vi "Cascade front panel.vi"() -> ()   [LabVIEW 2016]
uses:
  sdi_12/SDI-12/Sonde Vertical Graph.ctl
  controls/Vertical Chart.ctl
  sdi_12/Groundwater header.ctl
  controls/MCC DAQ Setup.ctl
  controls/Aux Sensor.ctl
  KPRO_2016 subvis/Control 2.ctl
  KPRO_2016 subvis/Graph Controls 2.ctl
  KPRO_2016 subvis/Ik control.ctl
  controls/MCC DAQ Readings.ctl
  controls/Kpro pressure measurement cluster.ctl
  controls/Kpro hydraulic measurement cluster.ctl
  activeXtest/activeXtest 2015 Folder/sonde cluster from excel.ctl
  sdi_12/Sonde Value Percent Tol.ctl
  activeXtest/activeXtest 2015 Folder/sample data row cluster.ctl
  activeXtest/activeXtest 2015 Folder/sonde cluster.ctl
  KPRO_2016 subvis/Sensor Physical Measurements.ctl
  KPRO_2016 subvis/SS Control 7.ctl
  <vilib>/Utility/NIReport.llb/NI_report.lvclass
  controls/Action Control 1.ctl
  <extravilib>/ChannelInstances/One Element Stream-t'Action Control 1.ctl'/Instantiate.vi
  <extravilib>/ChannelInstances/One Element Stream-t'Action Control 1.ctl'/Endpoint.vi
  KPRO_2016 subvis/Kpro Globals.vi
  <vilib>/Utility/file.llb/Write Delimited Spreadsheet (string).vi
  <userlib>/_OpenG.lib/file/file.llb/Strip Path - Traditional__ogtk.vi
  <userlib>/_OpenG.lib/file/file.llb/Build Path - Traditional__ogtk.vi
  <vilib>/Utility/file.llb/Write Delimited Spreadsheet (DBL).vi
  <userlib>/_OpenG.lib/file/file.llb/Strip Path Extension - Path__ogtk.vi
  <userlib>/_OpenG.lib/file/file.llb/Convert File Extension (String)__ogtk.vi
  <vilib>/ULx/Create Channel.llb/ULx Create Channel (AI-Voltage-Basic).vi
  KPRO_2016 subvis/Global_SIM_switch.vi
  C:/Program Files (x86)/National Instruments/LabVIEW 2016/vi.lib/ULx/ULx_LV.dll
  Program Files (x86)/National Instruments/LabVIEW 2016/vi.lib/ULx/ULx_LV.dll
  <vilib>/Utility/config.llb/NI_LVConfig.lvlib
  <extravilib>/ChannelInstances/One Element Stream-t'Action Control 1.ctl'.lvlib
panel:
  in  "Open Excel Files":bool
  in  "Input Variables and Slopes 2":T1={"Total Volume"=0.0, "String Pot Slope"=1.6619999408721924, "Flow Slope"=39.040000915527344, "Up Hole Pressure Slope"=48.27000045776367, "Depth to Water Table"=-0.0, "Atmospheric Pressure"=32.22022530555725, "Reservoir Pressure"=-0.004827000045779073, "Height of Sample Box"=0.0, "DH Pressure Trans Slope"=42.0, "DH Pressure Offset"=0.0, "Up Hole  Pressure Offset"=0.0, "Aux 1 Slope"=1.0, "Aux 2 Slope"=1.0, "Aux 3 Slope"=1.0} {"Aux 3 Slope" format="%.2f"; "Aux 2 Slope" format="%.2f"; "Aux 1 Slope" format="%.2f"; "Up Hole  Pressure Offset" format="%.2f"; "DH Pressure Offset" format="%.2f"; "DH Pressure Trans Slope" format="%.2f"; "Height of Sample Box" format="%.2f"; "Reservoir Pressure" format="%.2f"; "Atmospheric Pressure" format="%.2f"; "Depth to Water Table" format="%.2f"; "Up Hole Pressure Slope" format="%.2f"; "Flow Slope" format="%.2f"; "String Pot Slope" format="%.2f"; "Total Volume" format="%.2f"}
  out "Select Worksheet Index":i32
  out "Number of Sample Sheets":i32
  out "NI_report out":refnum<class "NI_report.lvclass">
  out "Sonde OK":bool
  out "DAQ On":bool
  in  "Finish Tests 2":bool
  out "output cluster":T2 caption="Cluster" {"Salinity" format="%_3g"; "Temp\ndeg C" format="%_2g"; "ORP" format="%_4g"; "pH" format="%_4g"; "Dissolved\nOxygen mg/L" format="%_3g"; "Specific\nCond (mS)" format="%_4g"; "Cumulative\nVolume (ml)" format="%#_4g"}
  out "Serial Number/MISC":string
  in  "Depth mode":bool caption="Use \nIncrement"
  in  "Sample Sheet Data Row Cluster 2":T3={"Head\nPressure"=0.0, "Depth"=0.0, "comment string"="", "Sonde Data Cluster"={"Cumulative\nVolume (ml)"=100.0, "Specific\nCond (mS)"=2.0, "Dissolved\nOxygen mg/L"=3.0, "pH"=4.0, "ORP"=5.0, "Temp\ndeg C"=26.0, "Salinity"=7.0}, "Aux1"=0.0, "Aux2"=0.0, "Aux3"=0.0} {"Sonde Data Cluster"."Salinity" format="%_3g"; "Sonde Data Cluster"."Temp\ndeg C" format="%_2g"; "Sonde Data Cluster"."ORP" format="%_4g"; "Sonde Data Cluster"."pH" format="%_4g"; "Sonde Data Cluster"."Dissolved\nOxygen mg/L" format="%_4g"; "Sonde Data Cluster"."Specific\nCond (mS)" format="%_4g"; "Sonde Data Cluster"."Cumulative\nVolume (ml)" format="%#_4g"; "Depth" format="%#.3g"; "Head\nPressure" format="%#.4g"}
  out "subarray":string[][](array[string])
  out "Initialization":i32
  in  "Increment Depth":bool
  in  "Finish Tests":bool
  in  "Start KPRO":bool
  in  "Record Continuous Samples":bool
  out "Current Time (s)":dbl
  in  "stop":bool
  in  "Write Data to Spreadsheet":bool
  in  "Sample Not Collected":bool
  in  "Record Single Sample":bool
  in  "Tab Control":T4(tab)
  out "12V Voltage Monitor":dbl format="%_3f"
  out "Found Quanta Sonde Com Port":refnum<visa-resource-name>
  in  "Temporary Data Files Directory":path=path "C:/Cascade/Data/Output Files"
  in  "Data File Directory":path=path "C:/Cascade/Data/Excel Reports"
  out "Quanta Sonde found?":bool
  in  "template file path":path=path "C:/Cascade/templates/Groundwater Profiling Log_empty_labview_template.xlsx"
  in  "Config File Path":path=path "C:/Cascade/Data/config files/DAQ Setup Config.ini"
  in  "Read Configuration File?":bool
  out "H-4191 Adapter found":bool
  in  "Save Configuration File?":bool
  out "Sonde Communication Error Out":errorcluster
  in  "Search for Comm Ports?":bool=TRUE
  in  "USB Serial Port Manual Entry":refnum<visa-resource-name>="COM13"
  in  "Sonde Parameters \nTolerance Limits":T5 {"Salinity %" format="%_2f%%"; "Temp %" format="%_2f%%"; "ORP %" format="%_2f%%"; "pH %" format="%_2f%%"; "DO %" format="%_2f%%"; "SC %" format="%_2f%%"}
  in  "Sonde Parameters \nInitial Values":T6 {"Salinity Initial" format="%_2f"; "Temp Initial" format="%_2f"; "ORP  Initial" format="%_2f"; "pH Initial" format="%_2f"; "DO Initial" format="%_2f"; "SC Initial" format="%_2f"}
  in  "Header path":path=path "C:/Cascade/templates/Fields for Excel sheets.xlsx"
  out "Sensor  Real \nMeasurements":T7 {"9V Monitor" format="%#.3g"; "Aux 3" format="%#.3g"; "Aux 2" format="%#.3g"; "Aux 1" format="%#.3g"; "String Pot" format="%#.3g"; "Top String Pot" format="%#_4g"; "Downhole Pressure" format="%#_4g"; "Flow" format="%#_4g"; "Uphole Pressure" format="%#_4g"}
  in  "MCC USB-DAQ Setup":T8={"Device Name in InstaCal"="Dev0", "Omega Pressure Sensor"={"DAQ Channel"=2.0, "Output Voltage Range"=1, "Enabled"=TRUE, "Description"="Uphole Pressure"}, "McMillian 102 Flowmeter"={"DAQ Channel"=11.0, "Output Voltage Range"=0, "Enabled"=TRUE, "Description"="Flow"}, "DHT Pressure Sensor"={"DAQ Channel"=3.0, "Output Voltage Range"=1, "Enabled"=TRUE, "Description"="Downhole Pressure"}, "Top String Pot"={"DAQ Channel"=0.0, "Output Voltage Range"=0, "Enabled"=TRUE, "Description"="Top String Pot"}, "String Pot Signal"={"DAQ Channel"=1.0, "Output Voltage Range"=0, "Enabled"=TRUE, "Description"="String Pot"}, "Aux Sensor 1"={"DAQ Channel"=5.0, "Output Voltage Range"=1, "Enabled"=TRUE, "Description"="Aux 1"}, "Aux Sensor 2"={"DAQ Channel"=6.0, "Output Voltage Range"=1, "Enabled"=TRUE, "Description"="Aux 2"}, "Aux Sensor 3"={"DAQ Channel"=7.0, "Output Voltage Range"=1, "Enabled"=TRUE, "Description"="Aux 3"}, "Voltage Monitor"={"DAQ Channel"=8.0, "Output Voltage Range"=0, "Enabled"=TRUE, "Description"="9V Monitor"}} {"Voltage Monitor"."Output Voltage Range" items=["+/-10 V Range", "+/-5 V Range", "+/-2.5V Range", "+/-1.25 V Range", "+/-0.625 V Range", "+/-0.3125 V Range", "+/-0.1562V Range", "+/-0.078125 V Range"]; "Aux Sensor 3"."Output Voltage Range" items=["+/-10 V Range", "+/-5 V Range", "+/-2.5V Range", "+/-1.25 V Range", "+/-0.625 V Range", "+/-0.3125 V Range", "+/-0.1562V Range", "+/-0.078125 V Range"]; "Aux Sensor 2"."Output Voltage Range" items=["+/-10 V Range", "+/-5 V Range", "+/-2.5V Range", "+/-1.25 V Range", "+/-0.625 V Range", "+/-0.3125 V Range", "+/-0.1562V Range", "+/-0.078125 V Range"]; "Aux Sensor 1"."Output Voltage Range" items=["+/-10 V Range", "+/-5 V Range", "+/-2.5V Range", "+/-1.25 V Range", "+/-0.625 V Range", "+/-0.3125 V Range", "+/-0.1562V Range", "+/-0.078125 V Range"]; "String Pot Signal"."Output Voltage Range" items=["+/-10 V Range", "+/-5 V Range", "+/-2.5V Range", "+/-1.25 V Range", "+/-0.625 V Range", "+/-0.3125 V Range", "+/-0.1562V Range", "+/-0.078125 V Range"]; "Top String Pot"."Output Voltage Range" items=["+/-10 V Range", "+/-5 V Range", "+/-2.5V Range", "+/-1.25 V Range", "+/-0.625 V Range", "+/-0.3125 V Range", "+/-0.1562V Range", "+/-0.078125 V Range"]; "DHT Pressure Sensor"."Output Voltage Range" items=["+/-10 V Range", "+/-5 V Range", "+/-2.5V Range", "+/-1.25 V Range", "+/-0.625 V Range", "+/-0.3125 V Range", "+/-0.1562V Range", "+/-0.078125 V Range"]; "McMillian 102 Flowmeter"."Output Voltage Range" items=["+/-10 V Range", "+/-5 V Range", "+/-2.5V Range", "+/-1.25 V Range", "+/-0.625 V Range", "+/-0.3125 V Range", "+/-0.1562V Range", "+/-0.078125 V Range"]; "Omega Pressure Sensor"."Output Voltage Range" items=["+/-10 V Range", "+/-5 V Range", "+/-2.5V Range", "+/-1.25 V Range", "+/-0.625 V Range", "+/-0.3125 V Range", "+/-0.1562V Range", "+/-0.078125 V Range"]}
  out "Rate":dbl=1000.0 caption="Sample Rate (Hz)"
  out "Number \nof Channels":u16
  in  "Channel \nData Rate S/s":dbl=3720.0 format="%#_13g"
  out "Descriptions":string[](array[string])
  out "Raw Voltages":dbl[](array[numeric])
  out "9V Voltage Monitor":dbl format="%#_3g"
  in  "Record DAQ Raw Voltages":bool
  out "Sensor Voltage Cluster":T10 {"9V Monitor" format="%#.3g"; "Aux 3" format="%#_3g"; "Aux 2" format="%#.3g"; "Aux 1" format="%#.3g"; "String Pot" format="%#.3g"; "Top String Pot" format="%#_3g"; "Downhole Pressure" format="%#.3g"; "Flow" format="%#_3g"; "Uphole Pressure" format="%-#1.3g"}
  in  "Clear Groundwater Header Values":bool
  in  "Groundwater Header":T11
  in  "Excel report file path":path=path "C:/Cascade/Data/Excel Reports/Groundwater Profiling Log_ara1.xlsx"
  out "Data Setup Indicator":string
  in  "Start Initialization":bool
  in  "Input Variables and Slopes":T1={"Total Volume"=0.0, "String Pot Slope"=1.6619999408721924, "Flow Slope"=39.040000915527344, "Up Hole Pressure Slope"=48.27000045776367, "Depth to Water Table"=-0.0, "Atmospheric Pressure"=32.22022530555725, "Reservoir Pressure"=-0.004827000045779073, "Height of Sample Box"=0.0, "DH Pressure Trans Slope"=42.0, "DH Pressure Offset"=0.0, "Up Hole  Pressure Offset"=0.0, "Aux 1 Slope"=1.0, "Aux 2 Slope"=1.0, "Aux 3 Slope"=1.0} {"Aux 3 Slope" format="%.2f"; "Aux 2 Slope" format="%.2f"; "Aux 1 Slope" format="%.2f"; "Up Hole  Pressure Offset" format="%.2f"; "DH Pressure Offset" format="%.2f"; "DH Pressure Trans Slope" format="%.2f"; "Height of Sample Box" format="%.2f"; "Reservoir Pressure" format="%.2f"; "Atmospheric Pressure" format="%.2f"; "Depth to Water Table" format="%.2f"; "Up Hole Pressure Slope" format="%.2f"; "Flow Slope" format="%.2f"; "String Pot Slope" format="%.2f"; "Total Volume" format="%.2f"}
  out "Pressure Offset":dbl
  out "appended path":path
  out "Down hole Pressure Transducer CSV data  path 2":path
  in  "Static IK path":path=path "C:/Cascade/Data/Output Files/Static Ik.csv"
  in  "Slopes File Path":path=path "C:/Cascade/Data/Output Files/slopes.csv"
  out "Output File Path":path=path "C:/KPRO_2010/Output_files/Static Ik.txt"
  out "KPRO SessionOutput File Path":path=path "C:/KPRO_2010/Output_files/Static Ik.txt"
  in  "Slopes History File Path":path=path "C:/Cascade/Data/Output Files/slopes.csv"
  out "Sonde Recording Error file":path
  out "IK Recording Error file":path
  out "Sonde Output File Path":path=path "C:/KPRO_2010/Output_files/Static Ik.txt"
  out "KPRO Cumulative Output File Path":path=path "C:/Cascade/Data/Output Files/Output_files"
  in  "Update Sonde":bool
  out "Sonde Data Array":T12[](array[typedef]) {"Salinity"."%" format="%_2f%%"; "Salinity"."Value" format="%_4g"; "Temperature"."%" format="%_2f%%"; "Temperature"."Value" format="%_4g"; "ORP"."%" format="%_2f%%"; "ORP"."Value" format="%_4g"; "pH"."%" format="%_2f%%"; "pH"."Value" format="%_4g"; "Dissolved Oxygen"."%" format="%_2f%%"; "Dissolved Oxygen"."Value" format="%_4g"; "Sp. Conductance"."%" format="%_2f%%"; "Sp. Conductance"."Value" format="%_4g"; "Cumulative\nVolume" format="%#_4g"}
  out "Table Label":string="Data from Sample Sheet %d from Excel File"
  out "Sonde Data Display":T14
  out "Temperature":cluster{"Y":dbl[], "Y":dbl[]}[](graph)
  in  "Record  Sonde Reason":bool
  in  "Select Reasons to Record Data":u16(ring) items=["Per Client Request", "Timed Out", "Sample stopped flowing", "Equipment Issue"]
  out "Sonde Recording Failure Path":path
  out "Sonde IK Behavior Path":path
  out "Recording Reason Sonde array":string[][](array[string])
  out "IK Reason array":string[][](array[string])
  out "SC  Reference\nCalibrate Response":bool
  out "DO  Reference\nCalibrate Response":bool
  in  "Salinity \nReference":dbl
  out "Salinity  Reference\nCalibrate Response":bool
  out "ORP  Reference\nCalibrate Response":bool
  in  "SC \nReference":dbl
  in  "DO \nReference":dbl
  in  "ORP Reference":dbl
  in  "pH Reference":dbl
  in  "pH Zero":dbl
  in  "Record  SC Calibration":bool
  in  "Record DO Calibration":bool
  in  "Record Salinity Calibration":bool
  in  "Record ORP Calibration":bool
  in  "Record pH Calibration Reference":bool
  in  "Record pH Calibration Zero":bool
  out "pH Zero \nCalibrate Response":bool
  out "pH  Reference\nCalibrate Response":bool
  out "KPRO Finish\nIndicator":bool
  in  "Input Depths \nand Parameters Cluster":T16={"Flow"=0.21081600494384767, "Zeroed \nPressure"=74.74207969932556, "Ik"=0.003788962123473114, "Current Depth"=-100.6, "Feet of Stainless"=40, "Start Depth"=0.0, "Abs Start Depth"=0.0} {"Abs Start Depth" format="%.2f"; "Start Depth" format="%.2f"; "Current Depth" format="%.2f"; "Ik" format="%.2f"; "Zeroed \nPressure" format="%.2f"; "Flow" format="%.2f"}
  out "Zero Pressure\nIndicator":bool
  in  "Zero\nPressure":bool caption="Zero Pressure"
  in  "enable_IKMGS_file":bool
  in  "enable_slug_file":bool
  in  "enable_kpro_file":bool=TRUE
  in  "Simulate AD6B":bool
  out "KPRO Test\nIndicator":bool
  in  "Record DTW File":bool
  in  "Zero In-Line Pressure\n(F = leave as is)":bool=TRUE
  out "Current Session":sgl[][](array[numeric]) format="%.2f"
  in  "KPRO test report header":string[](array[string])=["Time(msecs)", "Uncorrected Depth", "Corrected Depth", "Drive_Rate", "Flow", "Feet_of Stainless", "Up Hole Pressure", "IK", "Corrected Pressure", "Atm Pressure", "Depth to water", "Height of box", "Res_Pressure", "Secs_since_1_JAN_1904", "Depth jumps more than 1_foot", "Down hole Pressure"]
  in  "Depth Cluster":T17
  out "Cumulative_data_from_file":sgl[][](array[numeric]) format="%.2f"
  in  "KPRO test report header 2":string[](array[string])=["Time(msecs)", "Uncorrected Depth", "Corrected Depth", "Drive_Rate", "Flow", "Feet_of Stainless", "Up Hole Pressure", "IK", "Corrected Pressure", "Atm Pressure", "Depth to water", "Height of box", "Res_Pressure", "Secs_since_1_JAN_1904", "Depth jumps more than 1_foot", "Down hole Pressure"]
  out "Cumulative_data_ready":bool
  out "Depth Rate\nft/min":dbl format="%#.2g"
  out "Ik":dbl=0.003788962123473114 caption="Real Time - Depth vs. lk" format="%.2f"
  out "Uphole Pressure":dbl format="%.2f"
  in  "New Depth":dbl
  in  "Update Depth":bool
  in  "Select Entry for IK Log File":u16(ring) items=["IK Increase", "IK stayed the Same", "IK decreased"]
  out "Large Depth IK Graph Cluster":T18={[0.003788962123473114, 0.0037174584307500765, 0.0037174584307500765, 0.0037174584307500765, 0.0037174584307500765, 0.003788962123473114], [-100.1, -100.2, -100.3, -100.4, -100.5, -100.6]}
  in  "Culmulative Graph Cluster":T19={"Cumulative - Depth vs. Ik"={[], []}, "Real Time - Depth vs. lk "={[0.003788962123473114, 0.0037174584307500765, 0.0037174584307500765, 0.0037174584307500765, 0.0037174584307500765, 0.003788962123473114], [-100.1, -100.2, -100.3, -100.4, -100.5, -100.6]}, "Cumulative - Depth vs. Drive Rate"={[], []}, "Real Time - Depth vs. Drive Rate"={[0.02036245163917736, 0.125, 0.16666666666666674, 0.16666666666666663, 0.16666666666666663, 0.16666666666666663], [-100.1, -100.2, -100.3, -100.4, -100.5, -100.6]}}
  out "Down hole Pressure":dbl format="%.2f"
  in  "Record IK Reason":bool
  in  "Corrected Pressure Cluster":T20
  out "Flow":dbl format="%#.2g"
  out "Current Depth":sgl=-100.6 format="%.2f"
  out "Current \nDepth (m)":sgl=-30.661383 format="%.2f"
  in  "Read String Pot":bool
  out "Large Depth IK Graph":dbl(graph)
  out "DAQ Error":errorcluster
  out "Initialization Finished":bool=TRUE
  out "Stop":bool
  out "error out":errorcluster
  in  "error in (no error)":errorcluster
  out "producer loop":i32
  out "consumer loop":i32
  out "Active Channel Array":string[](array[string])
  out "delimited string":string
  out "Voltage Range":dbl[](array[numeric])
  out "Stop 2":bool
  out "column max value":i32
  out "Current Sample Sheet":string="Sample 1"
  out "last occupied cell's name":string
  out "row max value":i32
  in  "Current Sheet":i32=1
  out "Worksheet Names":string[](array[string])
  # "ft. water"
  # "mL/min."
  # "ft. water"
  # "ft."
  # "ft."
  # "Instructions for Sonde Calibration:\n1.  Use the Record Single Point to Record the Data prior to start of\ncalibration procedure to record the initial points to the excel worksheet.\n2.  pH Calibration is a 2 step process:  A pH standard between 6.8 and 7.2 is treated as the “zero”\nand all other values are treated as the “slope”. First calibrate “zero”, then  add a second to calibrate “slope”. \n3.  Specific Conductance:  Wait for the specific conductance readings to stabilize in the calibration solution, which may\nrequire one or two minutes."
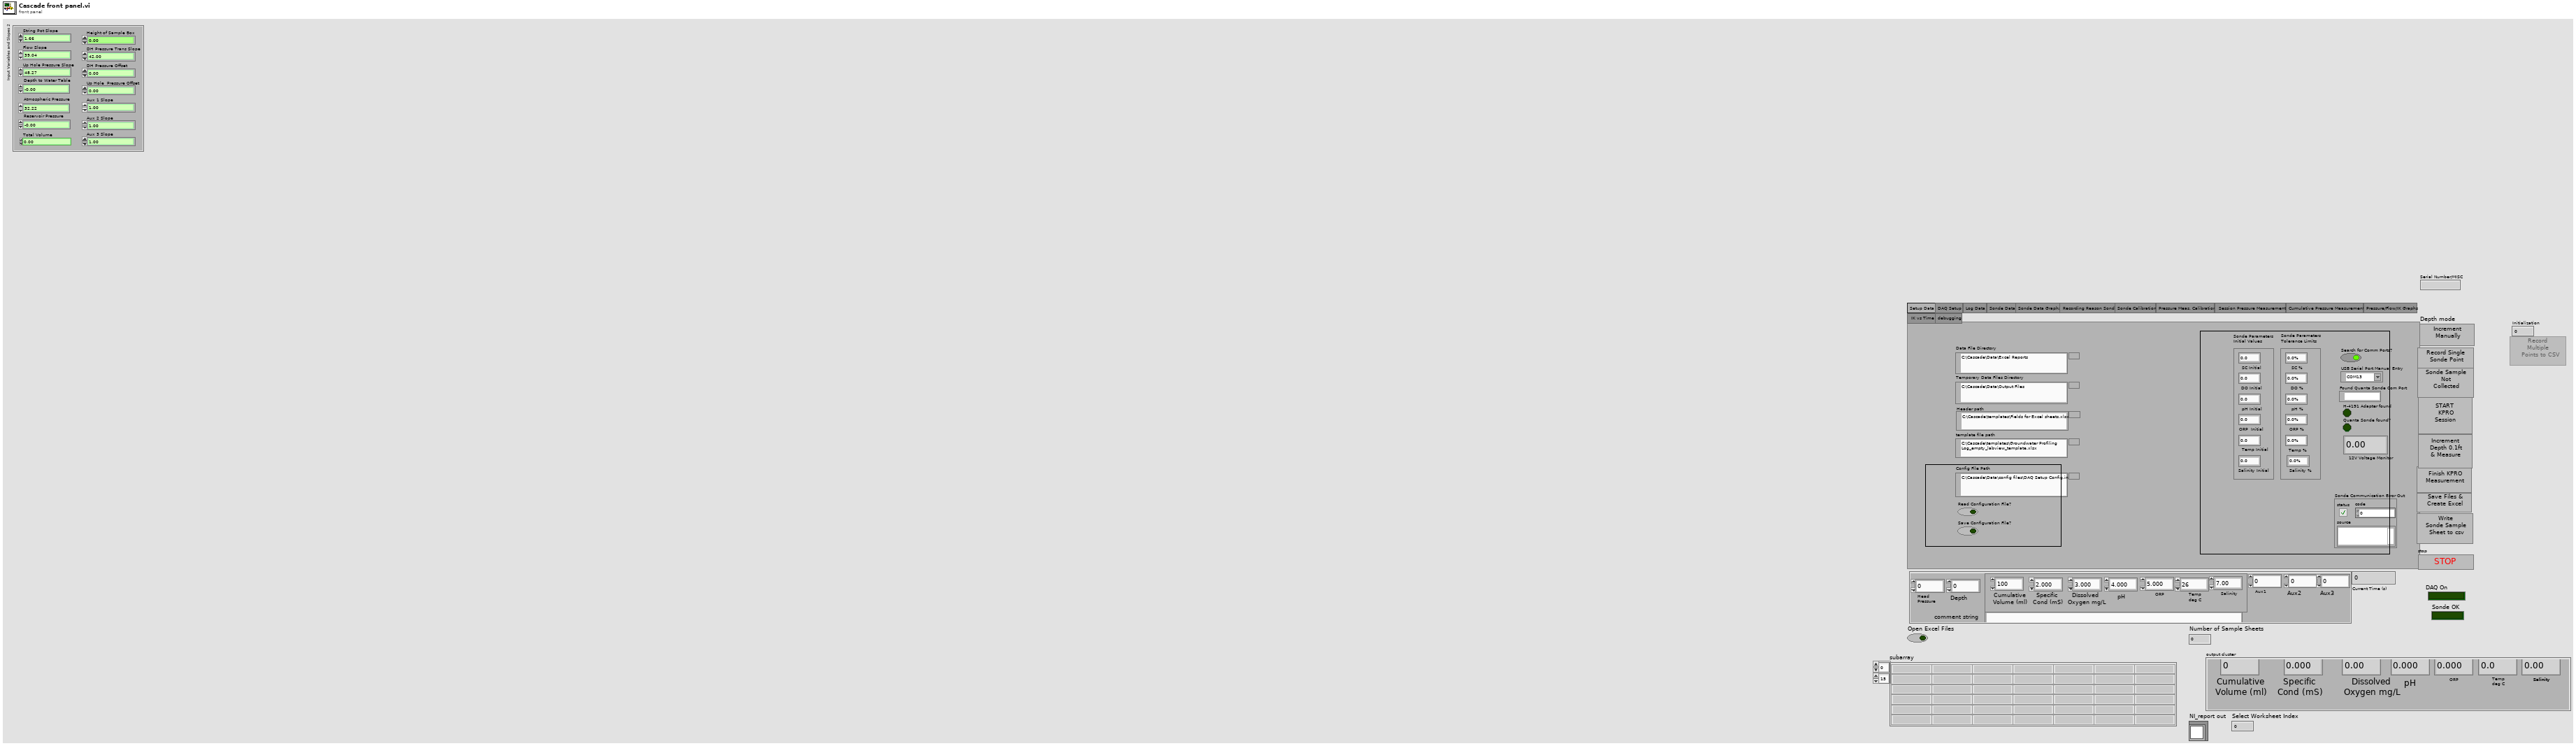
[diagram p1: front panel]
types:
  T1 = typedef "Control 2.ctl" = cluster{"Total Volume":dbl, "String Pot Slope":dbl, "Flow Slope":dbl, "Up Hole Pressure Slope":dbl, "Depth to Water Table":dbl, "Atmospheric Pressure":dbl, "Reservoir Pressure":dbl, "Height of Sample Box":dbl, "DH Pressure Trans Slope":dbl, "DH Pressure Offset":dbl, "Up Hole  Pressure Offset":dbl, "Aux 1 Slope":dbl, "Aux 2 Slope":dbl, "Aux 3 Slope":dbl}
  T2 = typedef "sonde cluster.ctl" = cluster{"Cumulative\nVolume (ml)":dbl, "Specific\nCond (mS)":dbl, "Dissolved\nOxygen mg/L":dbl, "pH":dbl, "ORP":dbl, "Temp\ndeg C":dbl, "Salinity":dbl}
  T3 = typedef "sample data row cluster.ctl" = cluster{"Head\nPressure":dbl, "Depth":dbl, "comment string":string, "Sonde Data Cluster":T2, "Aux1":dbl, "Aux2":dbl, "Aux3":dbl}
  T4 = enum32{"Setup Data", "DAQ Setup", "Log Data", "Sonde Data", "Sonde Data Graphs", "Recording Reason Sonde", "Sonde Calibration", "Pressure Meas. Calibration", " Session Pressure Measurements", "Cumulative Pressure Measurements", "Pressure/Flow/IK Graphs", "IK vs Time ", "debugging"}
  T5 = cluster{"SC %":dbl, "DO %":dbl, "pH % ":dbl, "ORP % ":dbl, "Temp % ":dbl, "Salinity %":dbl}
  T6 = cluster{"SC Initial ":dbl, "DO Initial ":dbl, "pH Initial  ":dbl, "ORP  Initial":dbl, "Temp Initial":dbl, "Salinity Initial ":dbl}
  T7 = typedef "Sensor Physical Measurements.ctl" = cluster{"Uphole Pressure":dbl, "Flow":dbl, "Downhole Pressure":dbl, "Top String Pot":dbl, "String Pot":dbl, "Aux 1":dbl, "Aux 2":dbl, "Aux 3":dbl, "9V Monitor":dbl}
  T8 = typedef "MCC DAQ Setup.ctl" = cluster{"Device Name in InstaCal":string, "Omega Pressure Sensor":T9, "McMillian 102 Flowmeter":T9, "DHT Pressure Sensor":T9, "Top String Pot":T9, "String Pot Signal":T9, "Aux Sensor 1":T9, "Aux Sensor 2":T9, "Aux Sensor 3":T9, "Voltage Monitor":T9}
  T9 = typedef "Aux Sensor.ctl" = cluster{"DAQ Channel":dbl, "Output Voltage Range":u16, "Enabled":bool, "Description":string}
  T10 = typedef "MCC DAQ Readings.ctl" = cluster{"Uphole Pressure":dbl, "Flow":dbl, "Downhole Pressure":dbl, "Top String Pot":dbl, "String Pot":dbl, "Aux 1":dbl, "Aux 2":dbl, "Aux 3":dbl, "9V Monitor":dbl}
  T11 = typedef "Groundwater header.ctl" = cluster{"Location":string, "Date Finished":string, "CTS":string, "sampler":string, "Kpro box Serial ":string, "Sonde Serial":string, "Drilling Contractor":string, "Ave Depth to Water":string, "Gas/Peri Pump":string, "Atmospheric Pressure":string, "KPRO N2 Pressure":string, "Gas Drive N2 Pressure":string, "Profile ID":string}
  T12 = typedef "sonde cluster from excel.ctl" = cluster{"Head":dbl, "Depth":dbl, "Time":string, "Cumulative\nVolume":dbl, "Sp. Conductance":T13, "Dissolved Oxygen":T13, "pH":T13, "ORP":T13, "Temperature":T13, "Salinity":T13, "Final Tol.":bool, "Final":bool, "Time 2":timestamp, "Aux 1":dbl, "Aux 2":dbl, "Aux 3":dbl}
  T13 = typedef "Sonde Value Percent Tol.ctl" = cluster{"Value":dbl, "%":dbl, "Tol.":bool}
  T14 = typedef "Sonde Vertical Graph.ctl" = cluster{"pH":T15, "Conductance":T15, "Salinity":T15, "DO % Saturation":T15, "DO mg/L":T15, "ORP":T15}
  T15 = typedef "Vertical Chart.ctl" = cluster{"Y":dbl[], "Y":dbl[]}[]
  T16 = typedef "SS Control 7.ctl" = cluster{"Flow":dbl, "Zeroed \nPressure":dbl, "Ik":dbl, "Current Depth":sgl, "Feet of Stainless":i32, "Start Depth":sgl, "Abs Start Depth":sgl}
  T17 = typedef "Kpro hydraulic measurement cluster.ctl" = cluster{"Absolute Depth In":dbl, "Current Absolute Depth":dbl, "First Absolute Depth":dbl, "Previous Relative Depth":dbl, "Current Relative Depth":dbl, "First Relative Depth":dbl, "Last Filed Depth":dbl, "Total Volume In":dbl, "Total Volume Out":dbl, "Current Measurement Time":dbl, "Previous Measurement Time":dbl}
  T18 = typedef "Ik control.ctl" = cluster{dbl[], dbl[]}
  T19 = typedef "Graph Controls 2.ctl" = cluster{"Cumulative - Depth vs. Ik":cluster{dbl[], dbl[]}, "Real Time - Depth vs. lk ":cluster{dbl[], dbl[]}, "Cumulative - Depth vs. Drive Rate":cluster{dbl[], dbl[]}, "Real Time - Depth vs. Drive Rate":cluster{dbl[], dbl[]}}
  T20 = typedef "Kpro pressure measurement cluster.ctl" = cluster{"Up hole Corrected Pressure":dbl, "Down hole Corrected Pressure":dbl}
  T21 = typedef "NI_LVConfig.lvlib/Config Data RefNum.ctl" = refnum<k1>
  T22 = enum8{"Enabled", "Disabled", "Disabled and Grayed Out"}
  T23 = typedef "Action Control 1.ctl" = enum16{"TimeOut", "Continuous  Sonde Data", "Init", "Exit", "Acq. Single Sonde Point", "Write Sonde Sample Sheet", "Acq. DAQ data", "Sample Not Collected", "Record Sonde Reason", "pH Calibration Zero", "pH Calibration Standard", "ORP Calibration Standard", "Salinity Calibration Standard", "DO Calibration Standard", "SC Calibration Standard", "Increment Depth Manually", "Start KPRO Measurements", "Finish KPRO Measurements", "Update Depth", "IK vs Time", "Record IK Reason", "Create Excel Files"}
  T24 = typedef "One Element Stream-t'Action Control 1.ctl'.lvlib/)Channel.ctl" = refnum<queue>
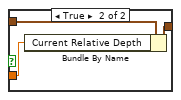
[diagram p13: hidden frame]
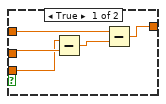
[diagram p14: hidden frame]
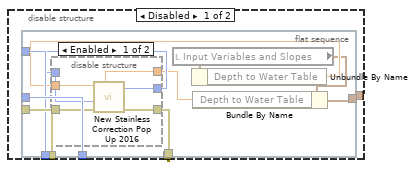
[diagram p20: hidden frame]
diagram:
  # "For calibrate command (XC) on SDI-12 address ‘a’, P is pH, C is specific conductance, S is\nsalinity or TDS, % is DO %Saturation, O is DO mg/L, R is ORP, D is depth, B is\nbarometric pressure, and t is TDS scale factor."
  n1 = flat-sequence {
    tunnel: [w20] -> w5
    tunnel: [w52] -> w7
    tunnel: w5 -> [w52]
    tunnel: [w48] -> w3
    tunnel: [w54] -> w14
    tunnel: w7 -> [w57]
    tunnel: [w57] -> w6
    tunnel: w14 -> [w101]
    tunnel: [w106] -> w12
    tunnel: [w108] -> w11
    tunnel: [w110] -> w8
    tunnel: [w103] -> w9
    tunnel: [w109] -> w10
    tunnel: [w107] -> _
    tunnel: [w98] -> w13
    tunnel: [w104] -> w2
    tunnel: [w105] -> w1
    frame #0 {
      n2 = invoke on="error out" class="Clust (strict)" method="Reinit To Default"(error in="error in (no error)") -> (error out=w18:errorcluster)  [unwired: 2 in, 2 out]
      n3 = flat-sequence {
        tunnel: [w24] -> w20
        tunnel: w18 -> [w23]
        frame #0 {
          n4 = case shown="False" "Read Configuration File?" {
            selector: "Read Configuration File?" -> [_ w31]
            tunnel: [w25 w36] -> w24
            tunnel: w23 -> [w25 w33]
            tunnel: "Config File Path" -> [_ w32]
            frame False {
            }
            frame True {
              n5 = call <vilib>:"Check if File or Folder Exists.vi"("error in (no error)"=w33, "path"=w32) -> ("error out"=w28:errorcluster, "file or folder exists?"=w29:bool, "dup path"=w27:path)  [unwired: 7 in]
              n6 = And(x=w31, y=w29) -> (x .and. y?=w30:bool)
              n7 = control-ref of="This VI"() -> (w34:refnum<vi>)
              n8 = case shown="True" w30 {
                selector: w30 -> [w37 _]
                tunnel: w27 -> [_ w42]
                tunnel: w28 -> [w38 w46]
                tunnel: [w38 w39] -> w35
                tunnel: w34 -> [_ w47]
                frame False {
                  n9 = local write "Read Configuration File?"(w37) -> ()
                }
                frame True {
                  n10 = call <vilib>:"Open Config Data.vi"("error in (no error)"=w46, "create file if necessary (T)"=FALSE, "configuration file path"=w42) -> ("error out"=w44:errorcluster, "refnum"=w45:T21)  [unwired: 6 in, 1 out]
                  n11 = call <userlib>:"Read Panel from INI__ogtk.vi"("error in (no error)"=w44, "VI ref"=w47, "refnum"=w45) -> ("error out"=w40:errorcluster, "refnum out"=w41:T21)  [unwired: 7 in]
                  n12 = call <vilib>:"Close Config Data.vi"("error in (no error)"=w40, "refnum"=w41) -> ("error out"=w39:errorcluster)  [unwired: 8 in, 1 out]
                }
              }
              n13 = call <vilib>:"Clear Errors.vi"("error in (no error)"=w35) -> ("error out"=w26:errorcluster)  [unwired: 5 in, 1 out]
              n14 = Merge Errors(w26) -> (w36:errorcluster)
            }
          }
        }
      }
    }
    frame #1 {
      n15 = invoke on="Current Session" class="Arr (strict)" method="Reinit To Default"() -> ()  [unwired: 3 in, 3 out]
      n16 = control-ref of="Sonde Data Display"() -> ()  [unwired: 1 out]
      n17 = local write "Current Sheet"(1 ("Current Sheet")) -> ()
      n18 = Get Date/Time In Seconds() -> (seconds since 1Jan1904=w48:timestamp)
      n19 = Get Date/Time In Seconds() -> (seconds since 1Jan1904=w49:timestamp)
      n20 = Subtract(x=w48, y=w49) -> (x-y=w50:dbl)
      n21 = To Double Precision Float(number=w50) -> (double precision float=→"Current Time (s)":dbl)
    }
    frame #2 {
      w65 = T22."Enabled" ("Disabled")
      w84 = T22."Disabled and Grayed Out" ("Disabled")
      n22 = invoke on="Current Sheet" class="DigNum (strict)" method="Reinit To Default"(error in=w57) -> (error out=w78:errorcluster)  [unwired: 2 in, 2 out]
      n23 = local write "Initialization Finished"(FALSE ("Initialization Finished")) -> ()
      n24 = invoke on="Sample Not Collected" class="Bool" method="Reinit To Default"(error in=w78) -> (error out=w81:errorcluster)  [unwired: 2 in, 2 out]
      n25 = invoke on="Record Continuous Samples" class="Bool" method="Reinit To Default"(error in=w81) -> (error out=w80:errorcluster)  [unwired: 2 in, 2 out]
      n26 = invoke on="Write Data to Spreadsheet" class="Bool" method="Reinit To Default"(error in=w80) -> (error out=w79:errorcluster)  [unwired: 2 in, 2 out]
      n27 = call "search for Quanta Sonde devices.vi"("VISA resource name"="USB Serial Port Manual Entry", "Search for Comm Ports?"="Search for Comm Ports?", "error in (no error)"=w57) -> ("12V monitor"=w64:dbl, "Com Port with Quanta Sonde devices"=w90:refnum<visa-resource-name>[], "Number of Quanta Sonde devices"=w89:i32, "Serial Number/MISC"=w67:string, "Number of Quanta Sonde devices > 0?"=→"Quanta Sonde found?":bool, "H-4191 Adapter found"=→"H-4191 Adapter found":bool, "Error Out"=w73:errorcluster)  [unwired: 4 in, 2 out]
      "12V Voltage Monitor" <- w64
      "Sonde Communication Error Out" <- w73
      "Serial Number/MISC" <- w67
      n28 = invoke on="Record Single Sample" class="Bool" method="Reinit To Default"(error in=w79) -> (error out=w56:errorcluster)  [unwired: 2 in, 2 out]
      n29 = property on="Record Continuous Samples" class="Bool"(error in=w56, "DisabledEnum"=w84) -> (error out=w85:errorcluster)  [unwired: 1 in, 1 out]
      n30 = local read "Groundwater Header"() -> (w66:T11)
      n31 = Greater Or Equal?(x=w64, y=11.75) -> (x >= y?=→"Sonde OK":bool)
      n32 = case shown="1" w89 {
        tunnel: w90 -> [_ w97]
        tunnel: [refnum<visa-resource-name> refnum ("RS232 Port Out") w95] -> w88
        frame 0, Default {
        }
        frame 1 {
          n33 = Index Array(array=w97, index=0) -> (element=w95:refnum<visa-resource-name>)
        }
      }
      "Found Quanta Sonde Com Port" <- w88
      n34 = property on="Record Single Sample" class="Bool"(error in=w85, "DisabledEnum"=w84) -> (error out=w86:errorcluster)  [unwired: 1 in, 1 out]
      n35 = invoke on="stop" class="Bool" method="Reinit To Default"(error in=w56) -> (error out=w83:errorcluster)  [unwired: 2 in, 2 out]
      n36 = Bundle By Name(cluster=w66, "Sonde Serial"=w67) -> (w68:T11)
      n37 = invoke on="Stop" class="Bool (strict)" method="Reinit To Default"(error in=w56) -> (error out=w75:errorcluster)  [unwired: 2 in, 2 out]
      n38 = property on="Sample Not Collected" class="Bool"(error in=w86, "DisabledEnum"=w84) -> (error out=w82:errorcluster)  [unwired: 1 in, 1 out]
      n39 = local write "Groundwater Header"(w68) -> ()
      n40 = property on="Write Data to Spreadsheet" class="Bool"(error in=w83, "DisabledEnum"=w84) -> (error out=w76:errorcluster)  [unwired: 1 in, 1 out]
      n41 = invoke on="Stop 2" class="Bool (strict)" method="Reinit To Default"(error in=w75) -> (error out=w74:errorcluster)  [unwired: 2 in, 2 out]
      n42 = call <vilib>:"Clear Errors.vi"("error in (no error)"=w73) -> ("error out"=w72:errorcluster)  [unwired: 5 in, 1 out]
      n43 = Merge Errors(w72, w74, w76, w82) -> (w69:errorcluster)
      n44 = flat-sequence {
        tunnel: [w93] -> w61
        tunnel: w69 -> [w93]
        frame #0 {
          n45 = local write "Tab Control"(T4."Log Data" ("Tab Control")) -> ()
        }
      }
      n46 = invoke on="Sonde Data Array" class="Arr (strict)" method="Reinit To Default"(error in=w61) -> (error out=w60:errorcluster)  [unwired: 2 in, 2 out]
      n47 = invoke on="Data Setup Indicator" class="Str" method="Reinit To Default"(error in=w60) -> (error out=w58:errorcluster)  [unwired: 2 in, 2 out]
      n48 = property on="Clear Groundwater Header Values" class="Bool"(error in=w58, "DisabledEnum"=w65) -> (error out=w59:errorcluster)  [unwired: 1 in, 1 out]
      n49 = property on="Start Initialization" class="Bool"(error in=w59, "DisabledEnum"=w65) -> (error out=w55:errorcluster)  [unwired: 1 in, 1 out]
      n50 = invoke on="Clear Groundwater Header Values" class="Bool" method="Reinit To Default"(error in=w55) -> (error out=w54:errorcluster)  [unwired: 2 in, 2 out]
    }
    frame #3 {
      n51 = while {
        tunnel: w101 -> [w116]
        tunnel: [w113] -> w100
        tunnel: [w115] -> _
        i -> [w115]
        stop <- w118 stop-if-true
        n52 = event shown="[3] \"Stop\": Value Change" {
          selector: _ -> [_ _ _ _ _]
          dyn-events: _ -> [_ _ _ _ _]
          timeout: 100 -> [_ _ _ _ _]
          tunnel: [FALSE w126 TRUE ("Stop") w130 _] -> w118
          event Timeout {
            n53 = event-data() -> ()  [unwired: 1 in, 3 out]
          }
          event "Start Initialization": Value Change {
            n54 = event-data() -> ()  [unwired: 1 in, 3 out]
            n55 = case shown="True" "Start Initialization" {
              tunnel: [FALSE ("Stop") TRUE ("Stop")] -> w126
              frame False {
              }
              frame True {
                n56 = invoke on="Data Setup Indicator" class="Str" method="Reinit To Default"() -> ()  [unwired: 3 in, 3 out]
                n57 = invoke on="Start Initialization" class="Bool" method="Reinit To Default"() -> ()  [unwired: 3 in, 3 out]
              }
            }
          }
          event Panel Close? {
            n58 = event-data() -> ()  [unwired: 1 in, 4 out]
            n59 = event-data() -> ()  [unwired: 2 in, 1 out]
          }
          event "Stop": Value Change {
            n60 = event-data() -> ("NewVal"=w131:bool)  [unwired: 1 in, 5 out]
            n61 = case shown="False" w131 {
              selector: w131 -> [w132 w133]
              tunnel: [w132 w133] -> w130
              frame False {
              }
              frame True {
              }
            }
          }
          event "Clear Groundwater Header Values": Value Change {
            n62 = event-data() -> ()  [unwired: 1 in, 6 out]
            n63 = case shown="True" "Clear Groundwater Header Values" {
              frame False {
              }
              frame True {
                n64 = invoke on="Groundwater Header" class="Clust (strict)" method="Reinit To Default"() -> (error out=w135:errorcluster)  [unwired: 3 in, 2 out]
                n65 = flat-sequence {
                  tunnel: w135 -> [_]
                  frame #0 {
                    n66 = local read "Groundwater Header"() -> (w136:T11)
                    n67 = local read "Serial Number/MISC"() -> (w137:string)
                    n68 = Bundle By Name(cluster=w136, "Sonde Serial"=w137) -> (w138:T11)
                    n69 = local write "Groundwater Header"(w138) -> ()
                  }
                }
              }
            }
          }
        }
        n70 = call <userlib>:"Wait (ms)__ogtk.vi"("error in (no error)"=w116, "milliseconds to wait"=u32 100) -> ("error out"=w113:errorcluster)  [unwired: 8 in, 1 out]
        n71 = Quotient & Remainder(x=w115, y=100) -> (floor(x/y)=w111:i32)  [unwired: 1 out]
        n72 = case shown="0" w111 {
          tunnel: w113 -> [w121 w123]
          frame 1, Default {
            n73 = property on="Data Setup Indicator" class="Str"(error in=w121, "Text.TextColor"=u32 0) -> ()  [unwired: 1 in, 2 out]
          }
          frame 0 {
            n74 = property on="Data Setup Indicator" class="Str"(error in=w123, "Text.TextColor"=u32 16716800) -> ()  [unwired: 1 in, 2 out]
          }
        }
        "Data Setup Indicator" <- "Hit the Start Key after Data Entry of Log Parameters and File Names." ("Data Setup Indicator")
      }
      n75 = flat-sequence {
        tunnel: w100 -> [w156]
        tunnel: [w154] -> w110
        tunnel: [w153] -> w109
        tunnel: [w140] -> w108
        tunnel: [w151] -> w107
        tunnel: [w150] -> w106
        tunnel: [w149] -> w102
        tunnel: [w147] -> w103
        frame #0 {
          n76 = control-ref of="last occupied cell's name"() -> (w146:refnum<vi>)
          n77 = control-ref of="Current Sample Sheet"() -> (w144:refnum<vi>)
          n78 = control-ref of="row max value"() -> (w145:refnum<vi>)
          n79 = call "setup excel worksheet.vi"("Last Occupied cell Name reference"=w146, "Row Max Value Reference"=w145, "Current Sample Sheet Reference"=w144, "template file path"="template file path", "Excel report file path"="Excel report file path", "error in (no error)"=w156, "Header path"="Header path", "Open Excel Files"="Open Excel Files") -> ("subarray"=→"subarray":string[][], "column max value"=→"column max value":i32, "row max value"=→"row max value":i32, "Column of Volume"=w147:i32, "Worksheet Names"=w140:string[], "NI_report out"=w150:refnum<class "NI_report.lvclass">, "Columns"=w153:i32[], "Number of Sample Sheets"=w154:i32, "Select Worksheet Index"=w151:i32, "error out"=w149:errorcluster)  [unwired: 2 in]
          "Worksheet Names" <- w140
          "NI_report out" <- w150
          "Number of Sample Sheets" <- w154
          "Select Worksheet Index" <- w151
        }
      }
      n80 = flat-sequence {
        tunnel: w102 -> [w163]
        tunnel: [w157] -> w99
        frame #0 {
          w164 = T22."Disabled and Grayed Out" ("Disabled")
          n81 = local write "KPRO Finish\nIndicator"(FALSE ("KPRO Finish\nIndicator")) -> ()
          n82 = invoke on="Start KPRO" class="Bool" method="Reinit To Default"(error in=w163) -> (error out=w162:errorcluster)  [unwired: 2 in, 2 out]
          n83 = invoke on="Finish Tests" class="Bool" method="Reinit To Default"(error in=w162) -> (error out=w161:errorcluster)  [unwired: 2 in, 2 out]
          n84 = invoke on="Increment Depth" class="Bool" method="Reinit To Default"(error in=w161) -> (error out=w160:errorcluster)  [unwired: 2 in, 2 out]
          n85 = property on="Clear Groundwater Header Values" class="Bool"(error in=w160, "DisabledEnum"=w164) -> (error out=w159:errorcluster)  [unwired: 1 in, 1 out]
          n86 = property on="Start Initialization" class="Bool"(error in=w159, "DisabledEnum"=w164) -> (error out=w158:errorcluster)  [unwired: 1 in, 1 out]
          n87 = invoke on="Update Sonde" class="Bool (strict)" method="Reinit To Default"(error in=w158) -> (error out=w157:errorcluster)  [unwired: 2 in, 2 out]
        }
      }
      n88 = flat-sequence {
        tunnel: [w167] -> w105
        tunnel: [w167] -> w104
        tunnel: [w172] -> w98
        tunnel: w99 -> [w171]
        frame #0 {
          n89 = Unbundle By Name("Input Variables and Slopes") -> ("Depth to Water Table"=w177:dbl)
          n90 = local read "Input Depths \nand Parameters Cluster"() -> (w169:T16)
          n91 = Bundle By Name(cluster="Input Variables and Slopes", "Depth to Water Table"=w177) -> (w174:T1)
          n92 = call <vilib>:"Check if File or Folder Exists.vi"("error in (no error)"=w171, "path"="Slopes File Path") -> ("error out"=w170:errorcluster, "file or folder exists?"=w166:bool, "dup path"=w175:path)  [unwired: 7 in]
          n93 = case shown="True" w166 {
            tunnel: w175 -> [_ w193]
            tunnel: w174 -> [w181 w192]
            tunnel: [w181 w191] -> w173
            tunnel: w170 -> [w180 w187]
            tunnel: [w180 w187] -> w172
            frame False {
              n94 = local write "Data Setup Indicator"("Slope file not found." ("Data Setup Indicator")) -> ()
            }
            frame True {
              n95 = call "Get_SLOPE_data_from_file 2016.vi"("Slopes File Path"=w193) -> ("Last Aux 1 Slope"=w186:dbl, "Last_String_Pot_Slope"=w190:dbl, "DHT Offset"=w182:dbl, "DHT Slope"=w183:dbl, "Last_Flow_Slope"=w189:dbl, "Last Aux 2 Slope"=w185:dbl, "Last Aux 3 Slope"=w184:dbl, "Last_Pressure_Slope"=w188:dbl)  [unwired: 6 in, 1 out]
              n96 = Bundle By Name(cluster=w192, "String Pot Slope"=w190, "Flow Slope"=w189, "Up Hole Pressure Slope"=w188, "Aux 1 Slope"=w186, "Aux 2 Slope"=w185, "Aux 3 Slope"=w184, "DH Pressure Trans Slope"=w183, "DH Pressure Offset"=w182) -> (w191:T1)
            }
          }
          n97 = Unbundle By Name(w169) -> ("Feet of Stainless"=w167:i32)
          n98 = Bundle By Name(cluster=w169, "Feet of Stainless"=w167) -> (w168:T16)
          n99 = local write "Input Depths \nand Parameters Cluster"(w168) -> ()
          n100 = local write "Input Variables and Slopes"(w173) -> ()
        }
      }
    }
  }
  n101 = flat-sequence {
    tunnel: [w197] -> w17
    tunnel: w13 -> [w196]
    tunnel: [w195] -> w4
    frame #0 {
      w194 = Action_Control_1."Init"  # Event
      n102 = while {
        shift-right: [w205] -> w197
        shift-left: w196 -> [w205]
        shift-right: [w200] -> _
        shift-left: w194 -> [w198]
        tunnel: [w206] -> w195
        i -> [w204]
        stop <- w202 stop-if-true
        # "User Interface Producer Loop"
        n103 = First Call?() -> (First Call?: T/F=w199:bool)
        n104 = case shown="False" w199 {
          tunnel: w205 -> [w211 _]
          tunnel: [w209 FALSE ("Boolean")] -> w202
          tunnel: [w208 w396] -> w200
          tunnel: w198 -> [_ w396]
          frame False {
            w207 = Action_Control_1."TimeOut"  # Event
            n105 = event shown="[3] \"Record pH Calibration Zero\": Value Change" {
              selector: _ -> [_ _ _ _ _ _ _ _ _ _ _ _ _ _ _ _ _ _ _]
              dyn-events: _ -> [_ _ _ _ _ _ _ _ _ _ _ _ _ _ _ _ _ _ _]
              timeout: 100 -> [_ _ _ _ _ _ _ _ _ _ _ _ _ _ _ _ _ _ _]
              tunnel: [w212 w218 w224 w237 w249 w261 w273 w285 w297 w309 w322 w333 w343 w351 w359 w367 w376 w384 _] -> w208
              tunnel: [FALSE w217 w225 w238 w250 w262 w274 w286 w298 w310 w321 w332 w344 w352 w360 w368 w377 w385 _] -> w209
              tunnel: w211 -> [_ w215 w227 w240 w252 w264 w276 w288 w300 w312 _ w329 _ _ _ _ _ _ _]
              tunnel: [_ w215 w226 w239 w251 w263 w275 w287 w299 w311 _ _ _ _ _ _ _ _ _] -> _
              tunnel: w207 -> [w212 w214 w223 w236 w248 w260 w272 w284 w296 w308 w320 w327 w341 w349 w358 w366 w375 w383 _]
              event Timeout {
                n106 = event-data() -> ()  [unwired: 1 in, 3 out]
              }
              event "stop": Value Change {
                n107 = event-data() -> ()  [unwired: 1 in, 6 out]
                n108 = case shown="False" "stop" {
                  tunnel: [w219 w221] -> w218
                  tunnel: [FALSE TRUE] -> w217
                  tunnel: w214 -> [w219 _]
                  frame False {
                  }
                  frame True {
                    w221 = Action_Control_1."Exit"  # Event
                  }
                }
              }
              event "Record DAQ Raw Voltages": Value Change {
                n109 = event-data() -> ()  [unwired: 1 in, 6 out]
                n110 = case shown="False" "Record DAQ Raw Voltages" {
                  tunnel: [w229 w232] -> w224
                  tunnel: [FALSE FALSE ("Boolean")] -> w225
                  tunnel: [w230 w233] -> w226
                  tunnel: w227 -> [w230 w233]
                  tunnel: w223 -> [w229 _]
                  frame False {
                  }
                  frame True {
                    w232 = Action_Control_1."Acq. DAQ data"  # Event
                  }
                }
              }
              event "Record pH Calibration Zero": Value Change {
                n111 = event-data() -> ()  [unwired: 1 in, 6 out]
                n112 = case shown="True" "Record pH Calibration Zero" {
                  tunnel: [w241 w244] -> w237
                  tunnel: [FALSE FALSE ("Boolean")] -> w238
                  tunnel: [w242 w245] -> w239
                  tunnel: w240 -> [w242 w245]
                  tunnel: w236 -> [w241 _]
                  frame False {
                  }
                  frame True {
                    w244 = Action_Control_1."pH Calibration Zero"  # Event
                  }
                }
              }
              event "Record pH Calibration Reference": Value Change {
                n113 = event-data() -> ()  [unwired: 1 in, 6 out]
                n114 = case shown="True" "Record pH Calibration Reference" {
                  tunnel: [w253 w256] -> w249
                  tunnel: [FALSE FALSE ("Boolean")] -> w250
                  tunnel: [w254 w257] -> w251
                  tunnel: w252 -> [w254 w257]
                  tunnel: w248 -> [w253 _]
                  frame False {
                  }
                  frame True {
                    w256 = Action_Control_1."pH Calibration Standard"  # Event
                  }
                }
              }
              event "Record ORP Calibration": Value Change {
                n115 = event-data() -> ()  [unwired: 1 in, 6 out]
                n116 = case shown="True" "Record ORP Calibration" {
                  tunnel: [w265 w268] -> w261
                  tunnel: [FALSE FALSE ("Boolean")] -> w262
                  tunnel: [w266 w269] -> w263
                  tunnel: w264 -> [w266 w269]
                  tunnel: w260 -> [w265 _]
                  frame False {
                  }
                  frame True {
                    w268 = Action_Control_1."ORP Calibration Standard"  # Event
                  }
                }
              }
              event "Record Salinity Calibration": Value Change {
                n117 = event-data() -> ()  [unwired: 1 in, 6 out]
                n118 = case shown="True" "Record Salinity Calibration" {
                  tunnel: [w277 w280] -> w273
                  tunnel: [FALSE FALSE ("Boolean")] -> w274
                  tunnel: [w278 w281] -> w275
                  tunnel: w276 -> [w278 w281]
                  tunnel: w272 -> [w277 _]
                  frame False {
                  }
                  frame True {
                    w280 = Action_Control_1."Salinity Calibration Standard"  # Event
                  }
                }
              }
              event "Record DO Calibration": Value Change {
                n119 = event-data() -> ()  [unwired: 1 in, 6 out]
                n120 = case shown="True" "Record DO Calibration" {
                  tunnel: [w289 w292] -> w285
                  tunnel: [FALSE FALSE ("Boolean")] -> w286
                  tunnel: [w290 w293] -> w287
                  tunnel: w288 -> [w290 w293]
                  tunnel: w284 -> [w289 _]
                  frame False {
                  }
                  frame True {
                    w292 = Action_Control_1."DO Calibration Standard"  # Event
                  }
                }
              }
              event "Record  SC Calibration": Value Change {
                n121 = event-data() -> ()  [unwired: 1 in, 6 out]
                n122 = case shown="True" "Record  SC Calibration" {
                  tunnel: [w301 w304] -> w297
                  tunnel: [FALSE FALSE ("Boolean")] -> w298
                  tunnel: [w302 w305] -> w299
                  tunnel: w300 -> [w302 w305]
                  tunnel: w296 -> [w301 _]
                  frame False {
                  }
                  frame True {
                    w304 = Action_Control_1."SC Calibration Standard"  # Event
                  }
                }
              }
              event "Increment Depth": Value Change {
                n123 = event-data() -> ()  [unwired: 1 in, 6 out]
                n124 = case shown="True" "Increment Depth" {
                  tunnel: [w313 w316] -> w309
                  tunnel: [FALSE FALSE ("Boolean")] -> w310
                  tunnel: [w314 w317] -> w311
                  tunnel: w312 -> [w314 w317]
                  tunnel: w308 -> [w313 _]
                  frame False {
                  }
                  frame True {
                    w316 = Action_Control_1."Increment Depth Manually"  # Event
                  }
                }
              }
              event "Record Single Sample": Value Change {
                n125 = event-data() -> ()  [unwired: 1 in, 6 out]
                n126 = case shown="True" "Record Single Sample" {
                  tunnel: [w323 w325] -> w322
                  tunnel: [FALSE FALSE] -> w321
                  tunnel: w320 -> [w323 _]
                  frame False {
                  }
                  frame True {
                    w325 = Action_Control_1."Acq. Single Sonde Point"  # Event
                  }
                }
              }
              event "Write Data to Spreadsheet": Value Change {
                n127 = event-data() -> ("OldVal"=w331:bool, "NewVal"=w334:bool)  [unwired: 1 in, 4 out]
                n128 = Not(x=w331) -> (.not. x?=w330:bool)
                n129 = And(x=w330, y=w334) -> (x .and. y?=w328:bool)
                n130 = case shown="True" w328 {
                  tunnel: [w335 w338] -> w333
                  tunnel: [FALSE FALSE ("Boolean")] -> w332
                  tunnel: [w336 w339] -> _
                  tunnel: w329 -> [w336 w339]
                  tunnel: w327 -> [w335 _]
                  frame False {
                  }
                  frame True {
                    w338 = Action_Control_1."Write Sonde Sample Sheet"  # Event
                  }
                }
              }
              event "Sample Not Collected": Value Change {
                n131 = event-data() -> ("NewVal"=w342:bool)  [unwired: 1 in, 5 out]
                n132 = case shown="True" w342 {
                  tunnel: [FALSE FALSE] -> w344
                  tunnel: [w345 w347] -> w343
                  tunnel: w341 -> [_ w347]
                  frame True {
                    w345 = Action_Control_1."Sample Not Collected"  # Event
                  }
                  frame False {
                  }
                }
              }
              event "Record  Sonde Reason": Value Change {
                n133 = event-data() -> ("NewVal"=w350:bool)  [unwired: 1 in, 5 out]
                n134 = case shown="True" w350 {
                  tunnel: [FALSE FALSE] -> w352
                  tunnel: [w353 w355] -> w351
                  tunnel: w349 -> [_ w355]
                  frame True {
                    w353 = Action_Control_1."Record Sonde Reason"  # Event
                  }
                  frame False {
                  }
                }
              }
              event "Start KPRO": Value Change {
                n135 = event-data() -> ()  [unwired: 1 in, 6 out]
                n136 = case shown="True" "Start KPRO" {
                  tunnel: [FALSE FALSE] -> w360
                  tunnel: [w362 w364] -> w359
                  tunnel: w358 -> [_ w364]
                  frame True {
                    w362 = Action_Control_1."Start KPRO Measurements"  # Event
                    n137 = local write "KPRO Finish\nIndicator"(FALSE ("KPRO Finish\nIndicator")) -> ()
                  }
                  frame False {
                  }
                }
              }
              event "Update Depth": Value Change {
                n138 = event-data() -> ()  [unwired: 1 in, 6 out]
                n139 = case shown="True" "Update Depth" {
                  tunnel: [FALSE FALSE] -> w368
                  tunnel: [w370 w372] -> w367
                  tunnel: w366 -> [_ w372]
                  frame True {
                    w370 = Action_Control_1."Update Depth"  # Event
                  }
                  frame False {
                  }
                }
              }
              event "Record IK Reason": Value Change {
                n140 = event-data() -> ()  [unwired: 1 in, 6 out]
                n141 = case shown="True" "Record IK Reason" {
                  tunnel: [FALSE FALSE] -> w377
                  tunnel: [w378 w380] -> w376
                  tunnel: w375 -> [_ w380]
                  frame True {
                    w378 = Action_Control_1."Record IK Reason"  # Event
                  }
                  frame False {
                  }
                }
              }
              event "Finish Tests": Value Change {
                n142 = event-data() -> ()  [unwired: 1 in, 6 out]
                n143 = case shown="True" "Finish Tests" {
                  tunnel: [FALSE FALSE] -> w385
                  tunnel: [w387 w389] -> w384
                  tunnel: w383 -> [_ w389]
                  frame True {
                    w387 = Action_Control_1."Finish KPRO Measurements"  # Event
                    "KPRO Finish\nIndicator" <- TRUE ("KPRO Finish\nIndicator")
                  }
                  frame False {
                  }
                }
              }
              event "Depth mode": Value Change {
                n144 = event-data() -> ()  [unwired: 1 in, 6 out]
                n145 = case shown="True" "Depth mode" {
                  tunnel: [FALSE ("Read String Pot") TRUE ("Read String Pot")] -> w391
                  frame False {
                  }
                  frame True {
                  }
                }
                n146 = local write "Read String Pot"(w391) -> ()
              }
            }
          }
          frame True {
          }
        }
        "Stop" <- w202
        n147 = local read "Stop"() -> (w203:bool)
        n148 = Or(x=w203, y=w202) -> ()  [unwired: 1 out]
        n149 = call <extravilib>:"Write With Abort.vi"("abort"=FALSE, "last element? (F)"=w202, "element"=w200) -> ("channel"=w206:T24)  [unwired: 6 in, 2 out]
        "producer loop" <- w204
      }
    }
  }
  n150 = flat-sequence {
    tunnel: [w422] -> w16
    tunnel: w13 -> [w421]
    tunnel: w12 -> [w420]
    tunnel: w11 -> [w418]
    tunnel: w10 -> [w416]
    tunnel: w9 -> [w415]
    tunnel: w8 -> [w413]
    tunnel: w6 -> [w412]
    tunnel: w4 -> [w411]
    tunnel: w3 -> [w409]
    tunnel: w2 -> [w408]
    tunnel: w1 -> [w407]
    frame #0 {
      w397 = dbl[][] []  # Cumulative Data over 1 string pot
      w401 = T6 {"SC Initial "=0.0, "DO Initial "=0.0, "pH Initial  "=0.0, "ORP  Initial"=0.0, "Temp Initial"=0.0, "Salinity Initial "=0.0}  # Sonde Parameters  Initial Values
      w402 = FALSE  # Read String Pot
      w403 = T16 {"Flow"=0.21081600494384767, "Zeroed \nPressure"=74.74207969932556, "Ik"=0.003788962123473114, "Current Depth"=-100.6, "Feet of Stainless"=40, "Start Depth"=0.0, "Abs Start Depth"=0.0}  # Input Depths  and Parameters Cluster
      w404 = T17 {"Absolute Depth In"=0.0, "Current Absolute Depth"=0.0, "First Absolute Depth"=0.0, "Previous Relative Depth"=0.0, "Current Relative Depth"=0.0, "First Relative Depth"=0.0, "Last Filed Depth"=0.0, "Total Volume In"=0.0, "Total Volume Out"=0.0, "Current Measurement Time"=0.0, "Previous Measurement Time"=0.0}  # Depth Cluster
      w405 = dbl[][] []  # Cumulative Data From File
      n151 = Get Date/Time In Seconds() -> (seconds since 1Jan1904=w400:timestamp)
      n152 = To Double Precision Float(number=w400) -> (double precision float=w399:dbl)
      n153 = while {
        tunnel: w421 -> [w473]
        tunnel: [w474] -> w422
        tunnel: w411 -> [w449]
        tunnel: w420 -> [w472]
        shift-right: [w462] -> _
        shift-left: "Current Sheet" -> [w423]
        tunnel: w418 -> [w464]
        tunnel: w416 -> [w470]
        tunnel: w415 -> [w469]
        shift-right: [w463] -> _
        shift-left: 0 ("row index") -> [w468]
        tunnel: [w467] -> _
        shift-right: [w466] -> _
        shift-left: cluster{"row":i32, "column":i32} {"row"=0, "column"=0} ("start of last occupied row") -> [w465]
        tunnel: w413 -> [w461]
        shift-right: [w455] -> _
        shift-left: dbl[] [] ("Time Array") -> [w456]
        shift-right: [w454] -> _
        shift-left: w405 -> [w453]
        tunnel: w399 -> [w452]
        tunnel: [w451] -> _
        tunnel: w412 -> [w437]
        shift-right: [w447] -> _
        shift-left: refnum<k24>[] [] -> [w436]
        tunnel: w409 -> [w424]
        shift-right: [w425] -> _
        shift-left: w408 -> [w426]
        shift-right: [w445] -> _
        shift-left: w407 -> [w445]
        shift-right: [w442] -> _
        shift-left: w402 -> [w441]
        shift-right: [w429] -> _
        shift-left: w404 -> [w440]
        shift-right: [w439] -> _
        shift-left: w403 -> [w438]
        shift-right: [w433] -> _
        shift-left: w401 -> [_]
        shift-right: [w431] -> _
        shift-left: dbl[][] [] ("Cumulative Sonde \nData Out") -> [w430]
        shift-right: [w428] -> _
        shift-left: w397 -> [w427]
        i -> [w434]
        stop <- w450 stop-if-true
        # "Consumer Data Handling Loop"
        n154 = flat-sequence {
          tunnel: [w478] -> w458
          tunnel: [w477] -> w457
          tunnel: w449 -> [w476]
          tunnel: [w475] -> w448
          frame #0 {
            n155 = call <extravilib>:"Read With Abort.vi"("abort"=FALSE, "channel"=w476) -> ("last element?"=w475:bool, "element"=w478:T23)  [unwired: 5 in, 3 out]
            n156 = feedback #1() -> (w477:T23)  [unwired: 1 in]
            n157 = feedback-in #1(w478) -> ()
          }
        }
        n158 = call <userlib>:"Wait (ms)__ogtk.vi"("error in (no error)"=w473, "milliseconds to wait"=u32 50) -> ("error out"=w460:errorcluster)  [unwired: 8 in, 1 out]
        n159 = call "open select sample sheet.vi"("Number of Sample Sheets"=w461, "error in (no error)"=w460, "Worksheet Names"=w464, "input 1"=w423, "NI_report in"=w472) -> ("error out"=w444:errorcluster, "Current Sample Sheet"=w446:string, "NI_report out"=w471:refnum<class "NI_report.lvclass">)  [unwired: 4 in]
        n160 = flat-sequence {
          tunnel: w424 -> [w491]
          frame #0 {
            n161 = Get Date/Time In Seconds() -> (seconds since 1Jan1904=w492:timestamp)
            n162 = Subtract(x=w492, y=w491) -> (x-y=w493:dbl)
            n163 = local write "Current Time (s)"(w493) -> ()
          }
        }
        n164 = flat-sequence {
          tunnel: w446 -> [w497]
          tunnel: w444 -> [w494]
          tunnel: [w496] -> w443
          tunnel: w423 -> [w495]
          frame #0 {
            n165 = Format Into String(format string="Data from Sample Sheet %d from Excel File", error in=w494, w495) -> (resulting string=→"Table Label":string, error out=w496:errorcluster)  [unwired: 1 in]
            "Current Sample Sheet" <- w497
          }
        }
        n166 = flat-sequence {
          tunnel: w437 -> [w483]
          tunnel: w436 -> [w482]
          tunnel: [w481] -> w435
          tunnel: w434 -> [w480]
          frame #0 {
            n167 = case shown="1, Default" w480 {
              tunnel: w482 -> [w484 w490]
              tunnel: w483 -> [_ w489]
              tunnel: [w484 w487] -> w481
              frame 0 {
              }
              frame 1, Default {
                n168 = local read "Descriptions"() -> (w488:string[])
                n169 = call "Measure DAQ Voltages.vi"("error in (no error)"=w489, "Descriptions"=w488, "Array in"=w490) -> ("Raw Voltages"=w486:dbl[], "Array out"=w487:refnum<k24>[], "Sensor Cluster"=w485:T10)  [unwired: 6 in]
                n170 = local write "Sensor Voltage Cluster"(w485) -> ()
                n171 = local write "Raw Voltages"(w486) -> ()
              }
            }
            "consumer loop" <- w480
          }
        }
        n172 = case shown="\"Init\"" w458 {
          selector: w458 -> [_ _ _ _ _ _ _ _ _ _ _ _ _ _ _ _ _ w1977 _ _ _]
          tunnel: w443 -> [w513 w668 w739 w782 w805 w951 w1143 w1160 w1200 w1247 w1277 w1364 w1465 w1568 w1671 w1774 w1876 w1983 w2063 w2408 w2424]
          tunnel: [w513 w668 w739 w782 w801 w947 w1143 w1160 w1200 w1246 w1275 w1362 w1463 w1566 w1669 w1772 w1874 w1966 w2063 w2408 w2434] -> w474
          tunnel: w448 -> [_ _ _ _ _ _ _ _ _ _ _ _ _ _ _ _ _ _ _ _ _]
          tunnel: w471 -> [w529 w657 w738 w781 w822 w971 w1142 w1159 w1199 w1241 w1288 w1382 w1483 w1586 w1689 w1792 w1894 w1984 w2070 w2407 w2425]
          tunnel: [w528 w667 w737 w780 w821 w970 w1141 w1158 w1198 w1240 w1273 w1359 w1460 w1563 w1666 w1769 w1871 w1971 w2069 w2406 w2439] -> w463
          tunnel: w470 -> [_ _ _ _ _ _ _ _ _ _ w1283 w1377 w1478 w1581 w1684 w1787 w1889 _ _ _ _]
          tunnel: w469 -> [_ _ _ _ _ _ _ _ _ _ w1282 w1376 w1477 w1580 w1683 w1786 w1888 _ _ _ _]
          tunnel: w468 -> [w528 w667 w737 w780 w821 w970 w1141 w1158 w1198 w1240 w1259 w1360 w1461 w1564 w1667 w1770 w1872 w1960 w2069 w2406 w2439]
          tunnel: [w529 w657 w738 w781 w822 w971 w1142 w1159 w1199 w1241 w1278 w1365 w1466 w1569 w1672 w1775 w1877 w1982 w2070 w2407 w2440] -> w467
          tunnel: w423 -> [w527 w666 w736 w779 w809 w955 w1140 w1157 w1197 w1239 w1257 w1373 w1474 w1577 w1680 w1783 w1885 w1979 w2068 w2405 w2438]
          tunnel: [w527 w666 w736 w779 w809 w955 w1140 w1157 w1197 w1239 w1257 w1373 w1474 w1577 w1680 w1783 w1885 w1978 w2068 w2405 w2438] -> w462
          tunnel: [w526 w665 w735 w778 w820 w969 w1139 w1156 w1196 w1238 w1274 w1361 w1462 w1565 w1668 w1771 w1873 w1974 w2067 w2404 w2437] -> w466
          tunnel: w465 -> [w526 w665 w735 w778 w820 w969 w1139 w1156 w1196 w1238 _ _ _ _ _ _ _ w1975 w2067 w2404 w2437]
          tunnel: w464 -> [_ _ _ _ _ _ _ _ _ _ _ _ _ _ _ _ _ w1981 _ _ _]
          tunnel: w461 -> [_ _ _ _ _ _ _ _ _ _ _ _ _ _ _ _ _ w1980 _ _ _]
          tunnel: w457 -> [_ _ _ _ _ _ _ _ _ _ _ _ _ _ _ _ _ w1976 _ _ _]
          tunnel: w456 -> [w512 w664 w734 w777 w819 w968 w1138 w1155 w1195 w1237 w1272 w1358 w1459 w1562 w1665 w1768 w1870 w1970 w2066 w2403 w2436]
          tunnel: [w511 w664 w734 w777 w819 w968 w1138 w1155 w1195 w1237 w1271 w1357 w1458 w1561 w1664 w1767 w1869 w1970 w2066 w2403 w2436] -> w455
          tunnel: [w506 w658 w733 w776 w807 w953 w1137 w1154 w1194 w1236 w1270 w1356 w1457 w1551 w1663 w1766 w1868 w1969 w2055 w2402 w2435] -> w454
          tunnel: w453 -> [w507 w658 w733 w776 w813 w960 w1137 w1154 w1194 w1236 w1269 w1355 w1456 w1551 w1662 w1765 w1867 w1969 w2056 w2402 w2435]
          tunnel: w452 -> [_ _ _ _ _ _ _ _ _ _ w1256 w1354 w1455 w1560 w1661 w1764 w1866 _ _ _ _]
          tunnel: w435 -> [w521 w663 w732 w775 w816 w965 w1136 w1153 w1193 w1235 w1267 w1352 w1453 w1558 w1659 w1762 w1864 w1968 _ w2400 w2429]
          tunnel: [w525 w662 w731 w774 w795 w946 w1135 w1144 w1192 w1234 w1268 w1353 w1454 w1559 w1660 w1763 w1865 w1967 w2062 _ w2430] -> w451
          tunnel: w437 -> [w525 w662 w731 w774 w796 w946 w1135 w1145 w1192 w1234 w1268 w1353 w1454 w1559 w1660 w1763 w1865 w1967 w2064 w2399 w2433]
          tunnel: [_ _ _ _ _ _ _ _ _ _ _ _ _ _ _ _ _ _ FALSE ("aborted?") FALSE ("aborted?") w2432] -> w450
          tunnel: [w517 w663 w732 w775 w816 w965 w1136 w1153 w1193 w1235 w1267 w1352 w1453 w1558 w1659 w1762 w1864 w1968 w2053 w2398 w2429] -> w447
          tunnel: [w524 w661 w730 w773 w818 w967 w1134 w1152 w1191 w1233 w1265 w1350 w1451 w1556 w1657 w1760 w1862 w1965 "Read String Pot" w2397 w2428] -> w442
          tunnel: w441 -> [w524 w661 w730 w773 w818 w967 w1134 w1152 w1191 w1233 w1265 w1350 w1451 w1556 w1657 w1760 w1862 w1965 _ w2397 w2428]
          tunnel: [w504 w651 w725 w769 w811 w957 w1133 w1151 w1190 w1232 w1264 w1349 w1450 w1555 w1656 w1759 w1861 w1964 w2059 w2396 w2427] -> w429
          tunnel: w440 -> [w505 w651 w726 w769 w788 w958 w1133 w1151 w1190 w1232 w1264 w1349 w1450 w1555 w1656 w1759 w1861 w1964 w2045 w2396 w2427]
          tunnel: [w523 w660 w729 w772 w817 w966 w1132 w1150 w1189 w1231 w1263 w1348 w1449 w1554 w1655 w1758 w1860 w1963 w2058 w2395 w2426] -> w439
          tunnel: w438 -> [w523 w660 w729 w772 w817 w966 w1132 w1150 w1189 w1231 w1263 w1348 w1449 w1554 w1655 w1758 w1860 w1963 _ w2395 w2426]
          tunnel: [w522 w659 w728 w771 w806 w952 w1131 w1149 w1188 w1230 w1254 w1347 w1448 w1553 w1654 w1757 w1859 w1962 w2049 w2394 w2421] -> w433
          tunnel: "Sonde Parameters \nInitial Values" -> [w522 w659 w728 w771 w806 w952 w1131 w1149 w1188 w1230 w1261 w1347 w1448 w1553 w1654 w1757 w1859 w1962 w2049 w2394 w2421]
          tunnel: w426 -> [w501 w653 w727 w770 w804 w950 w1130 w1148 w1187 w1229 w1260 w1346 w1447 w1552 w1653 w1756 w1858 w1961 w2048 w2393 w2420]
          tunnel: [w500 w652 w727 w770 w783 w940 w1130 w1148 w1187 w1229 w1260 w1346 w1447 w1552 w1653 w1756 w1858 w1961 w2048 w2393 w2420] -> w425
          tunnel: [w510 w656 w724 w768 w789 w944 w1129 w1147 w1186 w1228 w1255 w1345 w1446 w1550 w1652 w1755 w1857 w1959 w2046 w2392 w2419] -> w431
          tunnel: w430 -> [w509 w656 w724 w768 w789 w944 w1129 w1147 w1186 w1228 w1255 w1345 w1446 w1549 w1652 w1755 w1857 w1959 w2046 w2392 w2419]
          tunnel: [w502 w655 w723 w767 w785 w943 w1128 w1146 w1185 w1227 w1253 w1344 w1445 w1548 w1651 w1754 w1856 w1958 w2043 w2391 w2418] -> w428
          tunnel: w427 -> [w503 w655 w723 w767 w786 w942 w1128 w1146 w1185 w1227 w1253 w1344 w1445 w1548 w1651 w1754 w1856 w1958 w2043 w2391 w2418]
          frame "TimeOut", Default {
            n173 = flat-sequence {
              tunnel: [w638] -> _
              tunnel: [w642] -> w514
              tunnel: [w650] -> _
              tunnel: [w649] -> _
              tunnel: w521 -> [w648]
              tunnel: [w647] -> _
              frame #0 {
                n174 = local read "Input Variables and Slopes"() -> (w640:T1)
                n175 = local read "Input Variables and Slopes"() -> (w644:T1)
                n176 = local read "Sample Sheet Data Row Cluster 2"() -> (w637:T3)
                n177 = local read "Zero In-Line Pressure\n(F = leave as is)"() -> (w643:bool)
                n178 = Unbundle By Name(w644) -> ("DH Pressure Trans Slope"=w650:dbl, "DH Pressure Offset"=w649:dbl)
                n179 = local read "Sensor Voltage Cluster"() -> (w645:T10)
                n180 = local read "Descriptions"() -> (w646:string[])
                n181 = local read "Sensor  Real \nMeasurements"() -> (w641:T7)
                n182 = global read "Kpro Globals.vi" "Current Depth"() -> (w638:sgl)
                n183 = call "DHT Pressure 2016.vi"("Sensor Cluster"=w645, "DHT Pressure Offset"=w649, "Array in"=w648, "DHT Pressure \nSlope"=w650, "Descriptions"=w646, "Zero Pressure\n(F = leave as is)"=w643) -> ("Array out"=w647:refnum<k24>[], "DHT Pressure"=w642:dbl, "Sensor Cluster 2"=w639:T10)  [unwired: 7 in]
                n184 = local write "Sensor Voltage Cluster"(w639) -> ()
                n185 = call "convert sensor voltage to real measurements.vi"("Input Variables and Slopes"=w640, "Sensor  Real Measurements in"=w641, "Sensor Cluster"=w639) -> ("Sensor  Real Measurements out"=w635:T10)  [unwired: 8 in]
                n186 = Unbundle By Name(w635) -> ("Aux 1"=w634:dbl, "Aux 2"=w633:dbl, "Aux 3"=w632:dbl)
                n187 = Bundle By Name(cluster=w637, "Aux1"=w634, "Aux2"=w633, "Aux3"=w632) -> (w636:T3)
                n188 = local write "Sensor  Real \nMeasurements"(w635) -> ()
                n189 = local write "Down hole Pressure"(w642) -> ()
                n190 = local write "Sample Sheet Data Row Cluster 2"(w636) -> ()
                n191 = Add(x=w642, y=w638) -> ()  [unwired: 1 out]
              }
            }
            n192 = case shown="True" "Update Sonde" {
              tunnel: w512 -> [w531 w538]
              tunnel: [w531 w537] -> w511
              tunnel: [w530 w536] -> w510
              tunnel: w509 -> [w530 w535]
              frame False {
              }
              frame True {
                n193 = local read "Sonde Communication Error Out"() -> (w534:errorcluster)
                n194 = local read "Current Time (s)"() -> (w532:dbl)
                n195 = flat-sequence {
                  tunnel: w534 -> [w556]
                  tunnel: [w555] -> w533
                  tunnel: w538 -> [w554]
                  tunnel: [w553] -> w537
                  tunnel: [w552] -> w536
                  tunnel: w535 -> [w551]
                  tunnel: [w541] -> _
                  tunnel: [w550] -> _
                  tunnel: w532 -> [w549]
                  frame #0 {
                    n196 = local read "Sample Sheet Data Row Cluster 2"() -> (w542:T3)
                    n197 = control-ref of="Found Quanta Sonde Com Port"() -> (w548:refnum<vi>)
                    n198 = control-ref of="Current Time (s)"() -> (w544:refnum<vi>)
                    n199 = control-ref of="Temperature"() -> (w545:refnum<vi>)
                    n200 = control-ref of="Sonde Data Display"() -> (w547:refnum<vi>)
                    n201 = control-ref of="Sonde Data Display"() -> (w546:refnum<vi>)
                    n202 = Unbundle By Name(w542) -> ("Sonde Data Cluster.Cumulative\nVolume (ml)"=w539:dbl)
                    n203 = call "Sonde Single Measurement Subvi.vi"("VISAResourceName in"=w548, "Time Array"=w554, "Cumulative Sonde Data"=w551, "Previous time"=w549, "Sonde Data Display"=w547, "Sonde Graph in"=w546, "Temp Graph 3"=w545, "error in (no error)"=w556, "Row Cluster Input"=w542, "reference 5"=w544) -> ("seconds since 1Jan1904"=w550:timestamp, "Cumulative Sonde \nData Out"=w552:dbl[][], "Sample Sheet Data Row Cluster 2"=w541:T3, "output cluster"=w543:T2, "time array out"=w553:dbl[], "error out"=w555:errorcluster)
                    n204 = Bundle By Name(cluster=w541, "Sonde Data Cluster.Cumulative\nVolume (ml)"=w539) -> (w540:T3)
                    n205 = local write "Sample Sheet Data Row Cluster 2"(w540) -> ()
                    n206 = local write "output cluster"(w543) -> ()
                  }
                }
                n207 = local write "Sonde Communication Error Out"(w533) -> ()
              }
            }
            n208 = flat-sequence {
              tunnel: w521 -> [w626]
              tunnel: [w622] -> w520
              tunnel: [w621] -> w519
              frame #0 {
                n209 = local read "Input Variables and Slopes"() -> (w629:T1)
                n210 = Unbundle By Name(w629) -> ("Up Hole Pressure Slope"=w628:dbl, "Up Hole  Pressure Offset"=w625:dbl)
                n211 = local write "Input Variables and Slopes"(w629) -> ()
                n212 = local read "Sensor Voltage Cluster"() -> (w630:T10)
                n213 = local read "Descriptions"() -> (w622:string[])
                n214 = local read "Corrected Pressure Cluster"() -> (w624:T20)
                n215 = call "up hole Pressure 2016.vi"("Sensor Cluster"=w630, "Pressure Offset"=w625, "Array in"=w626, "Pressure \nSlope"=w628, "Descriptions"=w622, "Zero Pressure\n(F = leave as is)"=TRUE) -> ("Array out"=w621:refnum<k24>[], "Uphole Pressure"=w620:dbl, "Sensor Cluster 2"=w627:T10)  [unwired: 6 in, 1 out]
                n216 = local write "Uphole Pressure"(w620) -> ()
                n217 = Bundle By Name(cluster=w624, "Up hole Corrected Pressure"=w620) -> (w623:T20)
                n218 = local write "Sensor Voltage Cluster"(w627) -> ()
                n219 = local write "Corrected Pressure Cluster"(w623) -> ()
              }
            }
            n220 = flat-sequence {
              tunnel: w520 -> [w613]
              tunnel: w519 -> [w616]
              tunnel: [w612] -> w516
              tunnel: [w613] -> w518
              tunnel: [w609] -> w515
              tunnel: [w611] -> w517
              frame #0 {
                w617 = 0.0  # Offset
                n221 = local read "Input Variables and Slopes"() -> (w615:T1)
                n222 = local read "Input Depths \nand Parameters Cluster"() -> (w608:T16)
                n223 = Unbundle By Name(w615) -> ("Flow Slope"=w614:dbl)
                n224 = local read "Input Depths \nand Parameters Cluster"() -> (w619:T16)
                n225 = Unbundle By Name(w608) -> ("Feet of Stainless"=w607:i32)
                n226 = call "Flow 2016.vi"("Descriptions"=w613, "Array in"=w616, "Flow Slope"=w614, "Offset"=w617) -> ("Sensor Cluster"=w612:T10, "Flow (ml/min)"=w609:dbl, "Array out"=w611:refnum<k24>[])  [unwired: 4 in]
                n227 = local write "Sensor Voltage Cluster"(w612) -> ()
                n228 = call "pressure and IK2 2016.vi"("Ft. of SS"=w607, "flow"=w609) -> ("IK"=→"Large Depth IK Graph":dbl)  [unwired: 1 in, 1 out]
                n229 = Bundle By Name(cluster=w619, "Flow"=w609) -> (w618:T16)
                n230 = local write "Input Depths \nand Parameters Cluster"(w618) -> ()
              }
            }
            n231 = flat-sequence {
              tunnel: w518 -> [w595]
              tunnel: w507 -> [w573]
              tunnel: w516 -> [w594]
              tunnel: w505 -> [w578]
              tunnel: [w593] -> w504
              tunnel: w515 -> [w592]
              tunnel: w517 -> [w586]
              tunnel: [w585] -> _
              tunnel: [w565] -> w506
              tunnel: [w579] -> _
              tunnel: w514 -> [w570]
              tunnel: w513 -> [w567]
              tunnel: w503 -> [w566]
              tunnel: [w563] -> w502
              tunnel: w501 -> [w559]
              tunnel: [w558] -> w500
              frame #0 {
                # "Timeout"
                n232 = Unbundle By Name(w578) -> ("Current Relative Depth"=w577:dbl)
                n233 = local read "Input Depths \nand Parameters Cluster"() -> (w589:T16)
                n234 = local read "Culmulative Graph Cluster"() -> (w584:T19)
                n235 = local read "Depth mode"() -> (w575:bool)
                n236 = local read "Input Variables and Slopes"() -> (w591:T1)
                n237 = local read "KPRO Finish\nIndicator"() -> (w572:bool)
                n238 = local read "KPRO SessionOutput File Path"() -> (w579:path)
                n239 = Unbundle By Name(w591) -> ("String Pot Slope"=w590:dbl)
                n240 = Unbundle By Name(w589) -> ()  [unwired: 1 out]
                n241 = local read "Uphole Pressure"() -> (w560:dbl)
                n242 = call "Kpro Read String Pot 2016.vi"("Read String Pot"=w575, "Feet of\nStainless to be\nUsed (Count) in"=w559, "Session Array in"=w566, "Flow"=w592, "Manual Depth In"=w577, "Finished In"=w572, "Depth Cluster in"=w578, "error in (no error)"=w567, "String Pot \nSlope in"=w590, "Sensor Cluster In in"=w594, "Descriptions"=w595, "Pressure in"=w560, "Array in"=w586, "Downhole Pressure Sensor"=w570, "Initial Measurement Input"=FALSE) -> ("Sensor Cluster 2"=w587:T10, "IK"=w569:dbl, "Array out"=w585:refnum<k24>[], "Generate Array Calc IK"=w574:bool, "Feet of\nStainless to be\nUsed (Count) out"=w558:i32, "Depth Cluster out"=w593:T17, "Single String Pot Session Array out"=w563:dbl[][])  [unwired: 4 in, 2 out]
                n243 = local write "Ik"(w569) -> ()
                n244 = local write "Sensor Voltage Cluster"(w587) -> ()
                n245 = Unbundle By Name(w593) -> ("Current Absolute Depth"=w576:dbl)
                n246 = And(x=w574, y=w575) -> ()  [unwired: 1 out]
                n247 = Bundle By Name(cluster=w589, "Feet of Stainless"=w558) -> (w588:T16)
                n248 = local write "Input Depths \nand Parameters Cluster"(w588) -> ()
                n249 = flat-sequence {
                  tunnel: w576 -> [w601]
                  frame #0 {
                    n250 = global write "Kpro Globals.vi" "Current Depth"(w601) -> ()
                    n251 = local write "Current Depth"(w601) -> ()
                    n252 = Divide(x=w601, y=3.281) -> (x/y=w602:dbl)
                    n253 = local read "Sample Sheet Data Row Cluster 2"() -> (w605:T3)
                    n254 = local read "Corrected Pressure Cluster"() -> (w603:T20)
                    n255 = Unbundle By Name(w603) -> ("Up hole Corrected Pressure"=w600:dbl)
                    "Uphole Pressure" <- w600
                    n256 = Bundle By Name(cluster=w605, "Depth"=w601, "Head\nPressure"=w600) -> (w604:T3)
                    n257 = local write "Sample Sheet Data Row Cluster 2"(w604) -> ()
                    n258 = local write "Current \nDepth (m)"(w602) -> ()
                  }
                }
                n259 = case shown="True" FALSE {
                  tunnel: w573 -> [w596 w599]
                  tunnel: w563 -> [_ w597]
                  tunnel: [w596 w598] -> w565
                  frame False {
                  }
                  frame True {
                    n260 = Build Array (concatenate)(w599, w597) -> (w598:dbl[][])
                  }
                }
                n261 = call "Array to Plot 2016.vi"("Input Cumulative Array"=w565, "Input Real Time Array"=w563) -> ("Cumulative - Depth vs.Drive Rate"=w561:cluster{dbl[], dbl[]}, "Cumulative - Depth vs. Ik"=w582:cluster{dbl[], dbl[]}, "Real Time - Depth vs. Drive Rate"=w562:cluster{dbl[], dbl[]}, "Real Time - Depth vs. Ik"=w571:cluster{dbl[], dbl[]}, "Depth Rate"=w568:dbl)  [unwired: 2 in, 1 out]
                n262 = Bundle By Name(cluster=w584, "Cumulative - Depth vs. Ik"=w582, "Real Time - Depth vs. lk"=w571, "Cumulative - Depth vs. Drive Rate"=w561, "Real Time - Depth vs. Drive Rate"=w562) -> (w583:T19)
                n263 = local write "Large Depth IK Graph Cluster"(w571) -> ()
                n264 = local write "Culmulative Graph Cluster"(w583) -> ()
                n265 = local write "Depth Rate\nft/min"(w568) -> ()
                n266 = local write "Current Session"(w563) -> ()
                n267 = local read "Input Depths \nand Parameters Cluster"() -> (w581:T16)
                n268 = local write "Cumulative_data_from_file"(w565) -> ()
                n269 = Unbundle By Name(w581) -> ("Flow"=→"Flow":dbl)
              }
            }
          }
          frame "Finish KPRO Measurements" {
            n270 = flat-sequence {
              tunnel: w651 -> [w701]
              tunnel: [w712] -> w654
              tunnel: w658 -> [w709]
              tunnel: w655 -> [w703]
              tunnel: w653 -> [w702]
              tunnel: [w700] -> _
              tunnel: [w699] -> w652
              frame #0 {
                n271 = local read "Input Depths \nand Parameters Cluster"() -> (w711:T16)
                n272 = Unbundle By Name(w711) -> ()  [unwired: 1 out]
                n273 = Build Array (concatenate)(w709, w703) -> (w704:dbl[][])
                n274 = local read "KPRO SessionOutput File Path"() -> (w707:path)
                n275 = case shown="True" TRUE {
                  tunnel: w707 -> [w713 w722]
                  tunnel: errorcluster {"status"=FALSE, "code"=0, "source"=""} ("error constant") -> [w714 w719]
                  tunnel: [w714 w718] -> _
                  tunnel: [w713 w715] -> w706
                  frame False {
                  }
                  frame True {
                    n276 = call-poly <vilib>:"Write Delimited Spreadsheet.vi"("file path (dialog if empty)"=w722, "1D data"="KPRO test report header", "append to file? (new file:F)"=FALSE, "error in (no error)"=w719, "transpose? (no:F)"=FALSE, "delimiter (\\t)"="," ("delimiter (\\t)")) -> ("new file path (Not A Path if cancelled)"=w715:path, "error out"=w718:errorcluster)  [unwired: 8 in]
                  }
                }
                n277 = call "Finished Collection Write File.vi"("Cluster in"=w701, "Corrected Array in"=w704, "Feet of\nStainless to be\nUsed (Count) in"=w702, "Output KPRO"=w706) -> ("Corrected Array out"=w712:dbl[][], "Depth to \nbe Used \n(Feet)"=w700:sgl, "Feet of\nStainless to be\nUsed (Count) out"=w699:i32)  [unwired: 5 in]
                n278 = Bundle By Name(cluster=w711, "Feet of Stainless"=w699) -> (w710:T16)
                n279 = local write "Current Depth"(w700) -> ()
                n280 = local write "Input Depths \nand Parameters Cluster"(w710) -> ()
              }
            }
            n281 = disable-structure shown="Disabled" {
              disable-tunnel: w657 -> [w679 _]
              disable-tunnel: w654 -> [_ _]
              frame Disabled {
                n282 = disable-structure shown="Disabled" {
                  disable-tunnel: w679 -> [w684 _]
                  disable-tunnel: [w683 _] -> w678
                  disable-tunnel: [w682 _] -> w677
                  disable-tunnel: [w681 _] -> w676
                  frame Disabled {
                    n283 = call "open select sample sheet.vi"("input 1"=0 ("Active Sample Sheet"), "NI_report in"=w684) -> ("error out"=w683:errorcluster, "Current Sample Sheet"=w682:string, "NI_report out"=w681:refnum<class "NI_report.lvclass">)  [unwired: 7 in]
                  }
                  frame Enabled {
                  }
                }
                n284 = flat-sequence {
                  tunnel: [w697] -> _
                  tunnel: [w696] -> _
                  tunnel: w678 -> [w695]
                  tunnel: [w685] -> _
                  tunnel: [w688] -> _
                  tunnel: w677 -> [w686]
                  tunnel: w676 -> [w685]
                  frame #0 {
                    n285 = call "get sample sheet data cells.vi"("error in (no error)"=w695, "NI_report in"=w685) -> ("error out"=w698:errorcluster, "data"=w693:string[][], "NI_report out"=w697:refnum<class "NI_report.lvclass">, "left edge output cluster"=w691:cluster{"row":i32, "column":i32})  [unwired: 5 in, 1 out]
                    n286 = Array Subset(array=w693, index (col)=2 ("index")) -> ()  [unwired: 3 in, 1 out]
                    n287 = call "find last occupied cell.vi"("Active Sheet"=w686, "Header Rows to remove"=3, "sub array start"=w691, "error in (no error)"=w698) -> ("row max value"=w690:i32, 13:"start of last occupied row"=w696:cluster{"row":i32, "column":i32}, 14:"start of last occupied row"=w689:string, "error out"=w688:errorcluster)  [unwired: 5 in, 3 out]
                    n288 = local write "row max value"(w690) -> ()
                    n289 = local write "last occupied cell's name"(w689) -> ()
                    n290 = local write "Sonde Data Array"(T12[] [{"Head"=0.0, "Depth"=0.0, "Time"="19:00", "Cumulative\nVolume"=0.0, "Sp. Conductance"={"Value"=0.506, "%"=0.0, "Tol."=TRUE}, "Dissolved Oxygen"={"Value"=35.14, "%"=0.0, "Tol."=TRUE}, "pH"={"Value"=4.81, "%"=0.0, "Tol."=TRUE}, "ORP"={"Value"=390.0, "%"=0.0, "Tol."=TRUE}, "Temperature"={"Value"=23.86, "%"=0.0, "Tol."=TRUE}, "Salinity"={"Value"=0.24, "%"=0.0, "Tol."=TRUE}, "Final Tol."=TRUE, "Final"=FALSE, "Time 2"=timestamp(0 s since 1904-01-01), "Aux 1"=0.0, "Aux 2"=0.0, "Aux 3"=0.0}, {"Head"=0.0, "Depth"=0.0, "Time"="19:00", "Cumulative\nVolume"=0.0, "Sp. Conductance"={"Value"=0.506, "%"=0.0, "Tol."=TRUE}, "Dissolved Oxygen"={"Value"=35.12, "%"=0.0, "Tol."=TRUE}, "pH"={"Value"=4.81, "%"=0.0, "Tol."=TRUE}, "ORP"={"Value"=390.0, "%"=0.0, "Tol."=TRUE}, "Temperature"={"Value"=23.89, "%"=0.0, "Tol."=TRUE}, "Salinity"={"Value"=0.24, "%"=0.0, "Tol."=TRUE}, "Final Tol."=TRUE, "Final"=FALSE, "Time 2"=timestamp(0 s since 1904-01-01), "Aux 1"=0.0, "Aux 2"=0.0, "Aux 3"=0.0}, {"Head"=0.0, "Depth"=0.0, "Time"="19:00", "Cumulative\nVolume"=0.0, "Sp. Conductance"={"Value"=0.506, "%"=0.0, "Tol."=TRUE}, "Dissolved Oxygen"={"Value"=35.14, "%"=0.0, "Tol."=TRUE}, "pH"={"Value"=4.81, "%"=0.0, "Tol."=TRUE}, "ORP"={"Value"=390.0, "%"=0.0, "Tol."=TRUE}, "Temperature"={"Value"=23.86, "%"=0.0, "Tol."=TRUE}, "Salinity"={"Value"=0.24, "%"=0.0, "Tol."=TRUE}, "Final Tol."=TRUE, "Final"=FALSE, "Time 2"=timestamp(0 s since 1904-01-01), "Aux 1"=0.0, "Aux 2"=0.0, "Aux 3"=0.0}, {"Head"=0.0, "Depth"=0.0, "Time"="", "Cumulative\nVolume"=0.0, "Sp. Conductance"={"Value"=0.0, "%"=0.0, "Tol."=FALSE}, "Dissolved Oxygen"={"Value"=0.0, "%"=0.0, "Tol."=FALSE}, "pH"={"Value"=0.0, "%"=0.0, "Tol."=FALSE}, "ORP"={"Value"=0.0, "%"=0.0, "Tol."=FALSE}, "Temperature"={"Value"=0.0, "%"=0.0, "Tol."=FALSE}, "Salinity"={"Value"=0.0, "%"=0.0, "Tol."=FALSE}, "Final Tol."=FALSE, "Final"=FALSE, "Time 2"=timestamp(0 s since 1904-01-01), "Aux 1"=0.0, "Aux 2"=0.0, "Aux 3"=0.0}, {"Head"=0.0, "Depth"=0.0, "Time"="", "Cumulative\nVolume"=0.0, "Sp. Conductance"={"Value"=0.0, "%"=0.0, "Tol."=FALSE}, "Dissolved Oxygen"={"Value"=0.0, "%"=0.0, "Tol."=FALSE}, "pH"={"Value"=0.0, "%"=0.0, "Tol."=FALSE}, "ORP"={"Value"=0.0, "%"=0.0, "Tol."=FALSE}, "Temperature"={"Value"=0.0, "%"=0.0, "Tol."=FALSE}, "Salinity"={"Value"=0.0, "%"=0.0, "Tol."=FALSE}, "Final Tol."=FALSE, "Final"=FALSE, "Time 2"=timestamp(0 s since 1904-01-01), "Aux 1"=0.0, "Aux 2"=0.0, "Aux 3"=0.0}, {"Head"=0.0, "Depth"=0.0, "Time"="", "Cumulative\nVolume"=0.0, "Sp. Conductance"={"Value"=0.0, "%"=0.0, "Tol."=FALSE}, "Dissolved Oxygen"={"Value"=0.0, "%"=0.0, "Tol."=FALSE}, "pH"={"Value"=0.0, "%"=0.0, "Tol."=FALSE}, "ORP"={"Value"=0.0, "%"=0.0, "Tol."=FALSE}, "Temperature"={"Value"=0.0, "%"=0.0, "Tol."=FALSE}, "Salinity"={"Value"=0.0, "%"=0.0, "Tol."=FALSE}, "Final Tol."=FALSE, "Final"=FALSE, "Time 2"=timestamp(0 s since 1904-01-01), "Aux 1"=0.0, "Aux 2"=0.0, "Aux 3"=0.0}, {"Head"=0.0, "Depth"=0.0, "Time"="", "Cumulative\nVolume"=0.0, "Sp. Conductance"={"Value"=0.0, "%"=0.0, "Tol."=FALSE}, "Dissolved Oxygen"={"Value"=0.0, "%"=0.0, "Tol."=FALSE}, "pH"={"Value"=0.0, "%"=0.0, "Tol."=FALSE}, "ORP"={"Value"=0.0, "%"=0.0, "Tol."=FALSE}, "Temperature"={"Value"=0.0, "%"=0.0, "Tol."=FALSE}, "Salinity"={"Value"=0.0, "%"=0.0, "Tol."=FALSE}, "Final Tol."=FALSE, "Final"=FALSE, "Time 2"=timestamp(0 s since 1904-01-01), "Aux 1"=0.0, "Aux 2"=0.0, "Aux 3"=0.0}, {"Head"=0.0, "Depth"=0.0, "Time"="", "Cumulative\nVolume"=0.0, "Sp. Conductance"={"Value"=0.0, "%"=0.0, "Tol."=FALSE}, "Dissolved Oxygen"={"Value"=0.0, "%"=0.0, "Tol."=FALSE}, "pH"={"Value"=0.0, "%"=0.0, "Tol."=FALSE}, "ORP"={"Value"=0.0, "%"=0.0, "Tol."=FALSE}, "Temperature"={"Value"=0.0, "%"=0.0, "Tol."=FALSE}, "Salinity"={"Value"=0.0, "%"=0.0, "Tol."=FALSE}, "Final Tol."=FALSE, "Final"=FALSE, "Time 2"=timestamp(0 s since 1904-01-01), "Aux 1"=0.0, "Aux 2"=0.0, "Aux 3"=0.0}, {"Head"=0.0, "Depth"=0.0, "Time"="", "Cumulative\nVolume"=0.0, "Sp. Conductance"={"Value"=0.0, "%"=0.0, "Tol."=FALSE}, "Dissolved Oxygen"={"Value"=0.0, "%"=0.0, "Tol."=FALSE}, "pH"={"Value"=0.0, "%"=0.0, "Tol."=FALSE}, "ORP"={"Value"=0.0, "%"=0.0, "Tol."=FALSE}, "Temperature"={"Value"=0.0, "%"=0.0, "Tol."=FALSE}, "Salinity"={"Value"=0.0, "%"=0.0, "Tol."=FALSE}, "Final Tol."=FALSE, "Final"=FALSE, "Time 2"=timestamp(0 s since 1904-01-01), "Aux 1"=0.0, "Aux 2"=0.0, "Aux 3"=0.0}] ("Sonde Data Array")) -> ()
                  }
                }
              }
              frame Enabled {
              }
            }
            n291 = disable-structure shown="Disabled" {
              disable-tunnel: w654 -> [w669 _]
              frame Disabled {
                n292 = flat-sequence {
                  tunnel: w669 -> [w674]
                  frame #0 {
                    n293 = control-ref of="KPRO SessionOutput File Path"() -> (w672:refnum<vi>)
                    n294 = call "write KPRO file.vi"("Corrected Array in"=w674, "Generate Array Calc IK"=TRUE, "Path in"=w672) -> ("paths ok"=w671:bool, "appended path"=w670:path)  [unwired: 7 in]
                    n295 = case shown="True" w671 {
                      tunnel: w670 -> [_ w675]
                      frame False {
                      }
                      frame True {
                        n296 = local write "KPRO SessionOutput File Path"(w675) -> ()
                      }
                    }
                  }
                }
              }
              frame Enabled {
              }
            }
          }
          frame "Update Depth" {
            n297 = flat-sequence {
              tunnel: w726 -> [w751]
              tunnel: [w748] -> w725
              frame #0 {
                n298 = Unbundle By Name(w751) -> ("First Absolute Depth"=w749:dbl)
                n299 = local read "Current Depth"() -> (w745:sgl)
                n300 = local read "Sensor  Real \nMeasurements"() -> (w752:T7)
                n301 = Greater?(x="New Depth", y=w745) -> (0:w744:bool)
                n302 = case shown="False" w744 {
                  tunnel: [w761 w766] -> w750
                  tunnel: w749 -> [w760 w765]
                  tunnel: "New Depth" -> [w758 w763]
                  tunnel: w745 -> [w757 w762]
                  frame True {
                    n303 = Subtract(x=w757, y=w758) -> (x-y=w759:dbl)
                    n304 = Subtract(x=w760, y=w759) -> (x-y=w761:dbl)
                  }
                  frame False {
                    # "Reverse inputs \non Subtraction"
                    n305 = Subtract(x=w763, y=w762) -> (x-y=w764:dbl)
                    n306 = Subtract(x=w765, y=w764) -> (x-y=w766:dbl)
                  }
                }
                n307 = Unbundle By Name(w752) -> ("String Pot"=w741:dbl)
                n308 = Bundle By Name(cluster=w751, "Absolute Depth In"="New Depth", "Current Absolute Depth"="New Depth", "First Absolute Depth"=w750) -> (w743:T17)
                n309 = local read "Read String Pot"() -> (w740:bool)
                n310 = case shown="False" w740 {
                  tunnel: w743 -> [w753 w756]
                  tunnel: [w753 w755] -> w742
                  tunnel: w741 -> [_ w754]
                  frame False {
                  }
                  frame True {
                    n311 = Bundle By Name(cluster=w756, "Current Relative Depth"=w754) -> (w755:T17)
                  }
                }
                n312 = call "calculate current depth.vi"("Cluster in"=w742) -> ("Cluster out"=w748:T17)  [unwired: 10 in]
                n313 = Unbundle By Name(w748) -> ("Current Absolute Depth"=w747:dbl)
                n314 = local write "Current Depth"(w747) -> ()
                n315 = global write "Kpro Globals.vi" "Current Depth"(w747) -> ()
              }
            }
          }
          frame "IK vs Time" {
          }
          frame "Start KPRO Measurements" {
            n316 = flat-sequence {
              tunnel: w805 -> [w832]
              tunnel: w804 -> [w831]
              tunnel: [w830] -> w803
              tunnel: [w829] -> w802
              tunnel: [w826] -> w784
              frame #0 {
                n317 = local read "Input Variables and Slopes"() -> (w824:T1)
                n318 = Unbundle By Name(w824) -> ("Depth to Water Table"=w825:dbl)
                n319 = local read "Input Depths \nand Parameters Cluster"() -> (w828:T16)
                n320 = disable-structure shown="Enabled" {
                  disable-tunnel: w825 -> [w839 w840]
                  disable-tunnel: [w838 w840] -> w823
                  disable-tunnel: w832 -> [w837 w842]
                  disable-tunnel: [w836 w842] -> w829
                  disable-tunnel: w831 -> [w835 w841]
                  disable-tunnel: [w834 w841] -> w826
                  frame Enabled {
                    n321 = call <vilib>:"Clear Errors.vi"("error in (no error)"=w837) -> ("error out"=w833:errorcluster)  [unwired: 5 in, 1 out]
                    n322 = call "New Stainless Correction Pop Up 2016.vi"("error in (no error)"=w833, "New Feet\n of Stainless\n(Count)"=w835, "Depth to \nWater Table\nInput"=w839) -> ("error in (no error) 2"=w836:errorcluster, "Feet of\nStainless to be\nUsed (Count)"=w834:i32, "Depth to \nWater Table\nOutput"=w838:dbl)  [unwired: 6 in]
                  }
                  frame Disabled {
                  }
                }
                n323 = Bundle By Name(cluster=w824, "Depth to Water Table"=w823) -> (w830:T1)
                n324 = Bundle By Name(cluster=w828, "Feet of Stainless"=w826) -> (w827:T16)
                n325 = local write "Input Depths \nand Parameters Cluster"(w827) -> ()
              }
            }
            n326 = flat-sequence {
              tunnel: w816 -> [w870]
              tunnel: [w869] -> w815
              tunnel: w803 -> [w868]
              tunnel: w802 -> [w867]
              tunnel: [w866] -> w801
              tunnel: [w856] -> w800
              frame #0 {
                n327 = control-ref of="Input Variables and Slopes"() -> (w862:refnum<vi>)
                n328 = control-ref of="Sensor Voltage Cluster"() -> (w860:refnum<vi>)
                n329 = control-ref of="Zero In-Line Pressure\n(F = leave as is)"() -> (w859:refnum<vi>)
                n330 = control-ref of="Output File Path"() -> (w863:refnum<vi>)
                n331 = control-ref of="Descriptions"() -> (w861:refnum<vi>)
                n332 = call "measure down hole pressure and save to csv file.vi"("Path in"=w863, "reference 3"=w861, "reference in"=w862, "reference 4"=w860, "reference 5"=w859, "Record DTW File"="Record DTW File", "error in (no error)"=w867, "Array in"=w870, "Input Variables and Slopes"=w868) -> ("DTW path 2"=→"Down hole Pressure Transducer CSV data  path 2":path, "Array out"=w869:refnum<k24>[], "In-Line Pressure"=w856:dbl, "error out"=w866:errorcluster)  [unwired: 3 in]
                "Down hole Pressure" <- w856
                n333 = local read "Corrected Pressure Cluster"() -> (w858:T20)
                n334 = Bundle By Name(cluster=w858, "Down hole Corrected Pressure"=w856) -> (w857:T20)
                n335 = invoke on="Update Sonde" class="Bool (strict)" method="Reinit To Default"() -> ()  [unwired: 3 in, 3 out]
                n336 = local write "Corrected Pressure Cluster"(w857) -> ()
                n337 = property on="Large Depth IK Graph" class="WFChart (strict)"("History Data"=dbl[] []) -> ()  [unwired: 2 in, 2 out]
              }
            }
            n338 = flat-sequence {
              tunnel: w815 -> [w934]
              tunnel: [w930] -> w799
              tunnel: [w929] -> w798
              frame #0 {
                n339 = local read "Input Variables and Slopes"() -> (w937:T1)
                n340 = Unbundle By Name(w937) -> ("Up Hole Pressure Slope"=w936:dbl, "Up Hole  Pressure Offset"=w933:dbl)
                n341 = local write "Input Variables and Slopes"(w937) -> ()
                n342 = local read "Sensor Voltage Cluster"() -> (w938:T10)
                n343 = local read "Descriptions"() -> (w930:string[])
                n344 = local read "Corrected Pressure Cluster"() -> (w932:T20)
                n345 = call "up hole Pressure 2016.vi"("Sensor Cluster"=w938, "Pressure Offset"=w933, "Array in"=w934, "Pressure \nSlope"=w936, "Descriptions"=w930, "Zero Pressure\n(F = leave as is)"=TRUE) -> ("Array out"=w929:refnum<k24>[], "Uphole Pressure"=w928:dbl, "Sensor Cluster 2"=w935:T10)  [unwired: 6 in, 1 out]
                n346 = Bundle By Name(cluster=w932, "Up hole Corrected Pressure"=w928) -> (w931:T20)
                n347 = local write "Sensor Voltage Cluster"(w935) -> ()
                n348 = local write "Corrected Pressure Cluster"(w931) -> ()
                n349 = local write "Uphole Pressure"(w928) -> ()
              }
            }
            n350 = local read "Input Variables and Slopes"() -> (w794:T1)
            n351 = Unbundle By Name(w794) -> ("String Pot Slope"=w793:dbl)
            n352 = call "depth read from string pot 2016.vi"("Descriptions"=w799, "error in (no error)"=w796, "String Pot \nSlope"=w793, "Array in"=w798) -> ("Array out"=w797:refnum<k24>[], "Depth"=w791:dbl, "error out"=w795:errorcluster)  [unwired: 12 in, 1 out]
            n353 = flat-sequence {
              tunnel: w791 -> [w844]
              tunnel: [w843] -> w790
              frame #0 {
                w845 = 15  # Filter Size
                # "Functional Global in \nBoxcar Integrator\nInitialize filter array to \ncurrent string pot value"
                n354 = call "Boxcar filter2016.vi"("Initialize"=TRUE, "Filter Size"=w845, "Filter Input"=w844) -> ("Filter Output"=w843:dbl)
              }
            }
            n355 = flat-sequence {
              tunnel: [w847] -> w792
              frame #0 {
                n356 = Tick Count (ms)() -> (millisecond timer value=w849:u32)
                n357 = Divide(x=w849, y=u32 1000) -> (x/y=w847:dbl)
              }
            }
            n358 = flat-sequence {
              tunnel: [w854] -> w787
              tunnel: w790 -> [w851]
              tunnel: w792 -> [w853]
              tunnel: w788 -> [w852]
              frame #0 {
                n359 = local read "Current Depth"() -> (w850:sgl)
                n360 = Bundle By Name(cluster=w852, "Previous Relative Depth"=w851, "Current Relative Depth"=w851, "First Relative Depth"=w851, "Current Measurement Time"=w853, "Previous Measurement Time"=w853, "Absolute Depth In"=w850, "Current Absolute Depth"=w850, "First Absolute Depth"=w850) -> (w854:T17)
              }
            }
            n361 = flat-sequence {
              tunnel: w799 -> [w921]
              tunnel: w797 -> [w924]
              tunnel: [w919] -> w812
              tunnel: [w921] -> w814
              tunnel: [w920] -> w810
              tunnel: [w918] -> w808
              frame #0 {
                w925 = 0.0  # Offset
                n362 = local read "Input Variables and Slopes"() -> (w923:T1)
                n363 = Unbundle By Name(w923) -> ("Flow Slope"=w922:dbl)
                n364 = local read "Input Depths \nand Parameters Cluster"() -> (w927:T16)
                n365 = call "Flow 2016.vi"("Descriptions"=w921, "Array in"=w924, "Flow Slope"=w922, "Offset"=w925) -> ("Sensor Cluster"=w919:T10, "Flow (ml/min)"=w920:dbl, "Array out"=w918:refnum<k24>[])  [unwired: 4 in]
                n366 = local write "Sensor Voltage Cluster"(w919) -> ()
                n367 = Bundle By Name(cluster=w927, "Flow"=w920) -> (w926:T16)
                n368 = local write "Input Depths \nand Parameters Cluster"(w926) -> ()
              }
            }
            n369 = flat-sequence {
              tunnel: w814 -> [w906]
              tunnel: w813 -> [w886]
              tunnel: w812 -> [w905]
              tunnel: w787 -> [w904]
              tunnel: [w903] -> w811
              tunnel: w810 -> [w902]
              tunnel: w808 -> [w896]
              tunnel: [w895] -> _
              tunnel: [w877] -> w807
              tunnel: w800 -> [w890]
              tunnel: w786 -> [w881]
              tunnel: [w878] -> w785
              tunnel: w784 -> [w874]
              tunnel: [w872] -> w783
              frame #0 {
                n370 = local read "Culmulative Graph Cluster"() -> (w894:T19)
                n371 = local read "Input Depths \nand Parameters Cluster"() -> (w899:T16)
                n372 = local read "Input Variables and Slopes"() -> (w901:T1)
                n373 = local read "Uphole Pressure"() -> (w873:dbl)
                n374 = local read "KPRO Finish\nIndicator"() -> (w891:bool)
                n375 = local read "Depth mode"() -> (w887:bool)
                n376 = Unbundle By Name(w901) -> ("String Pot Slope"=w900:dbl)
                n377 = Unbundle By Name(w899) -> ()  [unwired: 1 out]
                n378 = call "Kpro Read String Pot 2016.vi"("Read String Pot"=w887, "Feet of\nStainless to be\nUsed (Count) in"=w874, "Session Array in"=dbl[][] [], "Flow"=w902, "Finished In"=w891, "Depth Cluster in"=w904, "String Pot \nSlope in"=w900, "Sensor Cluster In in"=w905, "Descriptions"=w906, "Pressure in"=w873, "Array in"=w896, "Downhole Pressure Sensor"=w890, "Initial Measurement Input"=TRUE) -> ("Sensor Cluster 2"=w897:T10, "Array out"=w895:refnum<k24>[], "Generate Array Calc IK"=w879:bool, "Feet of\nStainless to be\nUsed (Count) out"=w872:i32, "Depth Cluster out"=w903:T17, "Single String Pot Session Array out"=w878:dbl[][])  [unwired: 6 in, 3 out]
                n379 = local write "Current Session"(w878) -> ()
                n380 = Build Array (concatenate)(w886, w881) -> (w882:dbl[][])
                n381 = local write "Sensor Voltage Cluster"(w897) -> ()
                n382 = Unbundle By Name(w903) -> ("Current Absolute Depth"=w885:dbl)
                n383 = Bundle By Name(cluster=w899, "Feet of Stainless"=w872) -> (w898:T16)
                n384 = local write "Input Depths \nand Parameters Cluster"(w898) -> ()
                n385 = flat-sequence {
                  tunnel: w885 -> [w911]
                  frame #0 {
                    n386 = global write "Kpro Globals.vi" "Current Depth"(w911) -> ()
                    n387 = local write "Current Depth"(w911) -> ()
                    n388 = Divide(x=w911, y=3.281) -> (x/y=w912:dbl)
                    n389 = local read "Sample Sheet Data Row Cluster 2"() -> (w916:T3)
                    n390 = local read "Corrected Pressure Cluster"() -> (w914:T20)
                    n391 = Unbundle By Name(w914) -> ("Up hole Corrected Pressure"=w913:dbl)
                    n392 = Bundle By Name(cluster=w916, "Depth"=w911, "Head\nPressure"=w913) -> (w915:T3)
                    n393 = local write "Sample Sheet Data Row Cluster 2"(w915) -> ()
                    n394 = local write "Current \nDepth (m)"(w912) -> ()
                  }
                }
                n395 = case shown="True" FALSE {
                  tunnel: w878 -> [_ w910]
                  tunnel: [w907 w909] -> w877
                  tunnel: w882 -> [w907 w908]
                  frame False {
                  }
                  frame True {
                    n396 = Build Array (concatenate)(w908, w910) -> (w909:dbl[][])
                  }
                }
                n397 = call "Array to Plot 2016.vi"("Input Cumulative Array"=w877, "Input Real Time Array"=w878) -> ("Cumulative - Depth vs.Drive Rate"=w876:cluster{dbl[], dbl[]}, "Cumulative - Depth vs. Ik"=w892:cluster{dbl[], dbl[]}, "Real Time - Depth vs. Drive Rate"=w875:cluster{dbl[], dbl[]}, "Real Time - Depth vs. Ik"=w888:cluster{dbl[], dbl[]}, "Depth Rate"=w884:dbl)  [unwired: 2 in, 1 out]
                n398 = Bundle By Name(cluster=w894, "Cumulative - Depth vs. Ik"=w892, "Real Time - Depth vs. lk"=w888, "Cumulative - Depth vs. Drive Rate"=w876, "Real Time - Depth vs. Drive Rate"=w875) -> (w893:T19)
                n399 = local write "Culmulative Graph Cluster"(w893) -> ()
                n400 = local write "Large Depth IK Graph Cluster"(w888) -> ()
                n401 = local write "Depth Rate\nft/min"(w884) -> ()
                n402 = local write "Cumulative_data_from_file"(w877) -> ()
                n403 = control-ref of="KPRO SessionOutput File Path"() -> (w889:refnum<vi>)
                n404 = call "write KPRO file.vi"("Corrected Array in"=w877, "Generate Array Calc IK"=w879, "Path in"=w889) -> ()  [unwired: 7 in, 2 out]
              }
            }
          }
          frame "Increment Depth Manually" {
            n405 = disable-structure shown="Enabled" {
              disable-tunnel: w951 -> [w976 w994]
              disable-tunnel: w950 -> [w975 _]
              disable-tunnel: [w974 _] -> w941
              disable-tunnel: [w973 w995] -> w949
              disable-tunnel: [w972 w994] -> w948
              frame Disabled {
                n406 = flat-sequence {
                  tunnel: w976 -> [w984]
                  tunnel: [w983] -> w972
                  tunnel: w975 -> [w982]
                  tunnel: [w981] -> w974
                  tunnel: [w977] -> w973
                  frame #0 {
                    n407 = local read "Input Variables and Slopes"() -> (w979:T1)
                    n408 = Unbundle By Name(w979) -> ("Depth to Water Table"=w980:dbl)
                    n409 = disable-structure shown="Enabled" {
                      disable-tunnel: w980 -> [w990 w991]
                      disable-tunnel: [w989 w991] -> w978
                      disable-tunnel: w984 -> [w988 w993]
                      disable-tunnel: [w987 w993] -> w983
                      disable-tunnel: w982 -> [w986 w992]
                      disable-tunnel: [w985 w992] -> w981
                      frame Enabled {
                        n410 = call "New Stainless Correction Pop Up 2016.vi"("error in (no error)"=w988, "New Feet\n of Stainless\n(Count)"=w986, "Depth to \nWater Table\nInput"=w990) -> ("error in (no error) 2"=w987:errorcluster, "Feet of\nStainless to be\nUsed (Count)"=w985:i32, "Depth to \nWater Table\nOutput"=w989:dbl)  [unwired: 6 in]
                      }
                      frame Disabled {
                      }
                    }
                    n411 = Bundle By Name(cluster=w979, "Depth to Water Table"=w978) -> (w977:T1)
                  }
                }
              }
              frame Enabled {
                n412 = local read "Input Variables and Slopes"() -> (w995:T1)
              }
            }
            n413 = flat-sequence {
              tunnel: w965 -> [w1091]
              tunnel: [w1090] -> w964
              tunnel: w949 -> [w1089]
              tunnel: w948 -> [w1088]
              tunnel: [w1087] -> w947
              tunnel: [w1083] -> w945
              frame #0 {
                n414 = flat-sequence {
                  tunnel: [w1108] -> w1096
                  tunnel: [w1097] -> w1095
                  tunnel: [w1107] -> w1094
                  tunnel: [w1106] -> w1093
                  tunnel: [w1105] -> w1092
                  tunnel: w1091 -> [w1104]
                  tunnel: [w1103] -> w1090
                  tunnel: w1089 -> [w1099]
                  tunnel: [w1097] -> w1083
                  frame #0 {
                    n415 = local read "Zero In-Line Pressure\n(F = leave as is)"() -> (w1098:bool)
                    n416 = Unbundle By Name(w1099) -> ("DH Pressure Trans Slope"=w1106:dbl, "DH Pressure Offset"=w1105:dbl)
                    n417 = local read "Sensor Voltage Cluster"() -> (w1101:T10)
                    n418 = local write "Input Variables and Slopes"(w1099) -> ()
                    n419 = local read "Descriptions"() -> (w1102:string[])
                    n420 = global read "Kpro Globals.vi" "Current Depth"() -> (w1108:sgl)
                    n421 = call "DHT Pressure 2016.vi"("Sensor Cluster"=w1101, "DHT Pressure Offset"=w1105, "Array in"=w1104, "DHT Pressure \nSlope"=w1106, "Descriptions"=w1102, "Zero Pressure\n(F = leave as is)"=w1098) -> ("Array out"=w1103:refnum<k24>[], "DHT Pressure"=w1107:dbl, "Sensor Cluster 2"=w1100:T10)  [unwired: 7 in]
                    n422 = local write "Sensor Voltage Cluster"(w1100) -> ()
                    n423 = Add(x=w1107, y=w1108) -> (x+y=w1097:dbl)
                    n424 = local write "Down hole Pressure"(w1097) -> ()
                  }
                }
                n425 = local read "Record DTW File"() -> (w1086:bool)
                n426 = case shown="True" w1086 {
                  selector: w1086 -> [w1110 _]
                  tunnel: [w1110 FALSE ("Boolean")] -> _
                  tunnel: w1095 -> [_ w1122]
                  tunnel: w1096 -> [_ w1123]
                  tunnel: w1092 -> [_ w1120]
                  tunnel: w1094 -> [_ w1121]
                  tunnel: w1093 -> [_ w1119]
                  tunnel: w1088 -> [w1109 w1114]
                  tunnel: [w1109 w1113] -> w1087
                  frame False {
                  }
                  frame True {
                    n427 = Build Array(w1123, w1122, w1121, w1120, w1119) -> (w1126:dbl[])
                    n428 = local read "Output File Path"() -> (w1118:path)
                    n429 = call-poly <userlib>:"Strip Path__ogtk.vi"("path"=w1118) -> ("stripped path"=w1117:path)  [unwired: 1 out]
                    n430 = call-poly <userlib>:"Strip Path__ogtk.vi"("path"=path "DTW.csv") -> ("name"=w1115:string)  [unwired: 1 out]
                    n431 = call-poly <userlib>:"Build Path__ogtk.vi"("name or relative path"=w1115, "base path"=w1117) -> ("appended path"=w1111:path)
                    n432 = local write "Down hole Pressure Transducer CSV data  path 2"(w1111) -> ()
                    n433 = call-poly <vilib>:"Write Delimited Spreadsheet.vi"("file path (dialog if empty)"=w1111, "1D data"=w1126, "append to file? (new file:F)"=TRUE, "error in (no error)"=w1114, "delimiter (\\t)"="," ("delimiter (\\t)")) -> ("error out"=w1113:errorcluster)  [unwired: 9 in, 1 out]
                  }
                }
                n434 = local read "Corrected Pressure Cluster"() -> (w1084:T20)
                n435 = Bundle By Name(cluster=w1084, "Down hole Corrected Pressure"=w1083) -> (w1085:T20)
                n436 = local write "Corrected Pressure Cluster"(w1085) -> ()
              }
            }
            n437 = flat-sequence {
              tunnel: w964 -> [w1077]
              tunnel: [w1073] -> w963
              tunnel: [w1072] -> w962
              frame #0 {
                n438 = local read "Input Variables and Slopes"() -> (w1080:T1)
                n439 = Unbundle By Name(w1080) -> ("Up Hole Pressure Slope"=w1079:dbl, "Up Hole  Pressure Offset"=w1076:dbl)
                n440 = local write "Input Variables and Slopes"(w1080) -> ()
                n441 = local read "Sensor Voltage Cluster"() -> (w1081:T10)
                n442 = local read "Descriptions"() -> (w1073:string[])
                n443 = local read "Corrected Pressure Cluster"() -> (w1075:T20)
                n444 = call "up hole Pressure 2016.vi"("Sensor Cluster"=w1081, "Pressure Offset"=w1076, "Array in"=w1077, "Pressure \nSlope"=w1079, "Descriptions"=w1073, "Zero Pressure\n(F = leave as is)"=TRUE) -> ("Array out"=w1072:refnum<k24>[], "Uphole Pressure"=w1071:dbl, "Sensor Cluster 2"=w1078:T10)  [unwired: 6 in, 1 out]
                n445 = Bundle By Name(cluster=w1075, "Up hole Corrected Pressure"=w1071) -> (w1074:T20)
                n446 = local write "Sensor Voltage Cluster"(w1078) -> ()
                n447 = local write "Corrected Pressure Cluster"(w1074) -> ()
                n448 = local write "Uphole Pressure"(w1071) -> ()
              }
            }
            n449 = flat-sequence {
              tunnel: w963 -> [w1064]
              tunnel: w962 -> [w1067]
              tunnel: [w1062] -> w959
              tunnel: [w1064] -> w961
              tunnel: [w1063] -> w956
              tunnel: [w1061] -> w954
              frame #0 {
                w1068 = 0.0  # Offset
                n450 = local read "Input Variables and Slopes"() -> (w1066:T1)
                n451 = Unbundle By Name(w1066) -> ("Flow Slope"=w1065:dbl)
                n452 = local read "Input Depths \nand Parameters Cluster"() -> (w1070:T16)
                n453 = call "Flow 2016.vi"("Descriptions"=w1064, "Array in"=w1067, "Flow Slope"=w1065, "Offset"=w1068) -> ("Sensor Cluster"=w1062:T10, "Flow (ml/min)"=w1063:dbl, "Array out"=w1061:refnum<k24>[])  [unwired: 4 in]
                n454 = local write "Sensor Voltage Cluster"(w1062) -> ()
                n455 = Bundle By Name(cluster=w1070, "Flow"=w1063) -> (w1069:T16)
                n456 = local write "Input Depths \nand Parameters Cluster"(w1069) -> ()
              }
            }
            n457 = flat-sequence {
              tunnel: w961 -> [w1044]
              tunnel: w960 -> [w1014]
              tunnel: w959 -> [w1043]
              tunnel: w958 -> [w1000]
              tunnel: [w1042] -> w957
              tunnel: w956 -> [w1041]
              tunnel: w954 -> [w1035]
              tunnel: [w1034] -> _
              tunnel: [w1007] -> w953
              tunnel: w946 -> [w1030]
              tunnel: w945 -> [w1023]
              tunnel: [w1006] -> w943
              tunnel: w942 -> [w1012]
              tunnel: w941 -> [w1002]
              tunnel: [w1001] -> w940
              frame #0 {
                n458 = Unbundle By Name(w1000) -> ("Current Relative Depth"=w1024:dbl)
                n459 = Unbundle By Name(w1000) -> ("Current Absolute Depth"=w999:dbl)
                n460 = local read "Input Depths \nand Parameters Cluster"() -> (w1026:T16)
                n461 = Unbundle By Name(w1026) -> ("Start Depth"=w1025:sgl)
                n462 = global read "Kpro Globals.vi" "increment_amount"() -> (w1028:dbl)
                n463 = local read "Culmulative Graph Cluster"() -> (w1033:T19)
                n464 = local read "Input Depths \nand Parameters Cluster"() -> (w1038:T16)
                n465 = Equal?(x=w999, y=w1025) -> (x = y?=w1020:bool)
                n466 = And(x=w1020, y=FALSE) -> (x .and. y?=w1021:bool)
                n467 = First Call?() -> ()  [unwired: 1 out]
                n468 = local read "Input Variables and Slopes"() -> (w1040:T1)
                n469 = local read "Uphole Pressure"() -> (w1003:dbl)
                n470 = local read "KPRO Finish\nIndicator"() -> (w1027:bool)
                n471 = local read "Depth mode"() -> (w1011:bool)
                n472 = case shown="True" w1021 {
                  tunnel: w1024 -> [w1048 w1049]
                  tunnel: [w1047 w1049] -> w1029
                  tunnel: w1028 -> [w1046 _]
                  frame False {
                    n473 = Add(x=w1046, y=w1048) -> (x+y=w1047:dbl)
                  }
                  frame True {
                  }
                }
                n474 = Unbundle By Name(w1038) -> ()  [unwired: 2 out]
                n475 = Unbundle By Name(w1040) -> ("String Pot Slope"=w1039:dbl)
                n476 = call "Kpro Read String Pot 2016.vi"("Read String Pot"=w1011, "Feet of\nStainless to be\nUsed (Count) in"=w1002, "Session Array in"=w1012, "Flow"=w1041, "Manual Depth In"=w1029, "Finished In"=w1027, "Depth Cluster in"=w1000, "error in (no error)"=w1030, "String Pot \nSlope in"=w1039, "Sensor Cluster In in"=w1043, "Descriptions"=w1044, "Pressure in"=w1003, "Array in"=w1035, "Downhole Pressure Sensor"=w1023, "Initial Measurement Input"=FALSE) -> ("Sensor Cluster 2"=w1036:T10, "IK"=w1013:dbl, "Array out"=w1034:refnum<k24>[], "Generate Array Calc IK"=w996:bool, "Depth Rate"=→"Depth Rate\nft/min":dbl, "Feet of\nStainless to be\nUsed (Count) out"=w1001:i32, "Depth Cluster out"=w1042:T17, "Single String Pot Session Array out"=w1006:dbl[][])  [unwired: 4 in, 1 out]
                "Ik" <- w1013
                n477 = And(x=w1011, y=w996) -> ()  [unwired: 1 out]
                n478 = local write "Sensor Voltage Cluster"(w1036) -> ()
                n479 = Unbundle By Name(w1042) -> ("Current Absolute Depth"=w1016:dbl)
                n480 = Bundle By Name(cluster=w1038, "Feet of Stainless"=w1001) -> (w1037:T16)
                n481 = local write "Ik"(w1013) -> ()
                n482 = local write "Input Depths \nand Parameters Cluster"(w1037) -> ()
                n483 = flat-sequence {
                  tunnel: w1016 -> [w1054]
                  frame #0 {
                    n484 = local read "Corrected Pressure Cluster"() -> (w1057:T20)
                    n485 = global write "Kpro Globals.vi" "Current Depth"(w1054) -> ()
                    n486 = local write "Current Depth"(w1054) -> ()
                    n487 = Divide(x=w1054, y=3.281) -> (x/y=w1055:dbl)
                    n488 = local read "Sample Sheet Data Row Cluster 2"() -> (w1059:T3)
                    n489 = local write "Current \nDepth (m)"(w1055) -> ()
                    n490 = Unbundle By Name(w1057) -> ("Up hole Corrected Pressure"=w1056:dbl)
                    n491 = Bundle By Name(cluster=w1059, "Depth"=w1054, "Head\nPressure"=w1056) -> (w1058:T3)
                    n492 = local write "Sample Sheet Data Row Cluster 2"(w1058) -> ()
                  }
                }
                n493 = case shown="True" FALSE {
                  tunnel: w1006 -> [_ w1051]
                  tunnel: [w1050 w1052] -> w1007
                  tunnel: w1014 -> [w1050 w1053]
                  frame False {
                  }
                  frame True {
                    n494 = Build Array (concatenate)(w1053, w1051) -> (w1052:dbl[][])
                  }
                }
                n495 = call "Array to Plot 2016.vi"("Input Cumulative Array"=w1007, "Input Real Time Array"=w1006) -> ("Cumulative - Depth vs.Drive Rate"=w1004:cluster{dbl[], dbl[]}, "Cumulative - Depth vs. Ik"=w1031:cluster{dbl[], dbl[]}, "Real Time - Depth vs. Drive Rate"=w1005:cluster{dbl[], dbl[]}, "Real Time - Depth vs. Ik"=w1018:cluster{dbl[], dbl[]}, "Depth Rate"=w1015:dbl)  [unwired: 2 in, 1 out]
                n496 = Bundle By Name(cluster=w1033, "Cumulative - Depth vs. Ik"=w1031, "Real Time - Depth vs. lk"=w1018, "Cumulative - Depth vs. Drive Rate"=w1004, "Real Time - Depth vs. Drive Rate"=w1005) -> (w1032:T19)
                n497 = local write "Culmulative Graph Cluster"(w1032) -> ()
                n498 = local write "Large Depth IK Graph Cluster"(w1018) -> ()
                n499 = local write "Depth Rate\nft/min"(w1015) -> ()
                n500 = control-ref of="KPRO Cumulative Output File Path"() -> (w997:refnum<vi>)
                n501 = control-ref of="KPRO SessionOutput File Path"() -> (w1008:refnum<vi>)
                n502 = call "write KPRO file.vi"("Corrected Array in"=w1006, "Generate Array Calc IK"=w996, "Path in"=w1008) -> ("paths ok"=w1019:bool, "appended path"=w1022:path)  [unwired: 7 in]
                n503 = case shown="True" w1019 {
                  tunnel: w1022 -> [_ w1045]
                  frame False {
                  }
                  frame True {
                    n504 = local write "KPRO SessionOutput File Path"(w1045) -> ()
                  }
                }
                n505 = call "write KPRO file.vi"("Corrected Array in"=w1007, "Generate Array Calc IK"=w996, "Path in"=w997) -> ()  [unwired: 7 in, 2 out]
                n506 = local write "Current Session"(w1006) -> ()
                n507 = local write "Cumulative_data_from_file"(w1007) -> ()
              }
            }
          }
          frame "Sample Not Collected" {
            n508 = local write "Tab Control"(T4."Recording Reason Sonde" ("Tab Control")) -> ()
          }
          frame "Record Sonde Reason" {
            n509 = flat-sequence {
              tunnel: w1145 -> [w1162]
              tunnel: [w1161] -> w1144
              frame #0 {
                n510 = local read "Sample Sheet Data Row Cluster 2"() -> (w1184:T3)
                n511 = local read "KPRO SessionOutput File Path"() -> (w1180:path)
                n512 = local write "Tab Control"(T4."Recording Reason Sonde" ("Tab Control")) -> ()
                n513 = property on="Select Reasons to Record Data" class="Ring (strict)"() -> ("Strings []"=w1172:string[])  [unwired: 2 in, 2 out]
                n514 = Get Date/Time In Seconds() -> (seconds since 1Jan1904=w1183:timestamp)
                n515 = Unbundle By Name(w1184) -> ("Head\nPressure"=w1182:dbl, "Depth"=w1181:dbl)
                n516 = call-poly <userlib>:"Strip Path Extension__ogtk.vi"("path"=w1180) -> ("root"=w1179:string)  [unwired: 1 out]
                n517 = local read "Recording Reason Sonde array"() -> (w1166:string[][])
                n518 = call-poly <userlib>:"Convert File Extension__ogtk.vi"("new ending (none)"="_Sample failure.csv", "file name"=w1179) -> ("new filename"=w1178:string)  [unwired: 1 out]
                n519 = Index Array(array=w1172, index="Select Reasons to Record Data") -> (element=w1170:string)
                n520 = Format Date/Time String(seconds (now)=w1183) -> (date/time string=w1176:string)  [unwired: 2 in]
                n521 = Format Into String(w1182) -> (resulting string=w1175:string)  [unwired: 3 in, 1 out]
                n522 = Format Into String(w1181) -> (resulting string=w1174:string)  [unwired: 3 in, 1 out]
                n523 = Format Into String("Select Reasons to Record Data") -> (resulting string=w1173:string)  [unwired: 3 in, 1 out]
                n524 = Build Array(w1176, w1175, w1174, w1173, w1170) -> (w1164:string[])
                n525 = String To Path(string=w1178) -> (path=w1163:path)
                "Sonde Recording Failure Path" <- w1163
                n526 = Build Array (concatenate)(w1166, w1164) -> (→"Recording Reason Sonde array":string[][])
                n527 = call-poly <vilib>:"Write Delimited Spreadsheet.vi"("file path (dialog if empty)"=w1163, "1D data"=w1164, "append to file? (new file:F)"=TRUE, "error in (no error)"=w1162, "delimiter (\\t)"="," ("delimiter (\\t)")) -> ("error out"=w1161:errorcluster)  [unwired: 9 in, 1 out]
                n528 = local write "Sonde Recording Error file"(w1163) -> ()
              }
            }
          }
          frame "Record IK Reason" {
            n529 = flat-sequence {
              frame #0 {
                n530 = local read "Select Entry for IK Log File"() -> (w1206:u16)
                n531 = property on="Select Entry for IK Log File" class="Ring (strict)"() -> ("Strings []"=w1205:string[])  [unwired: 2 in, 2 out]
                n532 = local read "Sample Sheet Data Row Cluster 2"() -> (w1222:T3)
                n533 = local read "KPRO SessionOutput File Path"() -> (w1218:path)
                n534 = local write "Tab Control"(T4."Pressure/Flow/IK Graphs" ("Tab Control")) -> ()
                n535 = Get Date/Time In Seconds() -> (seconds since 1Jan1904=w1221:timestamp)
                n536 = Unbundle By Name(w1222) -> ("Head\nPressure"=w1220:dbl, "Depth"=w1219:dbl)
                n537 = call-poly <userlib>:"Strip Path Extension__ogtk.vi"("path"=w1218) -> ("root"=w1217:string)  [unwired: 1 out]
                n538 = call-poly <userlib>:"Convert File Extension__ogtk.vi"("new ending (none)"="_IK Behavior.csv", "file name"=w1217) -> ("new filename"=w1215:string)  [unwired: 1 out]
                n539 = Index Array(array=w1205, index=w1206) -> (element=w1209:string)
                n540 = Format Date/Time String(seconds (now)=w1221) -> (date/time string=w1213:string)  [unwired: 2 in]
                n541 = local read "IK Reason array"() -> (w1201:string[][])
                n542 = Format Into String(w1220) -> (resulting string=w1212:string)  [unwired: 3 in, 1 out]
                n543 = Format Into String(w1219) -> (resulting string=w1211:string)  [unwired: 3 in, 1 out]
                n544 = Format Into String(w1206) -> (resulting string=w1210:string)  [unwired: 3 in, 1 out]
                n545 = Build Array(w1213, w1212, w1211, w1210, w1209) -> (w1208:string[])
                n546 = String To Path(string=w1215) -> (path=w1216:path)
                "Sonde IK Behavior Path" <- w1216
                n547 = Build Array (concatenate)(w1201, w1208) -> (→"IK Reason array":string[][])
                n548 = call-poly <vilib>:"Write Delimited Spreadsheet.vi"("file path (dialog if empty)"=w1216, "1D data"=w1208, "append to file? (new file:F)"=TRUE, "delimiter (\\t)"="," ("delimiter (\\t)")) -> ()  [unwired: 10 in, 2 out]
              }
            }
          }
          frame "Continuous  Sonde Data" {
            n549 = local read "Found Quanta Sonde Com Port"() -> (w1245:refnum<visa-resource-name>)
            n550 = control-ref of="Sonde Data Display"() -> (w1248:refnum<vi>)
            n551 = local read "Sample Sheet Data Row Cluster 2"() -> (w1226:T3)
            n552 = Unbundle By Name(w1226) -> ("Sonde Data Cluster.Cumulative\nVolume (ml)"=w1225:dbl)
            n553 = call "SDI-12 Continuous Operations.vi"("RS232 Port In"=w1245, "Sensor Address In"="0", "Sonde Data Ctl Refnum"=w1248, "Error In (No Error)"=w1247) -> ("output cluster"=w1224:T2, "Temperature"=w1243:cluster{"Y":dbl[], "Y":dbl[]}[], "Sonde Data Display"=w1242:T14, "Error Out"=w1246:errorcluster)  [unwired: 8 in, 4 out]
            n554 = Bundle By Name(cluster=w1224, "Cumulative\nVolume (ml)"=w1225) -> (w1223:T2)
            n555 = Bundle By Name(cluster=w1226, "Sonde Data Cluster"=w1223) -> (w1244:T3)
            n556 = local write "Temperature"(w1243) -> ()
            n557 = local write "Sonde Data Display"(w1242) -> ()
            n558 = local write "Sample Sheet Data Row Cluster 2"(w1244) -> ()
          }
          frame "Acq. Single Sonde Point" {
            n559 = invoke on="Record Single Sample" class="Bool" method="Reinit To Default"(error in=w1277) -> (error out=w1276:errorcluster)  [unwired: 2 in, 2 out]
            n560 = flat-sequence {
              tunnel: w1285 -> [w1343]
              tunnel: [w1336] -> _
              tunnel: w1286 -> [w1341]
              tunnel: [w1340] -> w1284
              tunnel: [w1339] -> _
              tunnel: [w1338] -> w1280
              tunnel: w1287 -> [w1336]
              frame #0 {
                n561 = Array Subset(array=w1336, index (col)=2 ("index")) -> (w1332:string[][])  [unwired: 3 in]
                n562 = local write "subarray"(w1332) -> ()
                n563 = local read "Current Sample Sheet"() -> (w1335:string)
                n564 = call "find last occupied cell.vi"("data"=w1336, "Active Sheet"=w1335, "Header Rows to remove"=3, "sub array start"=w1341, "error in (no error)"=w1343) -> ("row max value"=w1339:i32, "column max value"=w1334:i32, 13:"start of last occupied row"=w1338:cluster{"row":i32, "column":i32}, 14:"start of last occupied row"=w1333:string, "error out"=w1340:errorcluster)  [unwired: 4 in, 2 out]
                n565 = local write "last occupied cell's name"(w1333) -> ()
                n566 = local write "row max value"(w1334) -> ()
              }
            }
            n567 = call <vilib>:"Clear Errors.vi"("error in (no error)"=w1276) -> ("error out"=w1266:errorcluster)  [unwired: 5 in, 1 out]
            n568 = call "get sample sheet data cells.vi"("error in (no error)"=w1266, "NI_report in"=w1288) -> ("error out"=w1285:errorcluster, "data"=w1287:string[][], "NI_report out"=w1281:refnum<class "NI_report.lvclass">, "left edge output cluster"=w1286:cluster{"row":i32, "column":i32})  [unwired: 5 in, 1 out]
            n569 = flat-sequence {
              tunnel: w1284 -> [w1316]
              tunnel: [w1315] -> w1252
              tunnel: w1272 -> [w1314]
              tunnel: [w1313] -> w1271
              tunnel: [w1312] -> w1270
              tunnel: w1269 -> [w1311]
              tunnel: [w1302] -> w1262
              tunnel: [w1310] -> w1258
              tunnel: w1256 -> [w1309]
              frame #0 {
                n570 = local read "Sample Sheet Data Row Cluster 2"() -> (w1301:T3)
                n571 = control-ref of="Found Quanta Sonde Com Port"() -> (w1308:refnum<vi>)
                n572 = control-ref of="Current Time (s)"() -> (w1304:refnum<vi>)
                n573 = control-ref of="Sonde Data Display"() -> (w1307:refnum<vi>)
                n574 = control-ref of="Sonde Data Display"() -> (w1306:refnum<vi>)
                n575 = local write "Tab Control"(T4."Sonde Data" ("Tab Control")) -> ()
                n576 = control-ref of="Temperature"() -> (w1305:refnum<vi>)
                n577 = call "Sonde Single Measurement Subvi.vi"("VISAResourceName in"=w1308, "Time Array"=w1314, "Cumulative Sonde Data"=w1311, "Previous time"=w1309, "Sonde Data Display"=w1307, "Sonde Graph in"=w1306, "Temp Graph 3"=w1305, "error in (no error)"=w1316, "Row Cluster Input"=w1301, "reference 5"=w1304) -> ("seconds since 1Jan1904"=w1310:timestamp, "Cumulative Sonde \nData Out"=w1312:dbl[][], "Sample Sheet Data Row Cluster 2"=w1302:T3, "output cluster"=→"output cluster":T2, "time array out"=w1313:dbl[], "error out"=w1315:errorcluster)
                n578 = local write "Sample Sheet Data Row Cluster 2"(w1302) -> ()
              }
            }
            n579 = flat-sequence {
              tunnel: w1262 -> [w1299]
              tunnel: w1261 -> [w1296]
              tunnel: w1259 -> [w1293]
              tunnel: [w1291] -> w1254
              tunnel: w1252 -> [w1290]
              tunnel: [w1289] -> w1251
              frame #0 {
                n580 = local read "Sonde Data Array"() -> (w1295:T12[])
                n581 = call "populate sonde row cluster from sonde data cluster.vi"("Initialize \nInitial Value \nCluster"=TRUE ("Initialize \nInitial Value \nCluster"), "error in (no error)"=w1290, "Sonde Parameters \nInitial Values"=w1296, "Sample Sheet Data Row Cluster"=w1299, "Sonde Parameters \nTolerance Limits"="Sonde Parameters \nTolerance Limits") -> ("error out"=w1289:errorcluster, "Cluster"=w1292:T12, "Sonde Parameters \nInitial Values Out"=w1291:T6)  [unwired: 4 in]
                n582 = Insert Into Array(array=w1295, index=w1293, new element=w1292) -> (w1294:T12[])
                n583 = local write "Sonde Parameters \nInitial Values"(w1291) -> ()
                n584 = local write "Sonde Data Array"(w1294) -> ()
              }
            }
            n585 = To Double Precision Float(number=w1258) -> ()  [unwired: 1 out]
            n586 = call "write out sonde row.vi"("NI_report in"=w1281, "Columns"=w1283, "Column of Volume"=w1282, "Sample Sheet Data Row Cluster"=w1262, "row index"=w1259, "error in (no error)"=w1251, "start of last occupied row"=w1280) -> ("NI_report out"=w1279:refnum<class "NI_report.lvclass">, "row index out"=w1273:i32, "error out"=w1250:errorcluster)  [unwired: 6 in]
            n587 = flat-sequence {
              tunnel: w1250 -> [w1331]
              tunnel: w1279 -> [w1330]
              tunnel: [w1329] -> w1278
              tunnel: [w1324] -> w1275
              tunnel: [w1322] -> w1274
              frame #0 {
                n588 = local read "Current Sample Sheet"() -> (w1320:string)
                n589 = call <vilib>:"Clear Errors.vi"("error in (no error)"=w1331) -> ("error out"=w1318:errorcluster)  [unwired: 5 in, 1 out]
                n590 = call "get sample sheet data cells.vi"("error in (no error)"=w1318, "NI_report in"=w1330) -> ("error out"=w1325:errorcluster, "data"=w1326:string[][], "NI_report out"=w1329:refnum<class "NI_report.lvclass">, "left edge output cluster"=w1323:cluster{"row":i32, "column":i32})  [unwired: 5 in, 1 out]
                n591 = call "find last occupied cell.vi"("data"=w1326, "Active Sheet"=w1320, "Header Rows to remove"=3, "sub array start"=w1323, "error in (no error)"=w1325) -> ("row max value"=w1321:i32, 13:"start of last occupied row"=w1322:cluster{"row":i32, "column":i32}, 14:"start of last occupied row"=w1319:string, "error out"=w1324:errorcluster)  [unwired: 4 in, 3 out]
                n592 = Array Subset(array=w1326, index (col)=2 ("index")) -> (w1317:string[][])  [unwired: 3 in]
                n593 = local write "row max value"(w1321) -> ()
                n594 = local write "last occupied cell's name"(w1319) -> ()
                n595 = local write "subarray"(w1317) -> ()
              }
            }
          }
          frame "pH Calibration Zero" {
            n596 = invoke on="Record Single Sample" class="Bool" method="Reinit To Default"(error in=w1364) -> (error out=w1363:errorcluster)  [unwired: 2 in, 2 out]
            n597 = call <vilib>:"Clear Errors.vi"("error in (no error)"=w1363) -> ("error out"=w1351:errorcluster)  [unwired: 5 in, 1 out]
            n598 = call "get sample sheet data cells.vi"("error in (no error)"=w1351, "NI_report in"=w1382) -> ("error out"=w1379:errorcluster, "data"=w1381:string[][], "NI_report out"=w1374:refnum<class "NI_report.lvclass">, "left edge output cluster"=w1380:cluster{"row":i32, "column":i32})  [unwired: 5 in, 1 out]
            n599 = flat-sequence {
              tunnel: w1379 -> [w1444]
              tunnel: [w1438] -> _
              tunnel: w1380 -> [w1442]
              tunnel: [w1441] -> w1378
              tunnel: [w1440] -> _
              tunnel: [w1439] -> w1372
              tunnel: w1381 -> [w1438]
              frame #0 {
                n600 = local read "Current Sample Sheet"() -> (w1437:string)
                n601 = call "find last occupied cell.vi"("data"=w1438, "Active Sheet"=w1437, "Header Rows to remove"=3, "sub array start"=w1442, "error in (no error)"=w1444) -> ("row max value"=w1440:i32, "column max value"=w1436:i32, 13:"start of last occupied row"=w1439:cluster{"row":i32, "column":i32}, 14:"start of last occupied row"=w1435:string, "error out"=w1441:errorcluster)  [unwired: 4 in, 2 out]
                n602 = local write "row max value"(w1436) -> ()
                n603 = local write "last occupied cell's name"(w1435) -> ()
              }
            }
            n604 = local read "Found Quanta Sonde Com Port"() -> (w1368:refnum<visa-resource-name>)
            n605 = Equal?(x=w1368, y=refnum<visa-resource-name> refnum ("RS232 Port Out")) -> (x = y?=w1370:bool)
            n606 = case shown="False" w1370 {
              tunnel: w1368 -> [w1400 _]
              tunnel: [w1408 w1431] -> w1371
              tunnel: w1378 -> [w1402 w1434]
              tunnel: [w1411 w1434] -> w1375
              tunnel: w1358 -> [w1407 w1433]
              tunnel: [w1406 w1421] -> w1357
              tunnel: [w1405 w1420] -> w1356
              tunnel: w1355 -> [w1404 w1432]
              tunnel: w1354 -> [_ w1417]
              frame False {
                w1403 = "0" ("Sensor Address In")
                n607 = control-ref of="Sonde Data Display"() -> (w1412:refnum<vi>)
                n608 = local read "Sample Sheet Data Row Cluster 2"() -> (w1409:T3)
                n609 = call "Calibrate pH Sensor.vi"("Calibration Standard"="pH Zero", "Error In (No Error)"=w1402, "Sensor Address In"=w1403, "RS232 Port In"=w1400) -> ("Error Out"=w1401:errorcluster, "Sensor Calibrate Response"=→"pH Zero \nCalibrate Response":bool, "RS232 Port Out"=w1399:refnum<visa-resource-name>)  [unwired: 3 in, 2 out]
                n610 = call "SDI-12 Single Operation with output cluster.vi"("RS232 Port In"=w1399, "Sensor Address In"=w1403, "Sonde Data Ctl Refnum"=w1412, "Error In (No Error)"=w1401, "Time Array In"=w1407, "Measurement Array In"=w1404) -> ("time array out"=w1406:dbl[], "Measurement  array Out"=w1405:dbl[][], "output cluster"=w1410:T2, "Temperature"=w1414:cluster{"Y":dbl[], "Y":dbl[]}[], "Sonde Data Display"=w1413:T14, "Error Out"=w1411:errorcluster)  [unwired: 12 in, 4 out]
                n611 = local write "Temperature"(w1414) -> ()
                n612 = local write "Sonde Data Display"(w1413) -> ()
                n613 = Bundle By Name(cluster=w1409, "Sonde Data Cluster"=w1410) -> (w1408:T3)
              }
              frame True {
                n614 = Get Date/Time In Seconds() -> (seconds since 1Jan1904=w1423:timestamp)
                n615 = To Double Precision Float(number=w1423) -> (double precision float=w1422:dbl)
                n616 = local read "Sample Sheet Data Row Cluster 2"() -> (w1431:T3)
                n617 = Subtract(x=w1422, y=w1417) -> (x-y=w1415:dbl)
                n618 = local write "Current Time (s)"(w1415) -> ()
                n619 = Unbundle By Name(w1431) -> ("Sonde Data Cluster.Temp\ndeg C"=w1416:dbl, "Sonde Data Cluster.pH"=w1430:dbl, "Sonde Data Cluster.Specific\nCond (mS)"=w1429:dbl, "Sonde Data Cluster.Salinity"=w1428:dbl, "Sonde Data Cluster.Dissolved\nOxygen mg/L"=w1427:dbl, "Sonde Data Cluster.ORP"=w1426:dbl)  [unwired: 1 out]
                n620 = Build Array(w1416, w1430, w1429, w1428, w1427, 0.0 ("element"), w1426) -> (w1424:dbl[])
                n621 = Build Array (concatenate)(w1432, w1424) -> (w1420:dbl[][])
                n622 = Build Array (concatenate)(w1433, w1415) -> (w1421:dbl[])
                n623 = call "format into Sonde Vertical Graph Data Input.vi"("Sonde Measurement Array"=w1420, "Time Array"=w1421) -> ("Sonde Data Display"=w1419:T14, "Temperature"=w1418:cluster{"X":dbl[], "Y":dbl[]}[])  [unwired: 8 in]
                n624 = local write "Temperature"(w1418) -> ()
                n625 = local write "Sonde Data Display"(w1419) -> ()
              }
            }
            n626 = local write "Sample Sheet Data Row Cluster 2"(w1371) -> ()
            n627 = call "write out sonde row.vi"("NI_report in"=w1374, "Columns"=w1377, "Column of Volume"=w1376, "Sample Sheet Data Row Cluster"=w1371, "row index"=w1360, "error in (no error)"=w1375, "start of last occupied row"=w1372) -> ("NI_report out"=w1366:refnum<class "NI_report.lvclass">, "row index out"=w1359:i32, "error out"=w1367:errorcluster)  [unwired: 6 in]
            n628 = flat-sequence {
              tunnel: w1367 -> [w1396]
              tunnel: w1366 -> [w1395]
              tunnel: [w1394] -> w1365
              tunnel: [w1389] -> w1362
              tunnel: [w1387] -> w1361
              frame #0 {
                (unwired) 3 ("Header Rows to remove")
                n629 = call <vilib>:"Clear Errors.vi"("error in (no error)"=w1396) -> ("error out"=w1383:errorcluster)  [unwired: 5 in, 1 out]
                n630 = local read "Current Sample Sheet"() -> (w1385:string)
                n631 = call "get sample sheet data cells.vi"("error in (no error)"=w1383, "NI_report in"=w1395) -> ("error out"=w1390:errorcluster, "data"=w1391:string[][], "NI_report out"=w1394:refnum<class "NI_report.lvclass">, "left edge output cluster"=w1388:cluster{"row":i32, "column":i32})  [unwired: 5 in, 1 out]
                n632 = call "find last occupied cell.vi"("data"=w1391, "Active Sheet"=w1385, "Header Rows to remove"=3, "sub array start"=w1388, "error in (no error)"=w1390) -> ("row max value"=w1386:i32, 13:"start of last occupied row"=w1387:cluster{"row":i32, "column":i32}, 14:"start of last occupied row"=w1384:string, "error out"=w1389:errorcluster)  [unwired: 4 in, 3 out]
                n633 = Array Subset(array=w1391, index (col)=2 ("index")) -> ()  [unwired: 3 in, 1 out]
                n634 = local write "row max value"(w1386) -> ()
                n635 = local write "last occupied cell's name"(w1384) -> ()
              }
            }
          }
          frame "pH Calibration Standard" {
            n636 = invoke on="Record Single Sample" class="Bool" method="Reinit To Default"(error in=w1465) -> (error out=w1464:errorcluster)  [unwired: 2 in, 2 out]
            n637 = call <vilib>:"Clear Errors.vi"("error in (no error)"=w1464) -> ("error out"=w1452:errorcluster)  [unwired: 5 in, 1 out]
            n638 = call "get sample sheet data cells.vi"("error in (no error)"=w1452, "NI_report in"=w1483) -> ("error out"=w1480:errorcluster, "data"=w1482:string[][], "NI_report out"=w1475:refnum<class "NI_report.lvclass">, "left edge output cluster"=w1481:cluster{"row":i32, "column":i32})  [unwired: 5 in, 1 out]
            n639 = flat-sequence {
              tunnel: w1480 -> [w1547]
              tunnel: [w1540] -> _
              tunnel: w1481 -> [w1545]
              tunnel: [w1544] -> w1479
              tunnel: [w1543] -> _
              tunnel: [w1542] -> w1473
              tunnel: w1482 -> [w1540]
              frame #0 {
                n640 = Array Subset(array=w1540, index (col)=2 ("index")) -> ()  [unwired: 3 in, 1 out]
                n641 = local read "Current Sample Sheet"() -> (w1539:string)
                n642 = call "find last occupied cell.vi"("data"=w1540, "Active Sheet"=w1539, "Header Rows to remove"=3, "sub array start"=w1545, "error in (no error)"=w1547) -> ("row max value"=w1543:i32, "column max value"=w1538:i32, 13:"start of last occupied row"=w1542:cluster{"row":i32, "column":i32}, 14:"start of last occupied row"=w1537:string, "error out"=w1544:errorcluster)  [unwired: 4 in, 2 out]
                n643 = local write "last occupied cell's name"(w1537) -> ()
                n644 = local write "row max value"(w1538) -> ()
              }
            }
            n645 = local read "Found Quanta Sonde Com Port"() -> (w1469:refnum<visa-resource-name>)
            n646 = Equal?(x=w1469, y=refnum<visa-resource-name> refnum ("RS232 Port Out")) -> (x = y?=w1471:bool)
            n647 = case shown="False" w1471 {
              tunnel: w1469 -> [w1499 _]
              tunnel: [w1509 w1533] -> w1472
              tunnel: w1479 -> [w1502 w1536]
              tunnel: [w1512 w1536] -> w1476
              tunnel: w1459 -> [w1508 w1535]
              tunnel: [w1507 w1523] -> w1458
              tunnel: [w1506 w1522] -> w1457
              tunnel: w1456 -> [w1505 w1534]
              tunnel: w1455 -> [_ w1519]
              frame False {
                n648 = control-ref of="Sonde Data Display"() -> (w1513:refnum<vi>)
                n649 = call "Calibrate pH Sensor.vi"("Calibration Standard"="pH Reference", "Error In (No Error)"=w1502, "Sensor Address In"="0", "RS232 Port In"=w1499) -> ("Error Out"=w1501:errorcluster, "Sensor Calibrate Response"=→"pH  Reference\nCalibrate Response":bool, "RS232 Port Out"=w1498:refnum<visa-resource-name>)  [unwired: 3 in, 2 out]
                n650 = local read "Sample Sheet Data Row Cluster 2"() -> (w1510:T3)
                n651 = call "SDI-12 Single Operation with output cluster.vi"("RS232 Port In"=w1498, "Sensor Address In"="0", "Sonde Data Ctl Refnum"=w1513, "Error In (No Error)"=w1501, "Time Array In"=w1508, "Measurement Array In"=w1505) -> ("time array out"=w1507:dbl[], "Measurement  array Out"=w1506:dbl[][], "output cluster"=w1511:T2, "Temperature"=w1515:cluster{"Y":dbl[], "Y":dbl[]}[], "Sonde Data Display"=w1514:T14, "Error Out"=w1512:errorcluster)  [unwired: 12 in, 4 out]
                n652 = Bundle By Name(cluster=w1510, "Sonde Data Cluster"=w1511) -> (w1509:T3)
                n653 = local write "Temperature"(w1515) -> ()
                n654 = local write "Sonde Data Display"(w1514) -> ()
              }
              frame True {
                n655 = Get Date/Time In Seconds() -> (seconds since 1Jan1904=w1525:timestamp)
                n656 = To Double Precision Float(number=w1525) -> (double precision float=w1524:dbl)
                n657 = local read "Sample Sheet Data Row Cluster 2"() -> (w1533:T3)
                n658 = Subtract(x=w1524, y=w1519) -> (x-y=w1517:dbl)
                n659 = local write "Current Time (s)"(w1517) -> ()
                n660 = Unbundle By Name(w1533) -> ("Sonde Data Cluster.Temp\ndeg C"=w1518:dbl, "Sonde Data Cluster.pH"=w1532:dbl, "Sonde Data Cluster.Specific\nCond (mS)"=w1531:dbl, "Sonde Data Cluster.Salinity"=w1530:dbl, "Sonde Data Cluster.Dissolved\nOxygen mg/L"=w1529:dbl, "Sonde Data Cluster.ORP"=w1528:dbl)  [unwired: 1 out]
                n661 = Build Array(w1518, w1532, w1531, w1530, w1529, 0.0 ("element"), w1528) -> (w1526:dbl[])
                n662 = Build Array (concatenate)(w1534, w1526) -> (w1522:dbl[][])
                n663 = Build Array (concatenate)(w1535, w1517) -> (w1523:dbl[])
                n664 = call "format into Sonde Vertical Graph Data Input.vi"("Sonde Measurement Array"=w1522, "Time Array"=w1523) -> ("Sonde Data Display"=w1521:T14, "Temperature"=w1520:cluster{"X":dbl[], "Y":dbl[]}[])  [unwired: 8 in]
                n665 = local write "Temperature"(w1520) -> ()
                n666 = local write "Sonde Data Display"(w1521) -> ()
              }
            }
            n667 = local write "Sample Sheet Data Row Cluster 2"(w1472) -> ()
            n668 = call "write out sonde row.vi"("NI_report in"=w1475, "Columns"=w1478, "Column of Volume"=w1477, "Sample Sheet Data Row Cluster"=w1472, "row index"=w1461, "error in (no error)"=w1476, "start of last occupied row"=w1473) -> ("NI_report out"=w1467:refnum<class "NI_report.lvclass">, "row index out"=w1460:i32, "error out"=w1468:errorcluster)  [unwired: 6 in]
            n669 = flat-sequence {
              tunnel: w1468 -> [w1497]
              tunnel: w1467 -> [w1496]
              tunnel: [w1495] -> w1466
              tunnel: [w1490] -> w1463
              tunnel: [w1488] -> w1462
              frame #0 {
                (unwired) 3 ("Header Rows to remove")
                n670 = call <vilib>:"Clear Errors.vi"("error in (no error)"=w1497) -> ("error out"=w1484:errorcluster)  [unwired: 5 in, 1 out]
                n671 = local read "Current Sample Sheet"() -> (w1486:string)
                n672 = call "get sample sheet data cells.vi"("error in (no error)"=w1484, "NI_report in"=w1496) -> ("error out"=w1491:errorcluster, "data"=w1492:string[][], "NI_report out"=w1495:refnum<class "NI_report.lvclass">, "left edge output cluster"=w1489:cluster{"row":i32, "column":i32})  [unwired: 5 in, 1 out]
                n673 = call "find last occupied cell.vi"("data"=w1492, "Active Sheet"=w1486, "Header Rows to remove"=3, "sub array start"=w1489, "error in (no error)"=w1491) -> ("row max value"=w1487:i32, 13:"start of last occupied row"=w1488:cluster{"row":i32, "column":i32}, 14:"start of last occupied row"=w1485:string, "error out"=w1490:errorcluster)  [unwired: 4 in, 3 out]
                n674 = Array Subset(array=w1492, index (col)=2 ("index")) -> ()  [unwired: 3 in, 1 out]
                n675 = local write "row max value"(w1487) -> ()
                n676 = local write "last occupied cell's name"(w1485) -> ()
              }
            }
          }
          frame "ORP Calibration Standard" {
            n677 = invoke on="Record Single Sample" class="Bool" method="Reinit To Default"(error in=w1568) -> (error out=w1567:errorcluster)  [unwired: 2 in, 2 out]
            n678 = call <vilib>:"Clear Errors.vi"("error in (no error)"=w1567) -> ("error out"=w1557:errorcluster)  [unwired: 5 in, 1 out]
            n679 = call "get sample sheet data cells.vi"("error in (no error)"=w1557, "NI_report in"=w1586) -> ("error out"=w1583:errorcluster, "data"=w1585:string[][], "NI_report out"=w1578:refnum<class "NI_report.lvclass">, "left edge output cluster"=w1584:cluster{"row":i32, "column":i32})  [unwired: 5 in, 1 out]
            n680 = flat-sequence {
              tunnel: w1583 -> [w1650]
              tunnel: [w1643] -> _
              tunnel: w1584 -> [w1648]
              tunnel: [w1647] -> w1582
              tunnel: [w1646] -> _
              tunnel: [w1645] -> w1576
              tunnel: w1585 -> [w1643]
              frame #0 {
                n681 = Array Subset(array=w1643, index (col)=2 ("index")) -> ()  [unwired: 3 in, 1 out]
                n682 = local read "Current Sample Sheet"() -> (w1642:string)
                n683 = call "find last occupied cell.vi"("data"=w1643, "Active Sheet"=w1642, "Header Rows to remove"=3, "sub array start"=w1648, "error in (no error)"=w1650) -> ("row max value"=w1646:i32, "column max value"=w1641:i32, 13:"start of last occupied row"=w1645:cluster{"row":i32, "column":i32}, 14:"start of last occupied row"=w1640:string, "error out"=w1647:errorcluster)  [unwired: 4 in, 2 out]
                n684 = local write "last occupied cell's name"(w1640) -> ()
                n685 = local write "row max value"(w1641) -> ()
              }
            }
            n686 = local read "Found Quanta Sonde Com Port"() -> (w1572:refnum<visa-resource-name>)
            n687 = Equal?(x=w1572, y=refnum<visa-resource-name> refnum ("RS232 Port Out")) -> (x = y?=w1574:bool)
            n688 = case shown="False" w1574 {
              tunnel: w1572 -> [w1602 _]
              tunnel: [w1612 w1636] -> w1575
              tunnel: w1582 -> [w1604 w1639]
              tunnel: [w1615 w1639] -> w1579
              tunnel: w1562 -> [w1611 w1638]
              tunnel: [w1610 w1626] -> w1561
              tunnel: [w1609 w1625] -> w1550
              tunnel: w1549 -> [w1608 w1637]
              tunnel: w1560 -> [_ w1622]
              frame False {
                n689 = control-ref of="Sonde Data Display"() -> (w1616:refnum<vi>)
                n690 = call "Calibrate ORP Sensor2.vi"("Calibration Standard"="ORP Reference", "Error In (No Error)"=w1604, "Sensor Address In"="0", "RS232 Port In"=w1602) -> ("Error Out"=w1603:errorcluster, "Sensor Calibrate Response"=→"ORP  Reference\nCalibrate Response":bool, "RS232 Port Out"=w1601:refnum<visa-resource-name>)  [unwired: 3 in, 2 out]
                n691 = local read "Sample Sheet Data Row Cluster 2"() -> (w1613:T3)
                n692 = call "SDI-12 Single Operation with output cluster.vi"("RS232 Port In"=w1601, "Sensor Address In"="0", "Sonde Data Ctl Refnum"=w1616, "Error In (No Error)"=w1603, "Time Array In"=w1611, "Measurement Array In"=w1608) -> ("time array out"=w1610:dbl[], "Measurement  array Out"=w1609:dbl[][], "output cluster"=w1614:T2, "Temperature"=w1618:cluster{"Y":dbl[], "Y":dbl[]}[], "Sonde Data Display"=w1617:T14, "Error Out"=w1615:errorcluster)  [unwired: 12 in, 4 out]
                n693 = Bundle By Name(cluster=w1613, "Sonde Data Cluster"=w1614) -> (w1612:T3)
                n694 = local write "Temperature"(w1618) -> ()
                n695 = local write "Sonde Data Display"(w1617) -> ()
              }
              frame True {
                n696 = Get Date/Time In Seconds() -> (seconds since 1Jan1904=w1628:timestamp)
                n697 = To Double Precision Float(number=w1628) -> (double precision float=w1627:dbl)
                n698 = local read "Sample Sheet Data Row Cluster 2"() -> (w1636:T3)
                n699 = Subtract(x=w1627, y=w1622) -> (x-y=w1620:dbl)
                n700 = local write "Current Time (s)"(w1620) -> ()
                n701 = Unbundle By Name(w1636) -> ("Sonde Data Cluster.Temp\ndeg C"=w1621:dbl, "Sonde Data Cluster.pH"=w1635:dbl, "Sonde Data Cluster.Specific\nCond (mS)"=w1634:dbl, "Sonde Data Cluster.Salinity"=w1633:dbl, "Sonde Data Cluster.Dissolved\nOxygen mg/L"=w1632:dbl, "Sonde Data Cluster.ORP"=w1631:dbl)  [unwired: 1 out]
                n702 = Build Array(w1621, w1635, w1634, w1633, w1632, 0.0 ("element"), w1631) -> (w1629:dbl[])
                n703 = Build Array (concatenate)(w1637, w1629) -> (w1625:dbl[][])
                n704 = Build Array (concatenate)(w1638, w1620) -> (w1626:dbl[])
                n705 = call "format into Sonde Vertical Graph Data Input.vi"("Sonde Measurement Array"=w1625, "Time Array"=w1626) -> ("Sonde Data Display"=w1624:T14, "Temperature"=w1623:cluster{"X":dbl[], "Y":dbl[]}[])  [unwired: 8 in]
                n706 = local write "Temperature"(w1623) -> ()
                n707 = local write "Sonde Data Display"(w1624) -> ()
              }
            }
            n708 = local write "Sample Sheet Data Row Cluster 2"(w1575) -> ()
            n709 = call "write out sonde row.vi"("NI_report in"=w1578, "Columns"=w1581, "Column of Volume"=w1580, "Sample Sheet Data Row Cluster"=w1575, "row index"=w1564, "error in (no error)"=w1579, "start of last occupied row"=w1576) -> ("NI_report out"=w1570:refnum<class "NI_report.lvclass">, "row index out"=w1563:i32, "error out"=w1571:errorcluster)  [unwired: 6 in]
            n710 = flat-sequence {
              tunnel: w1571 -> [w1600]
              tunnel: w1570 -> [w1599]
              tunnel: [w1598] -> w1569
              tunnel: [w1593] -> w1566
              tunnel: [w1591] -> w1565
              frame #0 {
                (unwired) 3 ("Header Rows to remove")
                n711 = call <vilib>:"Clear Errors.vi"("error in (no error)"=w1600) -> ("error out"=w1587:errorcluster)  [unwired: 5 in, 1 out]
                n712 = local read "Current Sample Sheet"() -> (w1589:string)
                n713 = call "get sample sheet data cells.vi"("error in (no error)"=w1587, "NI_report in"=w1599) -> ("error out"=w1594:errorcluster, "data"=w1595:string[][], "NI_report out"=w1598:refnum<class "NI_report.lvclass">, "left edge output cluster"=w1592:cluster{"row":i32, "column":i32})  [unwired: 5 in, 1 out]
                n714 = call "find last occupied cell.vi"("data"=w1595, "Active Sheet"=w1589, "Header Rows to remove"=3, "sub array start"=w1592, "error in (no error)"=w1594) -> ("row max value"=w1590:i32, 13:"start of last occupied row"=w1591:cluster{"row":i32, "column":i32}, 14:"start of last occupied row"=w1588:string, "error out"=w1593:errorcluster)  [unwired: 4 in, 3 out]
                n715 = Array Subset(array=w1595, index (col)=2 ("index")) -> ()  [unwired: 3 in, 1 out]
                n716 = local write "row max value"(w1590) -> ()
                n717 = local write "last occupied cell's name"(w1588) -> ()
              }
            }
          }
          frame "Salinity Calibration Standard" {
            n718 = invoke on="Record Single Sample" class="Bool" method="Reinit To Default"(error in=w1671) -> (error out=w1670:errorcluster)  [unwired: 2 in, 2 out]
            n719 = call <vilib>:"Clear Errors.vi"("error in (no error)"=w1670) -> ("error out"=w1658:errorcluster)  [unwired: 5 in, 1 out]
            n720 = call "get sample sheet data cells.vi"("error in (no error)"=w1658, "NI_report in"=w1689) -> ("error out"=w1686:errorcluster, "data"=w1688:string[][], "NI_report out"=w1681:refnum<class "NI_report.lvclass">, "left edge output cluster"=w1687:cluster{"row":i32, "column":i32})  [unwired: 5 in, 1 out]
            n721 = flat-sequence {
              tunnel: w1686 -> [w1753]
              tunnel: [w1746] -> _
              tunnel: w1687 -> [w1751]
              tunnel: [w1750] -> w1685
              tunnel: [w1749] -> _
              tunnel: [w1748] -> w1679
              tunnel: w1688 -> [w1746]
              frame #0 {
                n722 = Array Subset(array=w1746, index (col)=2 ("index")) -> ()  [unwired: 3 in, 1 out]
                n723 = local read "Current Sample Sheet"() -> (w1745:string)
                n724 = call "find last occupied cell.vi"("data"=w1746, "Active Sheet"=w1745, "Header Rows to remove"=3, "sub array start"=w1751, "error in (no error)"=w1753) -> ("row max value"=w1749:i32, "column max value"=w1744:i32, 13:"start of last occupied row"=w1748:cluster{"row":i32, "column":i32}, 14:"start of last occupied row"=w1743:string, "error out"=w1750:errorcluster)  [unwired: 4 in, 2 out]
                n725 = local write "last occupied cell's name"(w1743) -> ()
                n726 = local write "row max value"(w1744) -> ()
              }
            }
            n727 = local read "Found Quanta Sonde Com Port"() -> (w1675:refnum<visa-resource-name>)
            n728 = Equal?(x=w1675, y=refnum<visa-resource-name> refnum ("RS232 Port Out")) -> (x = y?=w1677:bool)
            n729 = case shown="False" w1677 {
              tunnel: w1675 -> [w1708 _]
              tunnel: [w1715 w1739] -> w1678
              tunnel: w1685 -> [w1706 w1742]
              tunnel: [w1718 w1742] -> w1682
              tunnel: w1665 -> [w1714 w1741]
              tunnel: [w1713 w1729] -> w1664
              tunnel: [w1712 w1728] -> w1663
              tunnel: w1662 -> [w1711 w1740]
              tunnel: w1661 -> [_ w1725]
              frame False {
                n730 = call "Calibrate Salinity Sensor2.vi"("Calibration Standard"="Salinity \nReference", "Error In (No Error)"=w1706, "Sensor Address In"="0", "RS232 Port In"=w1708) -> ("Error Out"=w1705:errorcluster, "Sensor Calibrate Response"=→"Salinity  Reference\nCalibrate Response":bool, "RS232 Port Out"=w1707:refnum<visa-resource-name>)  [unwired: 3 in, 2 out]
                n731 = control-ref of="Sonde Data Display"() -> (w1719:refnum<vi>)
                n732 = local read "Sample Sheet Data Row Cluster 2"() -> (w1716:T3)
                n733 = call "SDI-12 Single Operation with output cluster.vi"("RS232 Port In"=w1707, "Sensor Address In"="0", "Sonde Data Ctl Refnum"=w1719, "Error In (No Error)"=w1705, "Time Array In"=w1714, "Measurement Array In"=w1711) -> ("time array out"=w1713:dbl[], "Measurement  array Out"=w1712:dbl[][], "output cluster"=w1717:T2, "Temperature"=w1721:cluster{"Y":dbl[], "Y":dbl[]}[], "Sonde Data Display"=w1720:T14, "Error Out"=w1718:errorcluster)  [unwired: 12 in, 4 out]
                n734 = local write "Temperature"(w1721) -> ()
                n735 = local write "Sonde Data Display"(w1720) -> ()
                n736 = Bundle By Name(cluster=w1716, "Sonde Data Cluster"=w1717) -> (w1715:T3)
              }
              frame True {
                n737 = Get Date/Time In Seconds() -> (seconds since 1Jan1904=w1731:timestamp)
                n738 = To Double Precision Float(number=w1731) -> (double precision float=w1730:dbl)
                n739 = local read "Sample Sheet Data Row Cluster 2"() -> (w1739:T3)
                n740 = Subtract(x=w1730, y=w1725) -> (x-y=w1723:dbl)
                n741 = local write "Current Time (s)"(w1723) -> ()
                n742 = Unbundle By Name(w1739) -> ("Sonde Data Cluster.Temp\ndeg C"=w1724:dbl, "Sonde Data Cluster.pH"=w1738:dbl, "Sonde Data Cluster.Specific\nCond (mS)"=w1737:dbl, "Sonde Data Cluster.Salinity"=w1736:dbl, "Sonde Data Cluster.Dissolved\nOxygen mg/L"=w1735:dbl, "Sonde Data Cluster.ORP"=w1734:dbl)  [unwired: 1 out]
                n743 = Build Array(w1724, w1738, w1737, w1736, w1735, 0.0 ("element"), w1734) -> (w1732:dbl[])
                n744 = Build Array (concatenate)(w1740, w1732) -> (w1728:dbl[][])
                n745 = Build Array (concatenate)(w1741, w1723) -> (w1729:dbl[])
                n746 = call "format into Sonde Vertical Graph Data Input.vi"("Sonde Measurement Array"=w1728, "Time Array"=w1729) -> ("Sonde Data Display"=w1727:T14, "Temperature"=w1726:cluster{"X":dbl[], "Y":dbl[]}[])  [unwired: 8 in]
                n747 = local write "Temperature"(w1726) -> ()
                n748 = local write "Sonde Data Display"(w1727) -> ()
              }
            }
            n749 = local write "Sample Sheet Data Row Cluster 2"(w1678) -> ()
            n750 = call "write out sonde row.vi"("NI_report in"=w1681, "Columns"=w1684, "Column of Volume"=w1683, "Sample Sheet Data Row Cluster"=w1678, "row index"=w1667, "error in (no error)"=w1682, "start of last occupied row"=w1679) -> ("NI_report out"=w1673:refnum<class "NI_report.lvclass">, "row index out"=w1666:i32, "error out"=w1674:errorcluster)  [unwired: 6 in]
            n751 = flat-sequence {
              tunnel: w1674 -> [w1703]
              tunnel: w1673 -> [w1702]
              tunnel: [w1701] -> w1672
              tunnel: [w1696] -> w1669
              tunnel: [w1694] -> w1668
              frame #0 {
                (unwired) 3 ("Header Rows to remove")
                n752 = call <vilib>:"Clear Errors.vi"("error in (no error)"=w1703) -> ("error out"=w1690:errorcluster)  [unwired: 5 in, 1 out]
                n753 = local read "Current Sample Sheet"() -> (w1692:string)
                n754 = call "get sample sheet data cells.vi"("error in (no error)"=w1690, "NI_report in"=w1702) -> ("error out"=w1697:errorcluster, "data"=w1698:string[][], "NI_report out"=w1701:refnum<class "NI_report.lvclass">, "left edge output cluster"=w1695:cluster{"row":i32, "column":i32})  [unwired: 5 in, 1 out]
                n755 = call "find last occupied cell.vi"("data"=w1698, "Active Sheet"=w1692, "Header Rows to remove"=3, "sub array start"=w1695, "error in (no error)"=w1697) -> ("row max value"=w1693:i32, 13:"start of last occupied row"=w1694:cluster{"row":i32, "column":i32}, 14:"start of last occupied row"=w1691:string, "error out"=w1696:errorcluster)  [unwired: 4 in, 3 out]
                n756 = Array Subset(array=w1698, index (col)=2 ("index")) -> ()  [unwired: 3 in, 1 out]
                n757 = local write "row max value"(w1693) -> ()
                n758 = local write "last occupied cell's name"(w1691) -> ()
              }
            }
          }
          frame "DO Calibration Standard" {
            n759 = invoke on="Record Single Sample" class="Bool" method="Reinit To Default"(error in=w1774) -> (error out=w1773:errorcluster)  [unwired: 2 in, 2 out]
            n760 = call <vilib>:"Clear Errors.vi"("error in (no error)"=w1773) -> ("error out"=w1761:errorcluster)  [unwired: 5 in, 1 out]
            n761 = call "get sample sheet data cells.vi"("error in (no error)"=w1761, "NI_report in"=w1792) -> ("error out"=w1789:errorcluster, "data"=w1791:string[][], "NI_report out"=w1784:refnum<class "NI_report.lvclass">, "left edge output cluster"=w1790:cluster{"row":i32, "column":i32})  [unwired: 5 in, 1 out]
            n762 = flat-sequence {
              tunnel: w1789 -> [w1855]
              tunnel: [w1848] -> _
              tunnel: w1790 -> [w1853]
              tunnel: [w1852] -> w1788
              tunnel: [w1851] -> _
              tunnel: [w1850] -> w1782
              tunnel: w1791 -> [w1848]
              frame #0 {
                n763 = Array Subset(array=w1848, index (col)=2 ("index")) -> ()  [unwired: 3 in, 1 out]
                n764 = local read "Current Sample Sheet"() -> (w1847:string)
                n765 = call "find last occupied cell.vi"("data"=w1848, "Active Sheet"=w1847, "Header Rows to remove"=3, "sub array start"=w1853, "error in (no error)"=w1855) -> ("row max value"=w1851:i32, "column max value"=w1846:i32, 13:"start of last occupied row"=w1850:cluster{"row":i32, "column":i32}, 14:"start of last occupied row"=w1845:string, "error out"=w1852:errorcluster)  [unwired: 4 in, 2 out]
                n766 = local write "last occupied cell's name"(w1845) -> ()
                n767 = local write "row max value"(w1846) -> ()
              }
            }
            n768 = local read "Found Quanta Sonde Com Port"() -> (w1778:refnum<visa-resource-name>)
            n769 = Equal?(x=w1778, y=refnum<visa-resource-name> refnum ("RS232 Port Out")) -> (x = y?=w1780:bool)
            n770 = case shown="False" w1780 {
              tunnel: w1778 -> [w1810 _]
              tunnel: [w1817 w1841] -> w1781
              tunnel: w1788 -> [w1812 w1844]
              tunnel: [w1820 w1844] -> w1785
              tunnel: w1768 -> [w1816 w1843]
              tunnel: [w1815 w1831] -> w1767
              tunnel: [w1814 w1830] -> w1766
              tunnel: w1765 -> [w1813 w1842]
              tunnel: w1764 -> [_ w1827]
              frame False {
                n771 = call "Calibrate DO Sensor.vi"("Calibration Standard"="DO \nReference", "Error In (No Error)"=w1812, "Sensor Address In"="0", "RS232 Port In"=w1810) -> ("Error Out"=w1811:errorcluster, "Sensor Calibrate Response"=→"DO  Reference\nCalibrate Response":bool, "RS232 Port Out"=w1809:refnum<visa-resource-name>)  [unwired: 4 in, 1 out]
                n772 = control-ref of="Sonde Data Display"() -> (w1821:refnum<vi>)
                n773 = call "SDI-12 Single Operation with output cluster.vi"("RS232 Port In"=w1809, "Sensor Address In"="0", "Sonde Data Ctl Refnum"=w1821, "Error In (No Error)"=w1811, "Time Array In"=w1816, "Measurement Array In"=w1813) -> ("time array out"=w1815:dbl[], "Measurement  array Out"=w1814:dbl[][], "output cluster"=w1819:T2, "Temperature"=w1823:cluster{"Y":dbl[], "Y":dbl[]}[], "Sonde Data Display"=w1822:T14, "Error Out"=w1820:errorcluster)  [unwired: 12 in, 4 out]
                n774 = local read "Sample Sheet Data Row Cluster 2"() -> (w1818:T3)
                n775 = local write "Temperature"(w1823) -> ()
                n776 = local write "Sonde Data Display"(w1822) -> ()
                n777 = Bundle By Name(cluster=w1818, "Sonde Data Cluster"=w1819) -> (w1817:T3)
              }
              frame True {
                n778 = Get Date/Time In Seconds() -> (seconds since 1Jan1904=w1833:timestamp)
                n779 = To Double Precision Float(number=w1833) -> (double precision float=w1832:dbl)
                n780 = local read "Sample Sheet Data Row Cluster 2"() -> (w1841:T3)
                n781 = Subtract(x=w1832, y=w1827) -> (x-y=w1825:dbl)
                n782 = local write "Current Time (s)"(w1825) -> ()
                n783 = Unbundle By Name(w1841) -> ("Sonde Data Cluster.Temp\ndeg C"=w1826:dbl, "Sonde Data Cluster.pH"=w1840:dbl, "Sonde Data Cluster.Specific\nCond (mS)"=w1839:dbl, "Sonde Data Cluster.Salinity"=w1838:dbl, "Sonde Data Cluster.Dissolved\nOxygen mg/L"=w1837:dbl, "Sonde Data Cluster.ORP"=w1836:dbl)  [unwired: 1 out]
                n784 = Build Array(w1826, w1840, w1839, w1838, w1837, 0.0 ("element"), w1836) -> (w1834:dbl[])
                n785 = Build Array (concatenate)(w1842, w1834) -> (w1830:dbl[][])
                n786 = Build Array (concatenate)(w1843, w1825) -> (w1831:dbl[])
                n787 = call "format into Sonde Vertical Graph Data Input.vi"("Sonde Measurement Array"=w1830, "Time Array"=w1831) -> ("Sonde Data Display"=w1829:T14, "Temperature"=w1828:cluster{"X":dbl[], "Y":dbl[]}[])  [unwired: 8 in]
                n788 = local write "Temperature"(w1828) -> ()
                n789 = local write "Sonde Data Display"(w1829) -> ()
              }
            }
            n790 = local write "Sample Sheet Data Row Cluster 2"(w1781) -> ()
            n791 = call "write out sonde row.vi"("NI_report in"=w1784, "Columns"=w1787, "Column of Volume"=w1786, "Sample Sheet Data Row Cluster"=w1781, "row index"=w1770, "error in (no error)"=w1785, "start of last occupied row"=w1782) -> ("NI_report out"=w1776:refnum<class "NI_report.lvclass">, "row index out"=w1769:i32, "error out"=w1777:errorcluster)  [unwired: 6 in]
            n792 = flat-sequence {
              tunnel: w1777 -> [w1805]
              tunnel: w1776 -> [w1804]
              tunnel: [w1803] -> w1775
              tunnel: [w1799] -> w1772
              tunnel: [w1797] -> w1771
              frame #0 {
                (unwired) 3 ("Header Rows to remove")
                n793 = call <vilib>:"Clear Errors.vi"("error in (no error)"=w1805) -> ("error out"=w1793:errorcluster)  [unwired: 5 in, 1 out]
                n794 = local read "Current Sample Sheet"() -> (w1795:string)
                n795 = call "get sample sheet data cells.vi"("error in (no error)"=w1793, "NI_report in"=w1804) -> ("error out"=w1800:errorcluster, "data"=w1801:string[][], "NI_report out"=w1803:refnum<class "NI_report.lvclass">, "left edge output cluster"=w1798:cluster{"row":i32, "column":i32})  [unwired: 5 in, 1 out]
                n796 = call "find last occupied cell.vi"("data"=w1801, "Active Sheet"=w1795, "Header Rows to remove"=3, "sub array start"=w1798, "error in (no error)"=w1800) -> ("row max value"=w1796:i32, 13:"start of last occupied row"=w1797:cluster{"row":i32, "column":i32}, 14:"start of last occupied row"=w1794:string, "error out"=w1799:errorcluster)  [unwired: 4 in, 3 out]
                n797 = local write "row max value"(w1796) -> ()
                n798 = local write "last occupied cell's name"(w1794) -> ()
              }
            }
          }
          frame "SC Calibration Standard" {
            n799 = invoke on="Record Single Sample" class="Bool" method="Reinit To Default"(error in=w1876) -> (error out=w1875:errorcluster)  [unwired: 2 in, 2 out]
            n800 = call <vilib>:"Clear Errors.vi"("error in (no error)"=w1875) -> ("error out"=w1863:errorcluster)  [unwired: 5 in, 1 out]
            n801 = call "get sample sheet data cells.vi"("error in (no error)"=w1863, "NI_report in"=w1894) -> ("error out"=w1891:errorcluster, "data"=w1893:string[][], "NI_report out"=w1886:refnum<class "NI_report.lvclass">, "left edge output cluster"=w1892:cluster{"row":i32, "column":i32})  [unwired: 5 in, 1 out]
            n802 = flat-sequence {
              tunnel: w1891 -> [w1957]
              tunnel: [w1951] -> _
              tunnel: w1892 -> [w1955]
              tunnel: [w1954] -> w1890
              tunnel: [w1953] -> _
              tunnel: [w1952] -> w1884
              tunnel: w1893 -> [w1951]
              frame #0 {
                n803 = local read "Current Sample Sheet"() -> (w1950:string)
                n804 = call "find last occupied cell.vi"("data"=w1951, "Active Sheet"=w1950, "Header Rows to remove"=3, "sub array start"=w1955, "error in (no error)"=w1957) -> ("row max value"=w1953:i32, "column max value"=w1949:i32, 13:"start of last occupied row"=w1952:cluster{"row":i32, "column":i32}, 14:"start of last occupied row"=w1948:string, "error out"=w1954:errorcluster)  [unwired: 4 in, 2 out]
                n805 = local write "last occupied cell's name"(w1948) -> ()
                n806 = local write "row max value"(w1949) -> ()
              }
            }
            n807 = local read "Found Quanta Sonde Com Port"() -> (w1880:refnum<visa-resource-name>)
            n808 = Equal?(x=w1880, y=refnum<visa-resource-name> refnum ("RS232 Port Out")) -> (x = y?=w1882:bool)
            n809 = case shown="False" w1882 {
              tunnel: w1880 -> [w1914 _]
              tunnel: [w1920 w1944] -> w1883
              tunnel: w1890 -> [w1912 w1947]
              tunnel: [w1923 w1947] -> w1887
              tunnel: w1870 -> [w1919 w1946]
              tunnel: [w1918 w1934] -> w1869
              tunnel: [w1917 w1933] -> w1868
              tunnel: w1867 -> [w1916 w1945]
              tunnel: w1866 -> [_ w1930]
              frame False {
                n810 = call "Calibrate SC Sensor2.vi"("Calibration Standard"="SC \nReference", "Error In (No Error)"=w1912, "Sensor Address In"="0", "RS232 Port In"=w1914) -> ("Error Out"=w1911:errorcluster, "Sensor Calibrate Response"=→"SC  Reference\nCalibrate Response":bool, "RS232 Port Out"=w1913:refnum<visa-resource-name>)  [unwired: 3 in, 2 out]
                n811 = control-ref of="Sonde Data Display"() -> (w1924:refnum<vi>)
                n812 = local read "Sample Sheet Data Row Cluster 2"() -> (w1921:T3)
                n813 = call <vilib>:"Clear Errors.vi"("error in (no error)"=w1911) -> ("error out"=w1908:errorcluster)  [unwired: 5 in, 1 out]
                n814 = call "SDI-12 Single Operation with output cluster.vi"("RS232 Port In"=w1913, "Sensor Address In"="0", "Sonde Data Ctl Refnum"=w1924, "Error In (No Error)"=w1908, "Time Array In"=w1919, "Measurement Array In"=w1916) -> ("time array out"=w1918:dbl[], "Measurement  array Out"=w1917:dbl[][], "output cluster"=w1922:T2, "Temperature"=w1926:cluster{"Y":dbl[], "Y":dbl[]}[], "Sonde Data Display"=w1925:T14, "Error Out"=w1923:errorcluster)  [unwired: 12 in, 4 out]
                n815 = local write "Temperature"(w1926) -> ()
                n816 = local write "Sonde Data Display"(w1925) -> ()
                n817 = Bundle By Name(cluster=w1921, "Sonde Data Cluster"=w1922) -> (w1920:T3)
              }
              frame True {
                n818 = Get Date/Time In Seconds() -> (seconds since 1Jan1904=w1936:timestamp)
                n819 = To Double Precision Float(number=w1936) -> (double precision float=w1935:dbl)
                n820 = local read "Sample Sheet Data Row Cluster 2"() -> (w1944:T3)
                n821 = Subtract(x=w1935, y=w1930) -> (x-y=w1928:dbl)
                n822 = local write "Current Time (s)"(w1928) -> ()
                n823 = Unbundle By Name(w1944) -> ("Sonde Data Cluster.Temp\ndeg C"=w1929:dbl, "Sonde Data Cluster.pH"=w1943:dbl, "Sonde Data Cluster.Specific\nCond (mS)"=w1942:dbl, "Sonde Data Cluster.Salinity"=w1941:dbl, "Sonde Data Cluster.Dissolved\nOxygen mg/L"=w1940:dbl, "Sonde Data Cluster.ORP"=w1939:dbl)  [unwired: 1 out]
                n824 = Build Array(w1929, w1943, w1942, w1941, w1940, 0.0 ("element"), w1939) -> (w1937:dbl[])
                n825 = Build Array (concatenate)(w1945, w1937) -> (w1933:dbl[][])
                n826 = Build Array (concatenate)(w1946, w1928) -> (w1934:dbl[])
                n827 = call "format into Sonde Vertical Graph Data Input.vi"("Sonde Measurement Array"=w1933, "Time Array"=w1934) -> ("Sonde Data Display"=w1932:T14, "Temperature"=w1931:cluster{"X":dbl[], "Y":dbl[]}[])  [unwired: 8 in]
                n828 = local write "Temperature"(w1931) -> ()
                n829 = local write "Sonde Data Display"(w1932) -> ()
              }
            }
            n830 = local write "Sample Sheet Data Row Cluster 2"(w1883) -> ()
            n831 = call "write out sonde row.vi"("NI_report in"=w1886, "Columns"=w1889, "Column of Volume"=w1888, "Sample Sheet Data Row Cluster"=w1883, "row index"=w1872, "error in (no error)"=w1887, "start of last occupied row"=w1884) -> ("NI_report out"=w1878:refnum<class "NI_report.lvclass">, "row index out"=w1871:i32, "error out"=w1879:errorcluster)  [unwired: 6 in]
            n832 = flat-sequence {
              tunnel: w1879 -> [w1907]
              tunnel: w1878 -> [w1906]
              tunnel: [w1905] -> w1877
              tunnel: [w1901] -> w1874
              tunnel: [w1899] -> w1873
              frame #0 {
                (unwired) 3 ("Header Rows to remove")
                (unwired) 2 ("index")
                n833 = call <vilib>:"Clear Errors.vi"("error in (no error)"=w1907) -> ("error out"=w1895:errorcluster)  [unwired: 5 in, 1 out]
                n834 = local read "Current Sample Sheet"() -> (w1897:string)
                n835 = call "get sample sheet data cells.vi"("error in (no error)"=w1895, "NI_report in"=w1906) -> ("error out"=w1902:errorcluster, "data"=w1903:string[][], "NI_report out"=w1905:refnum<class "NI_report.lvclass">, "left edge output cluster"=w1900:cluster{"row":i32, "column":i32})  [unwired: 5 in, 1 out]
                n836 = call "find last occupied cell.vi"("data"=w1903, "Active Sheet"=w1897, "Header Rows to remove"=3, "sub array start"=w1900, "error in (no error)"=w1902) -> ("row max value"=w1898:i32, 13:"start of last occupied row"=w1899:cluster{"row":i32, "column":i32}, 14:"start of last occupied row"=w1896:string, "error out"=w1901:errorcluster)  [unwired: 4 in, 3 out]
                n837 = local write "row max value"(w1898) -> ()
                n838 = local write "last occupied cell's name"(w1896) -> ()
              }
            }
          }
          frame "Write Sonde Sample Sheet" {
            n839 = flat-sequence {
              tunnel: w1984 -> [w2001]
              tunnel: w1983 -> [w2000]
              tunnel: w1981 -> [w1997]
              tunnel: w1980 -> [w1996]
              tunnel: w1979 -> [w1995]
              tunnel: [w1994] -> w1978
              tunnel: w1977 -> [w1993]
              tunnel: w1976 -> [w1992]
              tunnel: w1975 -> [w1990]
              tunnel: [w1988] -> w1973
              tunnel: [w1987] -> w1972
              tunnel: [w1986] -> w1971
              tunnel: w1960 -> [w1985]
              frame #0 {
                n840 = Not Equal?(x=w1993, y=w1992) -> (x != y?=w1991:bool)
                n841 = invoke on="Update Sonde" class="Bool (strict)" method="Reinit To Default"() -> ()  [unwired: 3 in, 3 out]
                n842 = Decrement(x=w1985) -> (x-1=w1986:i32)
                n843 = case shown="True" w1991 {
                  tunnel: w2001 -> [w2004 w2011]
                  tunnel: w1990 -> [_ w2010]
                  tunnel: w2000 -> [w2003 w2009]
                  tunnel: [w2003 w2008] -> w1999
                  tunnel: [w2004 w2007] -> w1998
                  tunnel: w1995 -> [w2002 w2006]
                  tunnel: [w2002 w2005] -> w1994
                  frame False {
                  }
                  frame True {
                    n844 = flat-sequence {
                      tunnel: [w2020] -> w2007
                      tunnel: w2011 -> [w2019]
                      tunnel: w2010 -> [w2016]
                      tunnel: w2009 -> [w2015]
                      tunnel: [w2014] -> w2008
                      tunnel: w2006 -> [w2013]
                      tunnel: [w2012] -> w2005
                      frame #0 {
                        n845 = Increment(x=w2013) -> (x+1=w2012:i32)
                        n846 = call "write comment cell with column offset.vi"("Column Relative?"=TRUE, "comment string"="done", "error in (no error)"=w2015, "start of last occupied row"=w2016, "NI_report in"=w2019) -> ("error out"=w2014:errorcluster, "NI_report out"=w2020:refnum<class "NI_report.lvclass">)  [unwired: 5 in]
                      }
                    }
                  }
                }
                n847 = call "open select sample sheet.vi"("Number of Sample Sheets"=w1996, "error in (no error)"=w1999, "Worksheet Names"=w1997, "input 1"=w1994, "NI_report in"=w1998) -> ("error out"=w1988:errorcluster, "Current Sample Sheet"=w1989:string, "NI_report out"=w1987:refnum<class "NI_report.lvclass">)  [unwired: 4 in]
                n848 = local write "Current Sample Sheet"(w1989) -> ()
              }
            }
            n849 = flat-sequence {
              tunnel: w1960 -> [w2035]
              frame #0 {
                n850 = local read "Sonde Data Array"() -> (w2038:T12[])
                n851 = Index Array(array=w2038, index=w2035) -> (element=w2040:T12)
                n852 = Bundle By Name(cluster=w2040, "Final"=TRUE) -> (w2036:T12)
                n853 = Replace Array Subset(array=w2038, new element=w2036, index=w2035) -> (w2037:T12[])
                n854 = local write "Sonde Data Array"(w2037) -> ()
              }
            }
            n855 = flat-sequence {
              tunnel: [w2033] -> w1982
              tunnel: [w2032] -> w1974
              tunnel: w1973 -> [w2031]
              tunnel: w1972 -> [w2030]
              tunnel: [w2022] -> w1966
              frame #0 {
                n856 = local read "Current Sample Sheet"() -> (w2024:string)
                n857 = call "get sample sheet data cells.vi"("error in (no error)"=w2031, "NI_report in"=w2030) -> ("error out"=w2034:errorcluster, "data"=w2028:string[][], "NI_report out"=w2033:refnum<class "NI_report.lvclass">, "left edge output cluster"=w2026:cluster{"row":i32, "column":i32})  [unwired: 5 in, 1 out]
                n858 = Array Subset(array=w2028, index (col)=2 ("index")) -> ()  [unwired: 3 in, 1 out]
                n859 = call "find last occupied cell.vi"("Active Sheet"=w2024, "Header Rows to remove"=3, "sub array start"=w2026, "error in (no error)"=w2034) -> ("row max value"=w2025:i32, 13:"start of last occupied row"=w2032:cluster{"row":i32, "column":i32}, 14:"start of last occupied row"=w2023:string, "error out"=w2022:errorcluster)  [unwired: 5 in, 3 out]
                n860 = local write "row max value"(w2025) -> ()
                n861 = local write "last occupied cell's name"(w2023) -> ()
                n862 = local write "Sonde Data Array"(T12[] [{"Head"=0.0, "Depth"=0.0, "Time"="19:00", "Cumulative\nVolume"=0.0, "Sp. Conductance"={"Value"=0.506, "%"=0.0, "Tol."=TRUE}, "Dissolved Oxygen"={"Value"=35.14, "%"=0.0, "Tol."=TRUE}, "pH"={"Value"=4.81, "%"=0.0, "Tol."=TRUE}, "ORP"={"Value"=390.0, "%"=0.0, "Tol."=TRUE}, "Temperature"={"Value"=23.86, "%"=0.0, "Tol."=TRUE}, "Salinity"={"Value"=0.24, "%"=0.0, "Tol."=TRUE}, "Final Tol."=TRUE, "Final"=FALSE, "Time 2"=timestamp(0 s since 1904-01-01), "Aux 1"=0.0, "Aux 2"=0.0, "Aux 3"=0.0}, {"Head"=0.0, "Depth"=0.0, "Time"="19:00", "Cumulative\nVolume"=0.0, "Sp. Conductance"={"Value"=0.506, "%"=0.0, "Tol."=TRUE}, "Dissolved Oxygen"={"Value"=35.12, "%"=0.0, "Tol."=TRUE}, "pH"={"Value"=4.81, "%"=0.0, "Tol."=TRUE}, "ORP"={"Value"=390.0, "%"=0.0, "Tol."=TRUE}, "Temperature"={"Value"=23.89, "%"=0.0, "Tol."=TRUE}, "Salinity"={"Value"=0.24, "%"=0.0, "Tol."=TRUE}, "Final Tol."=TRUE, "Final"=FALSE, "Time 2"=timestamp(0 s since 1904-01-01), "Aux 1"=0.0, "Aux 2"=0.0, "Aux 3"=0.0}, {"Head"=0.0, "Depth"=0.0, "Time"="19:00", "Cumulative\nVolume"=0.0, "Sp. Conductance"={"Value"=0.506, "%"=0.0, "Tol."=TRUE}, "Dissolved Oxygen"={"Value"=35.14, "%"=0.0, "Tol."=TRUE}, "pH"={"Value"=4.81, "%"=0.0, "Tol."=TRUE}, "ORP"={"Value"=390.0, "%"=0.0, "Tol."=TRUE}, "Temperature"={"Value"=23.86, "%"=0.0, "Tol."=TRUE}, "Salinity"={"Value"=0.24, "%"=0.0, "Tol."=TRUE}, "Final Tol."=TRUE, "Final"=FALSE, "Time 2"=timestamp(0 s since 1904-01-01), "Aux 1"=0.0, "Aux 2"=0.0, "Aux 3"=0.0}, {"Head"=0.0, "Depth"=0.0, "Time"="", "Cumulative\nVolume"=0.0, "Sp. Conductance"={"Value"=0.0, "%"=0.0, "Tol."=FALSE}, "Dissolved Oxygen"={"Value"=0.0, "%"=0.0, "Tol."=FALSE}, "pH"={"Value"=0.0, "%"=0.0, "Tol."=FALSE}, "ORP"={"Value"=0.0, "%"=0.0, "Tol."=FALSE}, "Temperature"={"Value"=0.0, "%"=0.0, "Tol."=FALSE}, "Salinity"={"Value"=0.0, "%"=0.0, "Tol."=FALSE}, "Final Tol."=FALSE, "Final"=FALSE, "Time 2"=timestamp(0 s since 1904-01-01), "Aux 1"=0.0, "Aux 2"=0.0, "Aux 3"=0.0}, {"Head"=0.0, "Depth"=0.0, "Time"="", "Cumulative\nVolume"=0.0, "Sp. Conductance"={"Value"=0.0, "%"=0.0, "Tol."=FALSE}, "Dissolved Oxygen"={"Value"=0.0, "%"=0.0, "Tol."=FALSE}, "pH"={"Value"=0.0, "%"=0.0, "Tol."=FALSE}, "ORP"={"Value"=0.0, "%"=0.0, "Tol."=FALSE}, "Temperature"={"Value"=0.0, "%"=0.0, "Tol."=FALSE}, "Salinity"={"Value"=0.0, "%"=0.0, "Tol."=FALSE}, "Final Tol."=FALSE, "Final"=FALSE, "Time 2"=timestamp(0 s since 1904-01-01), "Aux 1"=0.0, "Aux 2"=0.0, "Aux 3"=0.0}, {"Head"=0.0, "Depth"=0.0, "Time"="", "Cumulative\nVolume"=0.0, "Sp. Conductance"={"Value"=0.0, "%"=0.0, "Tol."=FALSE}, "Dissolved Oxygen"={"Value"=0.0, "%"=0.0, "Tol."=FALSE}, "pH"={"Value"=0.0, "%"=0.0, "Tol."=FALSE}, "ORP"={"Value"=0.0, "%"=0.0, "Tol."=FALSE}, "Temperature"={"Value"=0.0, "%"=0.0, "Tol."=FALSE}, "Salinity"={"Value"=0.0, "%"=0.0, "Tol."=FALSE}, "Final Tol."=FALSE, "Final"=FALSE, "Time 2"=timestamp(0 s since 1904-01-01), "Aux 1"=0.0, "Aux 2"=0.0, "Aux 3"=0.0}, {"Head"=0.0, "Depth"=0.0, "Time"="", "Cumulative\nVolume"=0.0, "Sp. Conductance"={"Value"=0.0, "%"=0.0, "Tol."=FALSE}, "Dissolved Oxygen"={"Value"=0.0, "%"=0.0, "Tol."=FALSE}, "pH"={"Value"=0.0, "%"=0.0, "Tol."=FALSE}, "ORP"={"Value"=0.0, "%"=0.0, "Tol."=FALSE}, "Temperature"={"Value"=0.0, "%"=0.0, "Tol."=FALSE}, "Salinity"={"Value"=0.0, "%"=0.0, "Tol."=FALSE}, "Final Tol."=FALSE, "Final"=FALSE, "Time 2"=timestamp(0 s since 1904-01-01), "Aux 1"=0.0, "Aux 2"=0.0, "Aux 3"=0.0}, {"Head"=0.0, "Depth"=0.0, "Time"="", "Cumulative\nVolume"=0.0, "Sp. Conductance"={"Value"=0.0, "%"=0.0, "Tol."=FALSE}, "Dissolved Oxygen"={"Value"=0.0, "%"=0.0, "Tol."=FALSE}, "pH"={"Value"=0.0, "%"=0.0, "Tol."=FALSE}, "ORP"={"Value"=0.0, "%"=0.0, "Tol."=FALSE}, "Temperature"={"Value"=0.0, "%"=0.0, "Tol."=FALSE}, "Salinity"={"Value"=0.0, "%"=0.0, "Tol."=FALSE}, "Final Tol."=FALSE, "Final"=FALSE, "Time 2"=timestamp(0 s since 1904-01-01), "Aux 1"=0.0, "Aux 2"=0.0, "Aux 3"=0.0}, {"Head"=0.0, "Depth"=0.0, "Time"="", "Cumulative\nVolume"=0.0, "Sp. Conductance"={"Value"=0.0, "%"=0.0, "Tol."=FALSE}, "Dissolved Oxygen"={"Value"=0.0, "%"=0.0, "Tol."=FALSE}, "pH"={"Value"=0.0, "%"=0.0, "Tol."=FALSE}, "ORP"={"Value"=0.0, "%"=0.0, "Tol."=FALSE}, "Temperature"={"Value"=0.0, "%"=0.0, "Tol."=FALSE}, "Salinity"={"Value"=0.0, "%"=0.0, "Tol."=FALSE}, "Final Tol."=FALSE, "Final"=FALSE, "Time 2"=timestamp(0 s since 1904-01-01), "Aux 1"=0.0, "Aux 2"=0.0, "Aux 3"=0.0}] ("Sonde Data Array")) -> ()
              }
            }
          }
          frame "Init" {
            n863 = flat-sequence {
              tunnel: w2064 -> [w2377]
              tunnel: [w2364] -> w2054
              tunnel: [w2363] -> w2053
              frame #0 {
                n864 = call "create DAQ strings.vi"("error in (no error)"=w2377, "MCC USB-DAQ Setup"="MCC USB-DAQ Setup") -> ("error IO"=w2370:errorcluster, "Descriptions"=w2368:string[], "delimited string"=w2371:string, "Array"=w2369:string[], "Voltage Range"=w2376:dbl[])  [unwired: 5 in]
                "delimited string" <- w2371
                "Active Channel Array" <- w2369
                "Voltage Range" <- w2376
                "Descriptions" <- w2368
                n865 = call "Physical Channels to Number of channels.vi"("error in (no error)"=w2370, "Physical Channel in"=w2371) -> ("error out"=w2372:errorcluster, "Number of Channels"=w2374:i32)  [unwired: 7 in, 1 out]
                "Number \nof Channels" <- w2374
                n866 = call "Calculate Rate from Num Channels and Max Rate.vi"("error in (no error)"=w2372, "Channel Data Rate S/s"="Channel \nData Rate S/s", "Number of Channels"=w2374) -> ("error out"=w2367:errorcluster, "Rate"=→"Rate":dbl)  [unwired: 7 in]
                n867 = for {
                  tunnel: w2369 -> [w2390] mode=indexing
                  tunnel: w2376 -> [w2389] mode=indexing
                  tunnel: [w2386] -> w2366 mode=indexing
                  shift-right: [w2387] -> w2365
                  shift-left: w2367 -> [w2385]
                  n868 = Negate(x=w2389) -> (-x=w2388:dbl)
                  n869 = call-poly <vilib>:"ULx Create Virtual Channel.vi"("maximum value"=w2389, "minimum value"=w2388, "physical channels"=w2390, "error in"=w2385) -> ("task out"=w2386:refnum<k24>, "error out"=w2387:errorcluster)  [unwired: 10 in]
                }
                n870 = call "get 9V monitor voltage.vi"("error in (no error)"=w2365, "Descriptions"=w2368, "Array"=w2369, "Array 2"=w2366) -> ("error out"=w2364:errorcluster, "9V Voltage Monitor"=w2362:dbl)  [unwired: 6 in]
                "DAQ Error" <- w2364
                "9V Voltage Monitor" <- w2362
                n871 = Greater Or Equal?(x=w2362, y=8.75) -> ()  [unwired: 1 out]
                n872 = flat-sequence {
                  tunnel: [w2383] -> w2363
                  tunnel: w2366 -> [w2381]
                  tunnel: w2364 -> [w2380]
                  frame #0 {
                    n873 = local read "Descriptions"() -> (w2384:string[])
                    n874 = call "Measure DAQ Voltages.vi"("error in (no error)"=w2380, "Descriptions"=w2384, "Array in"=w2381) -> ("Raw Voltages"=w2382:dbl[], "Array out"=w2383:refnum<k24>[], "Sensor Cluster"=w2379:T10)  [unwired: 6 in]
                    n875 = local write "Sensor Voltage Cluster"(w2379) -> ()
                    n876 = local write "Raw Voltages"(w2382) -> ()
                  }
                }
              }
            }
            n877 = local write "Initialization"(-1 ("Initialization")) -> ()
            n878 = flat-sequence {
              tunnel: w2054 -> [w2354]
              tunnel: [w2354] -> w2062
              frame #0 {
                w2355 = T22."Enabled" ("Disabled")
                n879 = property on="Write Data to Spreadsheet" class="Bool"("DisabledEnum"=w2355) -> (error out=w2358:errorcluster)  [unwired: 2 in, 1 out]
                n880 = property on="Record Continuous Samples" class="Bool"(error in=w2358, "DisabledEnum"=T22."Disabled and Grayed Out" ("Disabled")) -> (error out=w2357:errorcluster)  [unwired: 1 in, 1 out]
                n881 = property on="Record Single Sample" class="Bool"(error in=w2357, "DisabledEnum"=w2355) -> (error out=w2356:errorcluster)  [unwired: 1 in, 1 out]
                n882 = property on="Sample Not Collected" class="Bool"(error in=w2356, "DisabledEnum"=w2355) -> (error out=w2353:errorcluster)  [unwired: 1 in, 1 out]
                n883 = invoke on="Sonde Data Array" class="Arr (strict)" method="Reinit To Default"(error in=w2353) -> ()  [unwired: 2 in, 3 out]
                "Initialization Finished" <- TRUE
                "Zero Pressure\nIndicator" <- FALSE ("Zero Pressure\nIndicator")
              }
            }
            n884 = call <vilib>:"Clear Errors.vi"("error in (no error)"=w2054) -> ("error out"=w2041:errorcluster)  [unwired: 5 in, 1 out]
            n885 = local read "Descriptions"() -> (w2042:string[])
            n886 = stacked-sequence {
              seq-local: [w2080 _ _ _ _ _ _ _ _ _] -> [_ w2109 _ _ _ _ _ _ _ _]
              seq-local: [_ w2110 _ _ _ _ _ _ _ _] -> [_ _ w2131 _ _ _ _ _ _ _]
              seq-local: [_ _ w2130 _ _ _ _ _ _ _] -> [_ _ _ _ _ _ _ _ _ w2301]
              tunnel: [_ _ w2135 _ _ _ _ _ _ _] -> _
              tunnel: w2056 -> [_ _ _ _ _ _ _ _ _ w2304]
              tunnel: [_ _ _ _ _ _ _ _ _ w2303] -> w2055
              tunnel: w2041 -> [w2082 _ _ _ _ _ _ _ _ _]
              tunnel: w2053 -> [_ _ w2133 w2206 w2235 _ _ _ w2272 _]
              tunnel: w2042 -> [_ _ w2132 w2207 w2234 _ _ _ w2271 _]
              tunnel: [_ _ _ w2208 _ _ _ _ _ _] -> _
              tunnel: [_ _ _ _ _ _ _ _ _ w2301] -> w2057
              tunnel: w2045 -> [_ _ w2129 _ _ _ _ _ _ _]
              tunnel: [_ _ w2128 _ _ _ _ _ _ _] -> w2044
              frame #0 {
                n887 = flat-sequence {
                  tunnel: [w2087] -> w2080
                  tunnel: w2082 -> [w2088]
                  frame #0 {
                    n888 = local read "Groundwater Header"() -> (w2094:T11)
                    n889 = Unbundle By Name(w2094) -> ("Kpro box Serial"=w2084:string)
                    n890 = Scan From String(format string="%d", input string=w2084, error in=w2088, default 1=800.0 ("default value 1")) -> (error out=w2089:errorcluster, output 1=w2093:dbl)  [unwired: 1 in, 2 out]
                    n891 = Equal?(x=w2084, y="") -> (x = y?=w2085:bool)
                    n892 = case shown="True" w2085 {
                      tunnel: "KPRO Box Number\n\nEnter the number of the KPRO box you are using." ("prompt") -> [_ w2108]
                      tunnel: w2094 -> [w2098 w2107]
                      tunnel: w2093 -> [w2096 w2106]
                      tunnel: [w2096 w2105] -> w2092
                      tunnel: [w2098 w2103] -> w2090
                      tunnel: w2089 -> [w2097 w2101]
                      tunnel: [w2097 w2100] -> w2087
                      frame False {
                      }
                      frame True {
                        n893 = call "prompt_and_enter_value2.vi"("prompt_IN"=w2108, "Enter value"=w2106) -> ("Numeric"=w2105:dbl)  [unwired: 9 in]
                        n894 = call <vilib>:"Clear Errors.vi"("error in (no error)"=w2101) -> ("error out"=w2099:errorcluster)  [unwired: 5 in, 1 out]
                        n895 = Format Into String(format string="%d", error in=w2099, w2105) -> (resulting string=w2102:string, error out=w2100:errorcluster)  [unwired: 1 in]
                        n896 = Bundle By Name(cluster=w2107, "Kpro box Serial"=w2102) -> (w2103:T11)
                      }
                    }
                    n897 = global write "Kpro Globals.vi" "KPRO Box Number"(w2092) -> ()
                    n898 = local write "Groundwater Header"(w2090) -> ()
                  }
                }
                "Initialization" <- 0
              }
              frame #1 {
                n899 = local write "Initialization"(1 ("Initialization")) -> ()
                n900 = flat-sequence {
                  tunnel: w2109 -> [w2113]
                  tunnel: [w2112] -> w2110
                  frame #0 {
                    n901 = local read "Groundwater Header"() -> (w2121:T11)
                    n902 = local read "Temporary Data Files Directory"() -> (w2117:path)
                    n903 = Unbundle By Name(w2121) -> ("Profile ID"=w2120:string)
                    n904 = Equal?(x=w2120, y="") -> ()  [unwired: 1 out]
                    n905 = case shown="True" TRUE {
                      tunnel: "Profile ID\n\nEnter the profile ID" ("prompt") -> [_ w2127]
                      tunnel: [w2124 w2126] -> w2116
                      tunnel: w2120 -> [w2124 w2125]
                      frame False {
                      }
                      frame True {
                        n906 = call "prompt_string.vi"("prompt_IN"=w2127, "Enter value"=w2125) -> ("String"=w2126:string)  [unwired: 9 in]
                        n907 = global write "Kpro Globals.vi" "Profile ID"(w2126) -> ()
                      }
                    }
                    n908 = Bundle By Name(cluster=w2121, "Profile ID"=w2116) -> (w2122:T11)
                    n909 = call-poly <userlib>:"Build Path__ogtk.vi"("name or relative path"=w2116, "base path"=w2117) -> ("appended path"=w2115:path)
                    n910 = local write "Groundwater Header"(w2122) -> ()
                    n911 = call <userlib>:"Create Dir if Non-Existant__ogtk.vi"("error in (no error)"=w2113, "Directory Path"=w2115) -> ("error out"=w2112:errorcluster, "dup Directory Path"=w2114:path)  [unwired: 7 in, 1 out]
                    n912 = local write "Output File Path"(w2114) -> ()
                  }
                }
              }
              frame #2 {
                n913 = flat-sequence {
                  tunnel: [w2158] -> w2135
                  tunnel: w2131 -> [w2165]
                  tunnel: w2133 -> [w2163]
                  tunnel: w2132 -> [w2162]
                  tunnel: [w2150] -> w2130
                  tunnel: w2129 -> [w2149]
                  tunnel: [w2148] -> w2128
                  frame #0 {
                    n914 = local read "Input Variables and Slopes"() -> (w2169:T1)
                    n915 = call <vilib>:"Clear Errors.vi"("error in (no error)"=w2165) -> ("error out"=w2151:errorcluster)  [unwired: 5 in, 1 out]
                    n916 = local read "Temporary Data Files Directory"() -> (w2164:path)
                    n917 = Unbundle By Name(w2169) -> ("Up Hole Pressure Slope"=w2172:dbl, "String Pot Slope"=w2171:dbl, "Flow Slope"=w2170:dbl)
                    n918 = call "FILE_DIALOG 2016.vi"("flow_slope_IN"=w2170, "pressure_slope_IN"=w2172, "string_pot_slope_IN"=w2171, "Descriptions"=w2162, "error in (no error)"=w2151, "start path"=w2164, "Array in"=w2163) -> ("path"=w2145:path, "exists"=w2161:bool, "flow_slope_OUT"=w2167:dbl, "pressure_slope_OUT"=w2166:dbl, "Record Output Slopes to  Record File"=w2146:path, "string_pot_slope_OUT"=w2168:dbl, "Record Output Slopes for slopes.csv File"=w2147:path, "error out"=w2157:errorcluster)  [unwired: 11 in, 2 out]
                    "Output File Path" <- w2145
                    n919 = local write "Slopes History File Path"(w2146) -> ()
                    n920 = global write "Kpro Globals.vi" "Flow Slope"(w2167) -> ()
                    n921 = Bundle By Name(cluster=w2169, "String Pot Slope"=w2168, "Flow Slope"=w2167, "Up Hole Pressure Slope"=w2166) -> (w2159:T1)
                    n922 = global write "Kpro Globals.vi" "Pressure \nSlope"(w2166) -> ()
                    n923 = global write "Kpro Globals.vi" "String Pot \nSlope"(w2168) -> ()
                    n924 = local write "Slopes File Path"(w2147) -> ()
                    n925 = Path To String(path=w2145) -> (string=w2141:string)
                    n926 = call-poly <userlib>:"Strip Path__ogtk.vi"("path"=w2145) -> ("name"=w2140:string)  [unwired: 1 out]
                    n927 = String Length(string=w2140) -> (length=w2155:i32)
                    n928 = Concatenate Strings(w2141, w2140) -> (w2138:string)
                    n929 = String To Path(string=w2138) -> (path=→"appended path":path)
                    n930 = Equal To 0?(x=w2155) -> (x = 0?=w2137:bool)
                    n931 = local write "Input Variables and Slopes"(w2159) -> ()
                    n932 = Or(x=w2137, y=w2137) -> ()  [unwired: 1 out]
                    n933 = Concatenate Strings(w2138, "_KPROsession.csv") -> (w2144:string)
                    n934 = Concatenate Strings(w2138, "Static Ik.csv" ("string")) -> (w2142:string)
                    n935 = String To Path(string=w2144) -> (path=w2160:path)
                    "KPRO SessionOutput File Path" <- w2160
                    n936 = String To Path(string=w2142) -> (path=w2136:path)
                    n937 = local write "Static IK path"(w2136) -> ()
                    n938 = call <vilib>:"Check if File or Folder Exists.vi"("path"=w2160) -> ("file or folder exists?"=w2152:bool, "dup path"=w2154:path)  [unwired: 8 in, 1 out]
                    n939 = And(x=w2152, y=w2161) -> (x .and. y?=w2153:bool)
                    n940 = case shown="True" w2153 {
                      selector: w2153 -> [_ w2179]
                      tunnel: w2154 -> [_ w2190]
                      tunnel: w2159 -> [w2175 w2185]
                      tunnel: [w2175 w2184] -> w2158
                      tunnel: w2157 -> [w2174 w2180]
                      tunnel: [w2174 w2180] -> w2150
                      tunnel: w2149 -> [w2173 w2178]
                      tunnel: [w2173 w2177] -> w2148
                      frame False {
                      }
                      frame True {
                        n941 = local read "Culmulative Graph Cluster"() -> (w2189:T19)
                        n942 = call "Get_KPRO_data_from_file 2016.vi"("Output File KPRO Test"=w2190) -> ("Last_height_of_box"=w2182:dbl, "Last_depth_to_water"=w2183:dbl, "Last_depth"=w2181:dbl, "Output_array"=w2176:sgl[][])  [unwired: 7 in]
                        "Cumulative_data_from_file" <- w2176
                        n943 = Bundle By Name(cluster=w2185, "Depth to Water Table"=w2183, "Height of Sample Box"=w2182) -> (w2184:T1)
                        n944 = Bundle By Name(cluster=w2178, "Absolute Depth In"=w2181, "Current Absolute Depth"=w2181) -> (w2177:T17)
                        n945 = call "Array to Plot 2016.vi"("Input Cumulative Array"=w2176) -> ("Cumulative - Depth vs.Drive Rate"=w2186:cluster{dbl[], dbl[]}, "Cumulative - Depth vs. Ik"=w2187:cluster{dbl[], dbl[]})  [unwired: 3 in, 4 out]
                        n946 = Bundle By Name(cluster=w2189, "Cumulative - Depth vs. Ik"=w2187, "Cumulative - Depth vs. Drive Rate"=w2186) -> (w2188:T19)
                        n947 = local write "Culmulative Graph Cluster"(w2188) -> ()
                        n948 = local write "Input Variables and Slopes"(w2184) -> ()
                        "Cumulative_data_ready" <- w2179
                      }
                    }
                  }
                }
                n949 = local write "Initialization"(2 ("Initialization")) -> ()
              }
              frame #3 {
                # "Take offset and put\n into Pressure VI."
                n950 = local write "Initialization"(3 ("Initialization")) -> ()
                n951 = local read "Groundwater Header"() -> (w2198:T11)
                n952 = global read "Kpro Globals.vi" "Pressure Offset"() -> (w2191:dbl)
                n953 = local read "Input Variables and Slopes"() -> (w2196:T1)
                n954 = Unbundle By Name(w2198) -> ("Atmospheric Pressure"=w2195:string)
                n955 = case shown="False" TRUE {
                  tunnel: "ATMOSPHERIC PRESSURE READING\n\nHold Kpro effluent facing up and level with the pressure transducer.\nTurn on Kpro water, turn off when water flows with no air bubbles.\n\nPress OK when the reading equilibrates." ("message") -> [_ w2232]
                  tunnel: [w2223 w2231] -> w2213
                  tunnel: [w2222 w2225] -> w2210
                  tunnel: w2207 -> [_ w2230]
                  tunnel: w2206 -> [w2220 w2229]
                  tunnel: [w2221 w2228] -> w2205
                  tunnel: [w2217 w2227] -> w2200
                  tunnel: [w2220 w2226] -> w2199
                  tunnel: w2196 -> [w2222 w2225]
                  tunnel: w2195 -> [w2218 _]
                  tunnel: [w2216 w2224] -> w2192
                  tunnel: w2191 -> [w2216 w2224]
                  frame False {
                    n956 = local read "Sensor Voltage Cluster"() -> (w2223:T10)
                    n957 = Unbundle By Name(w2222) -> ("Up Hole Pressure Slope"=w2221:dbl)
                    n958 = Scan From String(input string=w2218, default 1=35.0 ("default value 1")) -> (output 1=w2217:dbl)  [unwired: 3 in, 3 out]
                  }
                  frame True {
                    n959 = local read "Sensor Voltage Cluster"() -> (w2231:T10)
                    n960 = Unbundle By Name(w2225) -> ("Up Hole Pressure Slope"=w2228:dbl)
                    n961 = call "Up Hole PRESSURE_CAL 2016.vi"("Pressure Offset"=w2224, "Descriptions"=w2230, "Array in"=w2229, "Pressure \nSlope"=w2228, "Sensor Cluster"=w2231, "Prompt_IN"=w2232) -> ("PRESSURE\nFt of water"=w2227:dbl, "Array out"=w2226:refnum<k24>[])  [unwired: 4 in]
                    "Pressure Offset" <- w2224
                  }
                }
                n962 = Equal?(x=w2195, y="") -> ()  [unwired: 1 out]
                n963 = local read "Corrected Pressure Cluster"() -> (w2212:T20)
                n964 = Bundle By Name(cluster=w2210, "Atmospheric Pressure"=w2200, "Up Hole  Pressure Offset"=w2192) -> (w2209:T1)
                n965 = global write "Kpro Globals.vi" "Atmospheric Pressure"(w2200) -> ()
                n966 = Format Into String(w2200) -> (resulting string=w2201:string)  [unwired: 3 in, 1 out]
                n967 = call "up hole Pressure 2016.vi"("Sensor Cluster"=w2213, "Pressure Offset"=w2200, "Array in"=w2199, "Pressure \nSlope"=w2205, "Descriptions"=w2207, "Zero Pressure\n(F = leave as is)"=TRUE) -> ("Array out"=w2208:refnum<k24>[], "Uphole Pressure"=w2193:dbl, "Sensor Cluster 2"=w2203:T10)  [unwired: 6 in, 1 out]
                n968 = Bundle By Name(cluster=w2198, "Atmospheric Pressure"=w2201) -> (w2202:T11)
                n969 = Bundle By Name(cluster=w2212, "Up hole Corrected Pressure"=w2193) -> (w2211:T20)
                n970 = local write "Sensor Voltage Cluster"(w2203) -> ()
                n971 = local write "Input Variables and Slopes"(w2209) -> ()
                n972 = local write "Groundwater Header"(w2202) -> ()
                n973 = local write "Corrected Pressure Cluster"(w2211) -> ()
                n974 = local write "Uphole Pressure"(w2193) -> ()
              }
              frame #4 {
                n975 = flat-sequence {
                  tunnel: w2235 -> [w2244]
                  tunnel: w2234 -> [w2243]
                  frame #0 {
                    n976 = local read "Input Variables and Slopes"() -> (w2242:T1)
                    n977 = Unbundle By Name(w2242) -> ("Up Hole Pressure Slope"=w2241:dbl)
                    n978 = local read "Sensor Voltage Cluster"() -> (w2247:T10)
                    n979 = global read "Kpro Globals.vi" "Pressure Offset"() -> (w2240:dbl)
                    n980 = call "Up Hole PRESSURE_CAL 2016.vi"("Pressure Offset"=w2240, "Descriptions"=w2243, "Array in"=w2244, "Pressure \nSlope"=w2241, "Sensor Cluster"=w2247, "Prompt_IN"="CHECK RESERVOIR PRESSURE\n\nTurn on Kpro. Unplug Kpro Out quick connect from sample box.\nReservoir pressure should be 69.2 +/- 5%(65.7 - 72.7).\n\nPress OK when the reading equilibrates within range." ("message")) -> ("PRESSURE\nFt of water"=w2237:dbl)  [unwired: 4 in, 1 out]
                    n981 = local read "Groundwater Header"() -> (w2239:T11)
                    n982 = Format Into String(w2237) -> (resulting string=w2236:string)  [unwired: 3 in, 1 out]
                    n983 = global write "Kpro Globals.vi" "Reservoir Pressure"(w2237) -> ()
                    n984 = Bundle By Name(cluster=w2242, "Reservoir Pressure"=w2237) -> (w2245:T1)
                    n985 = Bundle By Name(cluster=w2239, "KPRO N2 Pressure"=w2236) -> (w2238:T11)
                    n986 = local write "Input Variables and Slopes"(w2245) -> ()
                    n987 = local write "Groundwater Header"(w2238) -> ()
                  }
                }
                n988 = local write "Initialization"(5 ("Initialization")) -> ()
              }
              frame #5 {
                n989 = flat-sequence {
                  frame #0 {
                    n990 = local read "Input Depths \nand Parameters Cluster"() -> (w2252:T16)
                    n991 = Unbundle By Name(w2252) -> ("Start Depth"=w2249:sgl)
                    n992 = call "prompt_and_enter_value 2016.vi"("prompt_IN"="ENTER START DEPTH", "Enter value"=w2249) -> ("Numeric"=w2254:dbl)  [unwired: 9 in]
                    n993 = Absolute Value(x=w2254) -> (abs(x)=w2253:dbl)
                    n994 = Negate(x=w2253) -> (-x=w2250:dbl)
                    n995 = Bundle By Name(cluster=w2252, "Start Depth"=w2250) -> (w2251:T16)
                    n996 = local write "Input Depths \nand Parameters Cluster"(w2251) -> ()
                  }
                }
                n997 = local write "Initialization"(6 ("Initialization")) -> ()
              }
              frame #6 {
                n998 = local write "Initialization"(7 ("Initialization")) -> ()
                n999 = local read "Input Variables and Slopes"() -> (w2260:T1)
                n1000 = Unbundle By Name(w2260) -> ("Height of Sample Box"=w2258:dbl)
                n1001 = call "prompt_and_enter_value 2016.vi"("prompt_IN"="HEIGHT FROM GROUND SURFACE TO SAMPLE BOX\n\nMeasure the vertical distance between the ground surface and the pressure transducer." ("prompt"), "Enter value"=w2258) -> ("Numeric"=w2257:dbl)  [unwired: 9 in]
                n1002 = Bundle By Name(cluster=w2260, "Height of Sample Box"=w2257) -> (w2259:T1)
                n1003 = global write "Kpro Globals.vi" "height_of_box"(w2257) -> ()
                n1004 = local write "Input Variables and Slopes"(w2259) -> ()
              }
              frame #7 {
                n1005 = local write "Initialization"(8 ("Initialization")) -> ()
                n1006 = flat-sequence {
                  frame #0 {
                    n1007 = local read "Input Variables and Slopes"() -> (w2265:T1)
                    n1008 = Unbundle By Name(w2265) -> ("Depth to Water Table"=w2266:dbl)
                    n1009 = call "prompt_and_enter_value 2016.vi"("prompt_IN"="DEPTH TO WATER TABLE\n\nEnter the depth to the water table." ("prompt"), "Enter value"=w2266) -> ("Numeric"=w2268:dbl)  [unwired: 9 in]
                    n1010 = Absolute Value(x=w2268) -> (abs(x)=w2267:dbl)
                    n1011 = Negate(x=w2267) -> (-x=w2264:dbl)
                    n1012 = global write "Kpro Globals.vi" "Depth to Water Table"(w2264) -> ()
                    n1013 = Bundle By Name(cluster=w2265, "Depth to Water Table"=w2264) -> (w2263:T1)
                    n1014 = local write "Input Variables and Slopes"(w2263) -> ()
                  }
                }
              }
              frame #8 {
                n1015 = stacked-sequence {
                  tunnel: [w2273 _] -> _
                  tunnel: w2271 -> [w2277 w2296]
                  tunnel: w2272 -> [w2276 w2293]
                  tunnel: w2271 -> [_ w2294]
                  frame #0 {
                    # "Set to raw pressure mode"
                    n1016 = local read "Input Variables and Slopes"() -> (w2274:T1)
                    n1017 = local read "Sensor Voltage Cluster"() -> (w2281:T10)
                    n1018 = Unbundle By Name(w2274) -> ("Up Hole Pressure Slope"=w2273:dbl)
                    n1019 = local read "Corrected Pressure Cluster"() -> (w2279:T20)
                    n1020 = call "up hole Pressure 2016.vi"("Sensor Cluster"=w2281, "Pressure Offset"=0.0, "Array in"=w2276, "Pressure \nSlope"=w2273, "Descriptions"=w2277, "Zero Pressure\n(F = leave as is)"=TRUE) -> ("Uphole Pressure"=w2280:dbl)  [unwired: 6 in, 3 out]
                    n1021 = Bundle By Name(cluster=w2279, "Up hole Corrected Pressure"=w2280) -> (w2278:T20)
                    n1022 = local write "Corrected Pressure Cluster"(w2278) -> ()
                    n1023 = local read "Input Variables and Slopes 2"() -> (w2275:T1)
                    n1024 = Unbundle By Name(w2275) -> ()  [unwired: 1 out]
                  }
                  frame #1 {
                    # "adjust for 1 foot head"
                    # "Take offset and put\n into Pressure VI."
                    n1025 = local read "Input Variables and Slopes"() -> (w2288:T1)
                    n1026 = Unbundle By Name(w2288) -> ("Up Hole Pressure Slope"=w2287:dbl)
                    n1027 = local read "Sensor Voltage Cluster"() -> (w2297:T10)
                    n1028 = global read "Kpro Globals.vi" "Pressure Offset"() -> (w2295:dbl)
                    n1029 = local read "Corrected Pressure Cluster"() -> (w2285:T20)
                    n1030 = call "Up Hole PRESSURE_CAL 2016.vi"("Pressure Offset"=w2295, "Descriptions"=w2294, "Array in"=w2293, "Pressure \nSlope"=w2287, "Sensor Cluster"=w2297, "Prompt_IN"="ZERO TO GROUND SURFACE\n\nFill a grad cylinder to 750mL.\nPlace it on the ground at the profile location.\nImmerse the Kpro effluent and turn on Kpro flow.\nTurn off after water is flowing with no bubbles\nand the water has reached 800mL (1 foot).\n\nPress OK when the reading equilibrates." ("message")) -> ("PRESSURE\nFt of water"=w2298:dbl)  [unwired: 4 in, 1 out]
                    n1031 = Decrement(x=w2298) -> (x-1=w2292:dbl)
                    n1032 = call "up hole Pressure 2016.vi"("Sensor Cluster"=w2297, "Pressure Offset"=w2292, "Array in"=w2293, "Pressure \nSlope"=w2287, "Descriptions"=w2296, "Zero Pressure\n(F = leave as is)"=TRUE) -> ("Uphole Pressure"=w2284:dbl, "Pressure Offset 2"=w2289:dbl)  [unwired: 6 in, 2 out]
                    n1033 = Bundle By Name(cluster=w2285, "Up hole Corrected Pressure"=w2284) -> (w2286:T20)
                    n1034 = local read "Input Variables and Slopes"() -> (w2291:T1)
                    n1035 = Bundle By Name(cluster=w2291, "Up Hole  Pressure Offset"=w2289) -> (w2290:T1)
                    n1036 = local write "Input Variables and Slopes"(w2290) -> ()
                    n1037 = local write "Corrected Pressure Cluster"(w2286) -> ()
                  }
                }
                n1038 = local write "Initialization"(9 ("Initialization")) -> ()
              }
              frame #9 {
                n1039 = local write "Initialization"(10 ("Initialization")) -> ()
                n1040 = local read "Cumulative_data_ready"() -> (w2305:bool)
                n1041 = case shown="True" w2305 {
                  tunnel: w2304 -> [w2306 _]
                  tunnel: [w2306 w2307] -> w2303
                  frame False {
                  }
                  frame True {
                    n1042 = local write "Cumulative_data_ready"(FALSE ("Get_KPRO_data")) -> ()
                    n1043 = local read "Cumulative_data_from_file"() -> (w2307:sgl[][])
                  }
                }
              }
            }
            n1044 = flat-sequence {
              tunnel: [w2072] -> _
              frame #0 {
                n1045 = Build Array("Profile ID   " ("string"), "Depth    " ("string"), "Flow " ("string"), "Ik    " ("string")) -> (w2073:string[])
                n1046 = call-poly <vilib>:"Write Delimited Spreadsheet.vi"("file path (dialog if empty)"="Static IK path", "1D data"=w2073, "append to file? (new file:F)"=TRUE, "delimiter (\\t)"="," ("delimiter (\\t)")) -> ("error out"=w2072:errorcluster)  [unwired: 10 in, 1 out]
              }
            }
            n1047 = flat-sequence {
              tunnel: "Read String Pot" -> [_]
              tunnel: [w2346] -> w2050
              tunnel: w2057 -> [w2330]
              tunnel: w2053 -> [w2331]
              frame #0 {
                w2336 = 0.0
                w2337 = TRUE
                # "Initialize Incrementer if using hand incrementer,\nDon't use Debug,\nPut use string pot into shift register first pass to avoid allowing\na change in which method is the source of the depth reading."
                n1048 = global write "Global_SIM_switch.vi" "enable_kpro_file"("enable_kpro_file") -> ()
                n1049 = global write "Global_SIM_switch.vi" "Simulate AD6B"("Simulate AD6B") -> ()
                n1050 = global write "Global_SIM_switch.vi" "enable_slug_file"("enable_slug_file") -> ()
                n1051 = local read "Input Variables and Slopes"() -> (w2344:T1)
                n1052 = global write "Global_SIM_switch.vi" "enable_IKMGS_file"("enable_IKMGS_file") -> ()
                n1053 = Unbundle By Name(w2344) -> ("String Pot Slope"=w2343:dbl, "Up Hole Pressure Slope"=w2339:dbl)  [unwired: 1 out]
                n1054 = local read "Sensor Voltage Cluster"() -> (w2338:T10)
                n1055 = local read "Descriptions"() -> (w2329:string[])
                n1056 = local read "Sensor Voltage Cluster"() -> (w2345:T10)
                n1057 = call "In-Line-Pressure 2016.vi"("Zero Pressure\n(F = leave as is)"=w2337, "In-Line Pressure Slope"=w2339, "Sensor Voltages Cluster"=w2338, "In-Line Pressure Offset"=w2336) -> ("Pressure"=w2340:dbl)  [unwired: 7 in]
                n1058 = call "up hole Pressure 2016.vi"("Sensor Cluster"=w2338, "Pressure Offset"=w2336, "Array in"=w2331, "Pressure \nSlope"=w2339, "Descriptions"=w2329, "Zero Pressure\n(F = leave as is)"=w2337) -> ("Array out"=w2328:refnum<k24>[], "Uphole Pressure"=w2325:dbl)  [unwired: 6 in, 2 out]
                n1059 = Bundle By Name(cluster="Corrected Pressure Cluster", "Up hole Corrected Pressure"=w2325, "Down hole Corrected Pressure"=w2340) -> (w2341:T20)
                n1060 = call "depth read from string pot 2016.vi"("Descriptions"=w2329, "error in (no error)"=w2330, "String Pot \nSlope"=w2343, "Array in"=w2328, "Sensor Cluster In"=w2345) -> ("Depth"=w2347:dbl)  [unwired: 11 in, 3 out]
                n1061 = local read "Sample Sheet Data Row Cluster 2"() -> (w2327:T3)
                n1062 = local write "Corrected Pressure Cluster"(w2341) -> ()
                n1063 = flat-sequence {
                  tunnel: w2347 -> [w2349]
                  tunnel: [w2348] -> w2346
                  frame #0 {
                    w2350 = 15  # Filter Size
                    # "Functional Global in \nBoxcar Integrator\nInitialize filter array to \ncurrent string pot value"
                    n1064 = call "Boxcar filter2016.vi"("Initialize"=TRUE, "Filter Size"=w2350, "Filter Input"=w2349) -> ("Filter Output"=w2348:dbl)
                  }
                }
                n1065 = Bundle By Name(cluster=w2327, "Head\nPressure"=w2325) -> (w2326:T3)
                n1066 = local write "Sample Sheet Data Row Cluster 2"(w2326) -> ()
              }
            }
            n1067 = flat-sequence {
              tunnel: [w2312] -> w2058
              tunnel: [w2311] -> w2051
              tunnel: w2050 -> [w2309]
              tunnel: [w2309] -> w2047
              frame #0 {
                n1068 = local read "Input Depths \nand Parameters Cluster"() -> (w2310:T16)
                n1069 = Unbundle By Name(w2310) -> ("Start Depth"=w2313:sgl)
                n1070 = Less Or Equal To 0?(x=w2313) -> (x <= 0?=w2315:bool)
                n1071 = Negate(x=w2313) -> (-x=w2314:sgl)
                n1072 = Select(t=w2313, s=w2315, f=w2314) -> (s? t:f=w2311:sgl)
                n1073 = Bundle By Name(cluster=w2310, "Abs Start Depth"=w2311, "Current Depth"=w2309) -> (w2312:T16)
                n1074 = local write "Input Depths \nand Parameters Cluster"(w2312) -> ()
              }
            }
            n1075 = flat-sequence {
              tunnel: [w2322] -> w2060
              frame #0 {
                n1076 = Tick Count (ms)() -> (millisecond timer value=w2324:u32)
                n1077 = Divide(x=w2324, y=u32 1000) -> (x/y=w2322:dbl)
              }
            }
            n1078 = flat-sequence {
              tunnel: [w2317] -> w2059
              tunnel: w2060 -> [w2320]
              tunnel: [w2319] -> _
              tunnel: w2051 -> [w2319]
              tunnel: w2047 -> [w2318]
              tunnel: w2044 -> [w2316]
              frame #0 {
                n1079 = Bundle By Name(cluster=w2316, "Absolute Depth In"=w2319, "Previous Relative Depth"=w2318, "Current Relative Depth"=w2318, "First Relative Depth"=w2318, "Current Absolute Depth"=w2319, "Last Filed Depth"=0.0, "Current Measurement Time"=w2320, "Previous Measurement Time"=w2320, "First Absolute Depth"=w2319) -> (w2317:T17)
              }
            }
          }
          frame "Acq. DAQ data" {
            n1080 = flat-sequence {
              tunnel: w2400 -> [w2417]
              tunnel: w2399 -> [w2416]
              tunnel: [w2413] -> w2398
              frame #0 {
                n1081 = local read "Descriptions"() -> (w2414:string[])
                n1082 = local read "Sensor  Real \nMeasurements"() -> (w2412:T7)
                n1083 = local read "Input Variables and Slopes"() -> (w2410:T1)
                n1084 = call "Measure DAQ Voltages.vi"("error in (no error)"=w2416, "Descriptions"=w2414, "Array in"=w2417) -> ("Raw Voltages"=→"Raw Voltages":dbl[], "Array out"=w2413:refnum<k24>[], "Sensor Cluster"=w2409:T10)  [unwired: 6 in]
                "Sensor Voltage Cluster" <- w2409
                n1085 = call "convert sensor voltage to real measurements.vi"("Input Variables and Slopes"=w2410, "Sensor  Real Measurements in"=w2412, "Sensor Cluster"=w2409) -> ("Sensor  Real Measurements out"=w2411:T10)  [unwired: 8 in]
                n1086 = local write "Sensor  Real \nMeasurements"(w2411) -> ()
              }
            }
          }
          frame "Exit" {
            n1087 = flat-sequence {
              tunnel: [w2445] -> _
              tunnel: [w2452] -> w2422
              tunnel: w2425 -> [w2447]
              tunnel: w2424 -> [w2445]
              tunnel: [w2444] -> w2423
              frame #0 {
                w2451 = "Groundwater Profile Log" ("Worksheet Name in")
                n1088 = local read "Worksheet Names"() -> (w2449:string[])
                n1089 = local write "Current Sample Sheet"(w2451) -> ()
                n1090 = call "find and open select worksheet.vi"("Worksheet Names"=w2449, "error in (no error)"=w2445, "milliseconds to wait"=u32 100, "Worksheet Name in"=w2451, "NI_report in"=w2447) -> ("error out"=w2448:errorcluster, "NI_report out"=w2446:refnum<class "NI_report.lvclass">)  [unwired: 4 in, 1 out]
                n1091 = call "groundwater log header.vi"("Worksheet Names"=w2449, "Groundwater Header"="Groundwater Header", "error in (no error)"=w2448, "NI_report in"=w2446) -> ("error out"=w2444:errorcluster, "NI_report out"=w2452:refnum<class "NI_report.lvclass">)  [unwired: 6 in]
              }
            }
            n1092 = case shown="No Error" w2433 {
              tunnel: w2429 -> [w2476 _]
              tunnel: w2433 -> [w2475 w2487]
              tunnel: [w2474 w2487] -> w2431
              frame No Error {
                n1093 = for {
                  shift-right: [w2478] -> w2474
                  shift-left: w2475 -> [w2479]
                  tunnel: w2476 -> [w2477] mode=indexing
                  n1094 = while {
                    shift-right: [w2486] -> w2481
                    shift-left: w2479 -> [w2484]
                    shift-right: [w2485] -> w2480
                    shift-left: w2477 -> [w2483]
                    stop <- w2482 stop-if-true
                    n1095 = call <vilib>:"ULx Is Task Done.vi"("task in"=w2483, "error in"=w2484) -> ("task out"=w2485:refnum<k24>, "task done?"=w2482:bool, "error out"=w2486:errorcluster)  [unwired: 11 in]
                  }
                  n1096 = call <vilib>:"ULx Clear Task.vi"("task in"=w2480, "error in"=w2481) -> ("error out"=w2478:errorcluster)  [unwired: 13 in]
                }
              }
              frame Error {
              }
            }
            n1097 = flat-sequence {
              tunnel: [w2493] -> w2440
              tunnel: [w2492] -> w2441
              tunnel: w2423 -> [w2490]
              tunnel: w2422 -> [w2489]
              frame #0 {
                n1098 = local read "Excel report file path"() -> (w2488:path)
                n1099 = call-dynamic "Save Report to File.vi"("report in"=w2489, "report file path"=w2488, "prompt to replace? (F)"=FALSE, "error in (no error)"=w2490) -> ("report out"=w2493:refnum<class "NI_report.lvclass">, "error out"=w2492:errorcluster)  [unwired: 10 in]
              }
            }
            n1100 = call <userlib>:"Wait (ms)__ogtk.vi"("error in (no error)"=w2441, "milliseconds to wait"=u32 5) -> ("error out"=w2442:errorcluster)  [unwired: 8 in, 1 out]
            n1101 = flat-sequence {
              tunnel: w2442 -> [w2462]
              tunnel: w2440 -> [w2460]
              tunnel: [w2458] -> w2434
              frame #0 {
                (unwired) FALSE ("Write Ini")
                n1102 = call-dynamic "Dispose Report.vi"("report in"=w2460, "save changes? (F)"=FALSE, "error in (no error)"=w2462) -> ("error out"=w2457:errorcluster)  [unwired: 12 in]
                n1103 = case shown="False" "Save Configuration File?" {
                  tunnel: [errorcluster {"status"=FALSE, "code"=0, "source"=""} ("error IO") w2471] -> w2459
                  frame False {
                  }
                  frame True {
                    n1104 = local read "Config File Path"() -> (w2470:path)
                    n1105 = call <vilib>:"Open Config Data.vi"("create file if necessary (T)"=TRUE ("Read Ini"), "configuration file path"=w2470) -> ("error out"=w2468:errorcluster, "refnum"=w2465:T21)  [unwired: 7 in, 1 out]
                    n1106 = control-ref of="This VI"() -> (w2464:refnum<vi>)
                    n1107 = call <userlib>:"Write Panel to INI__ogtk.vi"("error in (no error)"=w2468, "VI ref"=w2464, "refnum"=w2465) -> ("error out"=w2467:errorcluster, "refnum out"=w2466:T21)  [unwired: 7 in]
                    n1108 = call <vilib>:"Clear Errors.vi"("error in (no error)"=w2467) -> ("error out"=w2473:errorcluster)  [unwired: 5 in, 1 out]
                    n1109 = call <vilib>:"Close Config Data.vi"("error in (no error)"=w2473, "refnum"=w2466) -> ("error out"=w2472:errorcluster)  [unwired: 8 in, 1 out]
                    n1110 = Merge Errors(w2472, w2467) -> (w2471:errorcluster)
                  }
                }
                n1111 = Merge Errors(w2459, w2457) -> (w2458:errorcluster)
              }
            }
            n1112 = flat-sequence {
              tunnel: [TRUE ("aborted?")] -> w2432
              tunnel: [w2454] -> w2430
              tunnel: w2431 -> [w2454]
              frame #0 {
              }
            }
          }
        }
        n1113 = local write "Depth Cluster"(w429) -> ()
      }
    }
  }
  n1114 = invoke on="IK Reason array" class="Arr (strict)" method="Reinit To Default"() -> ()  [unwired: 3 in, 3 out]
  n1115 = invoke on="Recording Reason Sonde array" class="Arr (strict)" method="Reinit To Default"() -> ()  [unwired: 3 in, 3 out]
  n1116 = Merge Errors(w17, w16) -> (→"error out":errorcluster)
